vi "MainKinetics.vi"() -> ()   [LabVIEW 2017]
uses:
  <vilib>/Utility/miscctls.llb/LVRowAndColumnTypeDef.ctl
  <vilib>/Utility/sysdir.llb/System Directory Type.ctl
  <vilib>/Utility/config.llb/Read Key (String).vi
  <vilib>/Utility/config.llb/Write Key (String).vi
  <vilib>/Utility/cursorutil.llb/Set Cursor (Icon Pict).vi
  PCAN_Driver/ControlCAN.lvlib
  <vilib>/Utility/config.llb/NI_LVConfig.lvlib
panel:
  out "Offset":dbl
  out "Analogtest":bool=TRUE
  out "TestinExecution":string
  out "FullSpeed2 Current":dbl
  out "FullSpeed1 Current":dbl
  out "String":string
  out "ParamVersion":string
  out "DSP Board S/N":string
  out "POWER Board S/N":string caption="DRIVER Board S/N"
  in  "EventTimeout":i32=100
  out "SpeedLimit":dbl[](array[numeric])
  out "TestArray":string[](array[string])
  out "Motor Speed RPM Serial":dbl
  out "DAQmx Device Name":tag
  out "PN":string
  out "FileName":string
  out "VenableSpeed":u16
  out "TesterVersion":string
  out "ClosePanel":bool=TRUE
  out "UUT SN Report":string
  out "Automation":bool
  out "Test Failed":bool
  out "VisualInspectionResult":bool
  out "MotorTempResult":bool
  out "VenableDirectionResult":bool
  out "VenableResult":bool
  out "ComTestResult":bool=TRUE
  out "UUT SoftwareVer":string
  out "Next SN":i32
  in  "SetSN":bool
  out "Current SN":i32
  out "FullSpeed2 Speed":dbl
  out "FullSpeed2 Current":dbl
  out "FullSpeed1 Current":dbl
  out "FullSpeed1 Speed":dbl
  out "UUT":u8
  out "CAN Status":bool
  out "Array":u64[][](array[numeric]) format="%016x"
  out "Motor Phase Current RMS":dbl
  out "Ambient Temperature":dbl
  out "Speed error":bool
  out "Commutation err":bool
  out "Under voltage/Over voltage":bool
  out "Derated drive temp":bool
  out "Motor Over temperature":bool
  out "Motor Sensor temp Fauilre":bool
  out "Drive Over temperature":bool
  out "Drive Sensor temp Failure":bool
  out "Ambient Over temp":bool
  out "Ambient Sensor temp":bool
  out "DC Voltage":dbl
  out "DC Current":dbl
  out "Power transistor Heat sink Temp.":dbl
  out "Motor Stator Temp.":dbl
  out "Motor Speed RPM":dbl
  out "ECS State":u16
  out "UUT":string="EBAY"
  in  "Logger Path":path
  in  "Report":bool
  in  "Start":bool
  in  "ATR":string[][](table)=[["Test Communication", "-", "-", "-", "-", ""], ["Set S/N", "-", "-", "-", "-", ""], ["Set Board Number", "-", "-", "-", "-", ""], [" ", "", "", "", "", ""], ["Test Communication", "-", "-", "-", "-", ""], ["Get S/N", "-", "-", "-", "", ""], ["Get Board Number", "-", "-", "-", "", ""], ["Get FW", "-", "-", "-", "", ""], ["Enable Motor", "", "", "", "", ""], ["Small position command", "", "", "", "", ""], ["Measure delta", "", "", "", "", ""], ["Velocity command", "", "", "", "", ""]]
  in  "Settings":bool
  in  "Refresh Button":bool
  out "Serial Status":bool
  in  "VISA Kinetics":refnum<visa-resource-name>="COM6"
  in  "Serial Com":bool
  in  "Help Button":bool
  out "Pannel User Message":string
  in  "Stop Button":bool
  # "Kinetics"
  # "REDLER TECHNOLOGIES LTD"
  # "ver 1.2p"
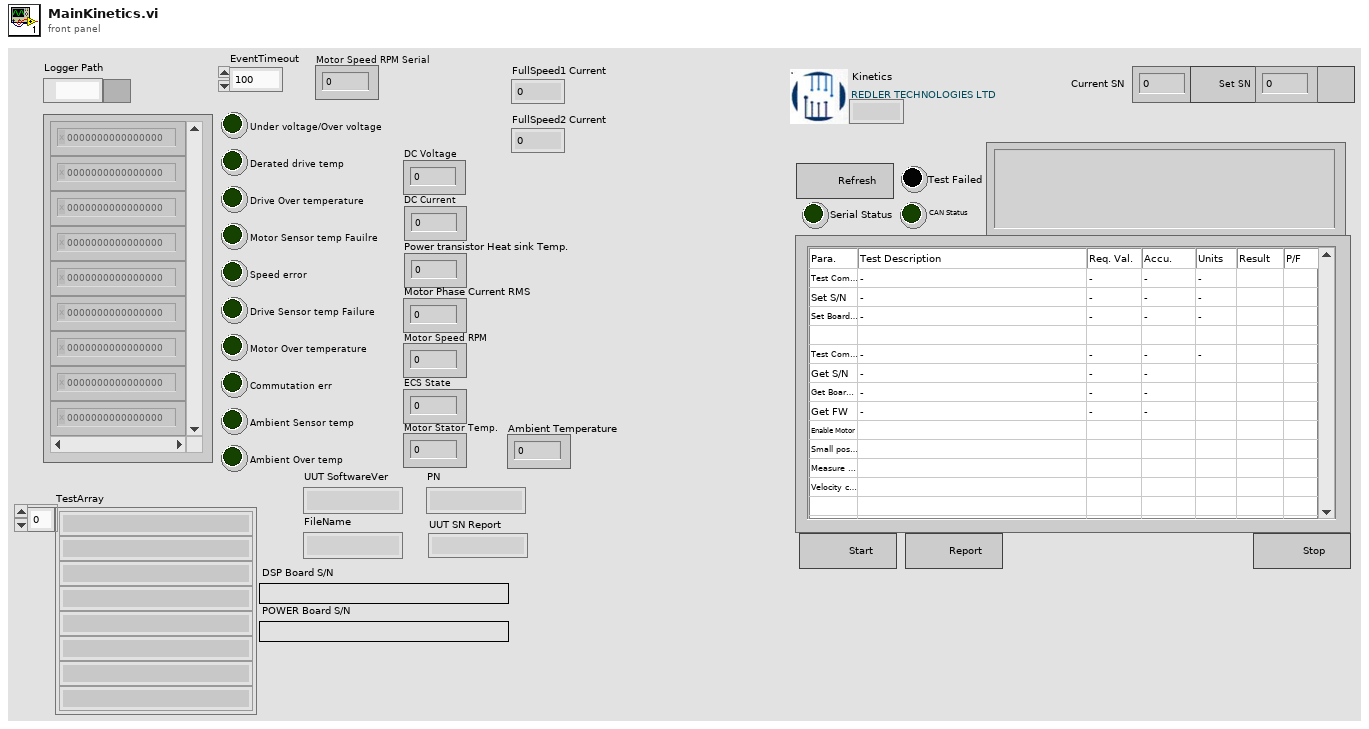
[diagram p1: front panel]
types:
  T1 = cluster{"VISA":refnum<visa-resource-name>, "TestArray":string[]}
  T2 = cluster{"ID":u32, "MSGTYPE":u8, "LEN":u8, "aDATA":u8[]}[]
  T3 = enum16{"Erase ATR Table", "Stop", "MainProgram", "Initialize"}
  T4 = typedef "NI_LVConfig.lvlib/Config Data RefNum.ctl" = refnum<k1>
  T5 = enum16{"Init", "0 ohm", "6 ohm", "13.2 ohm", "15 ohm", "25.9 ohm", "33 ohm", "Down", "Up", "Venable", "Firmware", "PowerSuply"}
  T6 = enum16{"Wait", "Exit", "VC=0", "ReadVC", "VC=1000"}
  T7 = enum16{"Stop", "Result", "FullSpeed2", "MD[1]=1", "FullSpeed1", "MD[1]=0"}
  T8 = enum16{"K15", "K16", "K17", "Venable", "Firmeware", "Fan", "Power", "120C", "110C", "100C", "90C", "80C", "70C", "60C", "50C", "40C", "30C", "25C", "20C", "10C", "0C"}
  T9 = enum8{"Term1", "Term2", "Current", "Fan", "TempCPU"}
  T10 = enum16{"Exit", "AI0/3", "AO0", "Wait", "Read", "Init"}
  T11 = enum16{"Exit", "Wait", "ReadCurrent", "ReadTemp", "Init"}
  T12 = enum16{"Init", "0 ohm", "6 ohm", "13.2 ohm", "15 ohm", "25.9 ohm", "33 ohm", "Down", "Up", "Venable", "Firmware", "PowerSuply"}[]
  T13 = enum8{"Enabled", "Disabled", "Disabled and Grayed Out"}
  T14 = typedef "LVRowAndColumnTypeDef.ctl" = cluster{"Row":i32, "Column":i32}
  T15 = enum32{"Invalid", "Standard", "Closed", "Hidden", "Minimized", "Maximized"}
  T16 = cluster{"ID":u32, "MSGTYPE":u8, "LEN":u8, "aDATA":u8[]}
  T17 = enum16{"open", "replace", "create", "open or create", "replace or create", "replace or create with confirmation"}
  T18 = typedef "ControlCAN.lvlib/DevType.ctl" = u32
  T19 = typedef "ControlCAN.lvlib/CAN Channel.ctl" = u32
  T20 = typedef "ControlCAN.lvlib/VCI_INIT_CONFIG.ctl" = cluster{"AccCode":u32, "AccMask":u32, "InitFlag":T21, "Fliter":T22, "Timing0":u8, "Timing1":u8, "Mode":T23}
  T21 = typedef "ControlCAN.lvlib/InitFlag.ctl" = u32
  T22 = typedef "ControlCAN.lvlib/Fliter.ctl" = u8
  T23 = typedef "ControlCAN.lvlib/Mode.ctl" = u8
  T24 = cluster{"DevType":T18, "DevIndex":u32, "CanIndex":T19, "VCI_INIT_CONFIG":T20}
  T25 = typedef "ControlCAN.lvlib/VCI_CAN_OBJ.ctl" = cluster{"ID":u32, "TimeStamp":u32, "TimeFlag":u8, "SendType":u8, "RemoteFlag":u8, "ExternFlag":u8, "DataLen":u8, "Data":u8[], "Reserved":u8[]}
  T26 = cluster{"Type":enum16{"接收", "发送"}, "Channel":T19, "Time":timestamp, "VCI_CAN_OBJ":T25}[]
  T27 = cluster{"Type":enum16{"接收", "发送"}, "Channel":T19, "Time":timestamp, "VCI_CAN_OBJ":T25}
  T28 = typedef "LVPoint32TypeDef.ctl" = cluster{"Horizontal":i32, "Vertical":i32}
  T29 = typedef "System Directory Type.ctl" = i32
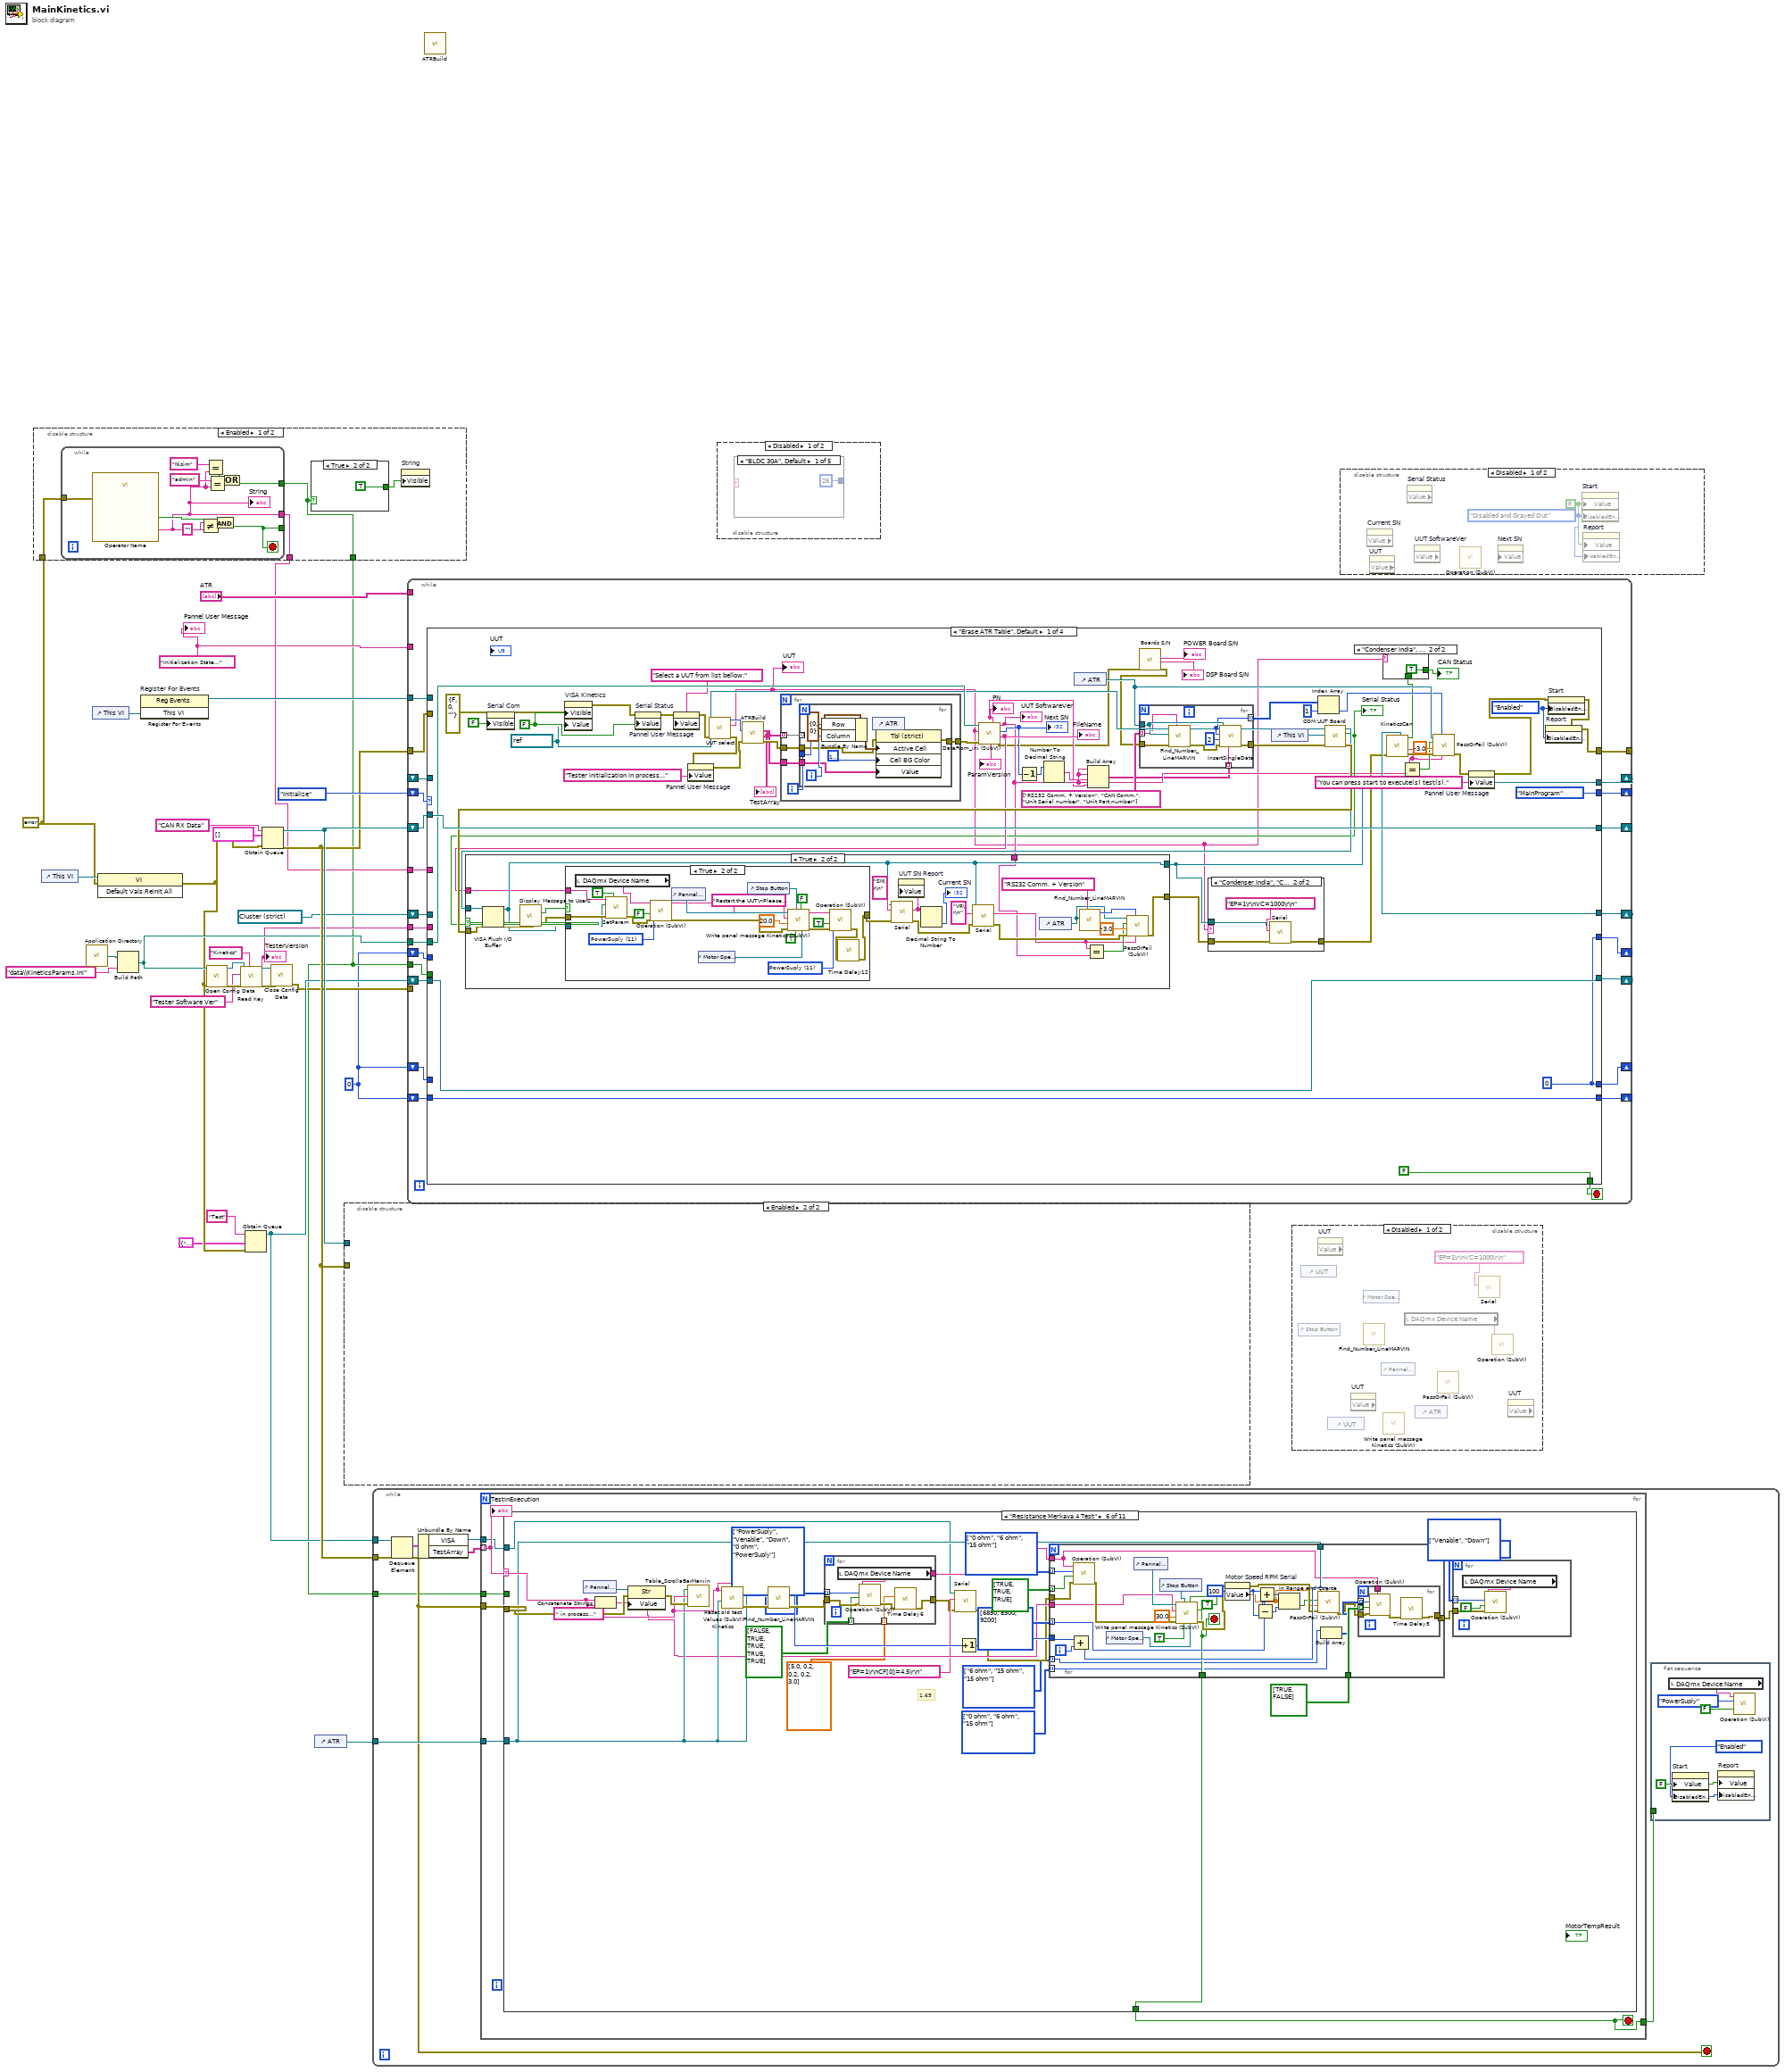
[diagram p0: block diagram]
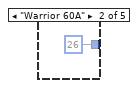
[diagram p2: hidden frame]
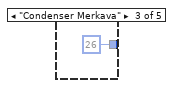
[diagram p3: hidden frame]
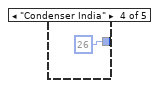
[diagram p4: hidden frame]
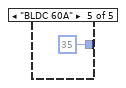
[diagram p5: hidden frame]
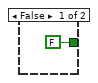
[diagram p7: hidden frame]
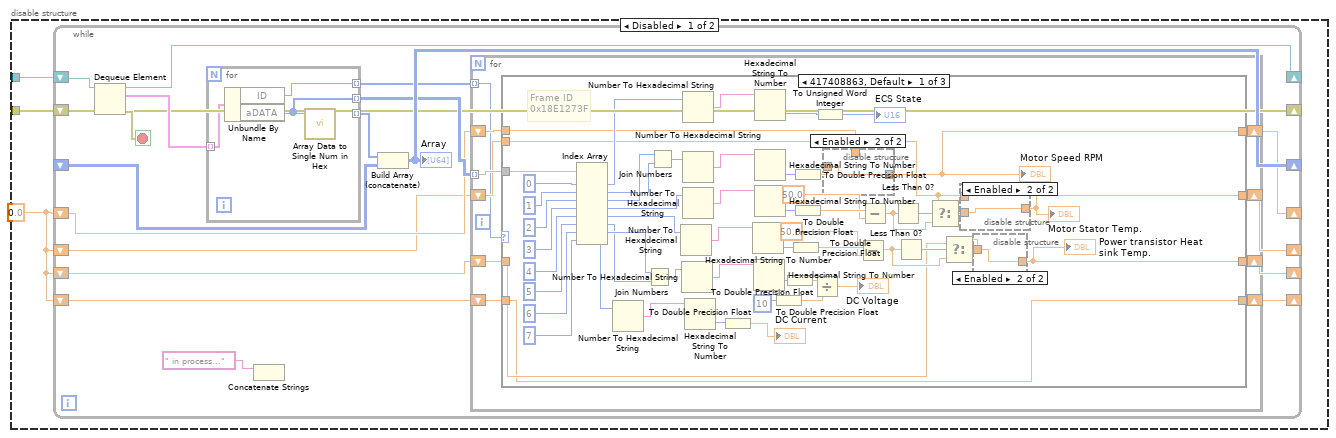
[diagram p9: hidden frame]
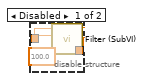
[diagram p10: hidden frame]
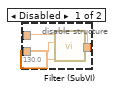
[diagram p11: hidden frame]
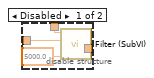
[diagram p12: hidden frame]
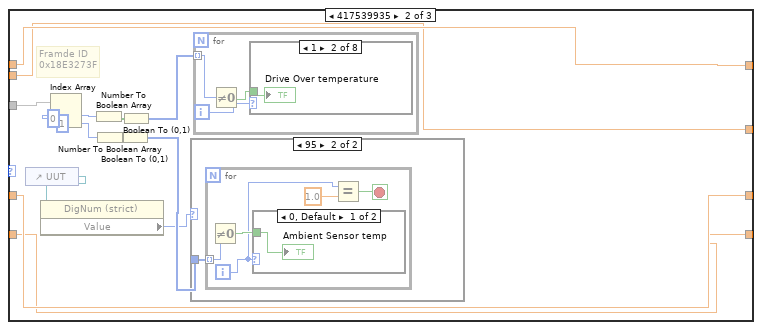
[diagram p13: hidden frame]
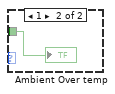
[diagram p15: hidden frame]
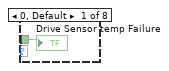
[diagram p16: hidden frame]
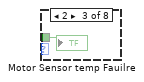
[diagram p17: hidden frame]
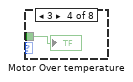
[diagram p18: hidden frame]
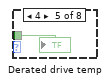
[diagram p19: hidden frame]
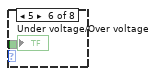
[diagram p20: hidden frame]
diagram:
  w17 = "Initialization State..."
  w2 = 0
  w5 = errorcluster {"status"=FALSE, "code"=0, "source"=""} ("error in (no error)")
  n1 = disable-structure shown="Enabled" {
    disable-tunnel: [w35 _] -> w18
    disable-tunnel: w5 -> [w33 _]
    disable-tunnel: [w32 _] -> w3
    frame Enabled {
      n2 = while {
        tunnel: [w45] -> _
        tunnel: [w38] -> w35
        tunnel: [w42] -> w32
        tunnel: w33 -> [w39]
        stop <- w45 stop-if-true
        n3 = call "Operator Name"("error in (no error)"=w39) -> ("Operator Name"=w38:string, "OK"=w46:bool)  [unwired: 16 in, 1 out]
        "String" <- w38
        n4 = Not Equal?(x=w38, y="") -> (x != y?=w47:bool)
        n5 = Equal?(x="Nisim", y=w38) -> (x = y?=w40:bool)
        n6 = Equal?(x="admin", y=w38) -> (x = y?=w43:bool)
        n7 = And(x=w46, y=w47) -> (x .and. y?=w45:bool)
        n8 = Or(x=w40, y=w43) -> (x .or. y?=w42:bool)
      }
      n9 = case shown="True" w32 {
        tunnel: [FALSE TRUE] -> w34
        frame False {
        }
        frame True {
        }
      }
      n10 = property on="String" class="Str"("Visible"=w34) -> ()  [unwired: 2 in, 2 out]
    }
    frame Disabled {
    }
  }
  n11 = control-ref of="This VI"() -> (w6:refnum<vi>)
  n12 = call <vilib>:"Application Directory.vi"() -> ("Application Directory"=w22:path)
  n13 = control-ref of="This VI"() -> (w20:refnum<vi>)
  n14 = invoke class="VI" method="Default Vals.Reinit All"(reference=w6, error in=w5) -> (error out=w4:errorcluster)  [unwired: 1 in, 2 out]
  n15 = Build Path(base path=w22, name or relative path="data\\KineticsParams.ini") -> (appended path=w9:path)
  n16 = register-events "Register For Events"(w20) -> (reference out=w19:refnum<event-registration>)  [unwired: 2 in, 1 out]
  n17 = call <vilib>:"Open Config Data.vi"("error in (no error)"=w4, "configuration file path"=w9) -> ("error out"=w15:errorcluster, "refnum"=w14:T4)  [unwired: 1 in, 7 out]
  n18 = call-poly <vilib>:"Read Key.vi"("section"="Kinetics", "error in (no error)"=w15, "key"="Tester Software Ver", "refnum"=w14) -> ("error out"=w12:errorcluster, "value"=w7:string, "refnum out"=w11:T4)  [unwired: 2 in, 3 out]
  "TesterVersion" <- w7
  n19 = Obtain Queue(name (unnamed)="Test", element data type=T1 {"VISA"="COM1", "TestArray"=[]}, error in (no error)=w4) -> (queue out=w25:refnum<queue>)  [unwired: 2 in, 2 out]
  n20 = Obtain Queue(name (unnamed)="CAN RX Data", element data type=T2 [], error in (no error)=w4) -> (queue out=w28:refnum<queue>, error out=w26:errorcluster)  [unwired: 2 in, 1 out]
  n21 = call <vilib>:"Close Config Data.vi"("error in (no error)"=w12, "refnum"=w11) -> ("error out"=w10:errorcluster)  [unwired: 8 in, 1 out]
  n22 = control-ref of="ATR"() -> (w16:refnum<vi>)
  n23 = disable-structure shown="Enabled" {
    disable-tunnel: w28 -> [w51 _]
    disable-tunnel: w26 -> [w50 _]
    frame Disabled {
      w49 = 0.0
      n24 = while {
        shift-right: [w68] -> _
        shift-left: w51 -> [w70]
        shift-right: [w66] -> _
        shift-left: _ -> [w67]
        shift-right: [w62] -> _
        shift-left: w50 -> [w62]
        shift-right: [w60] -> _
        shift-left: w49 -> [w61]
        shift-right: [w59] -> _
        shift-left: w49 -> [w58]
        shift-right: [w57] -> _
        shift-left: w49 -> [w56]
        shift-right: [w55] -> _
        shift-left: w49 -> [w54]
        stop <- w69 stop-if-true
        n25 = Dequeue Element(queue=w70, error in (no error)=w62) -> (queue out=w68:refnum<queue>, element=w63:T2, error out=w69:errorcluster)  [unwired: 1 in, 1 out]
        n26 = for {
          tunnel: [w216] -> w65 mode=indexing
          tunnel: w63 -> [w215] mode=indexing
          tunnel: [w214] -> w64 mode=indexing
          tunnel: [w213] -> w53 mode=indexing
          n27 = Unbundle By Name(w215) -> ("ID"=w213:u32, "aDATA"=w214:u8[])
          n28 = call "Array Data to Single Num in Hex.vi"("aDATA"=w214) -> ("Numeric"=w216:u64)  [unwired: 10 in]
        }
        n29 = Concatenate Strings(" in process..." ("Strin")) -> ()  [unwired: 1 in, 1 out]
        n30 = Build Array (concatenate)(w65, w67) -> (w66:u64[][])
        "Array" <- w66
        n31 = for {
          tunnel: w64 -> [w80] mode=indexing
          shift-right: [w78] -> w60
          shift-left: w61 -> [w79]
          shift-right: [w77] -> w59
          shift-left: w58 -> [w76]
          shift-right: [w75] -> w57
          shift-left: w56 -> [w74]
          shift-right: [w73] -> w55
          shift-left: w54 -> [w72]
          tunnel: w53 -> [w71] mode=indexing
          n32 = case shown="417408863, Default" w71 {
            tunnel: w80 -> [w117 w165 w203]
            tunnel: w79 -> [w91 w154 w192]
            tunnel: [w90 w154 w192] -> w78
            tunnel: [w87 w153 w191] -> w77
            tunnel: w76 -> [w86 w153 w191]
            tunnel: [w83 w152 w190] -> w75
            tunnel: w74 -> [w82 w152 w190]
            tunnel: [w81 w151 w186] -> w73
            tunnel: w72 -> [w81 w151 w185]
            frame 417408863, Default {
              # "Frame ID\n0x18E1273F"
              n33 = Index Array(array=w117, index #1=0 ("index"), index #2=1 ("index"), index #3=2 ("index"), index #4=3 ("index"), index #5=4 ("index"), index #6=5 ("index"), index #7=6 ("index"), index #8=7 ("index")) -> (element #1=w101:u8, element #2=w103:u8, element #3=w104:u8, element #4=w108:u8, element #5=w111:u8, element #6=w115:u8, element #7=w116:u8, element #8=w114:u8)
              n34 = Number To Hexadecimal String(2:w114) -> (0:w128:string)  [unwired: 1 in]
              n35 = Join Numbers(hi=w116, lo=w115) -> ((hi.lo)=w135:u16)
              n36 = Join Numbers(hi=w104, lo=w103) -> ((hi.lo)=w105:u16)
              n37 = Number To Hexadecimal String(2:w111) -> (0:w112:string)  [unwired: 1 in]
              n38 = Number To Hexadecimal String(2:w135) -> (0:w134:string)  [unwired: 1 in]
              n39 = Number To Hexadecimal String(2:w101) -> (0:w102:string)  [unwired: 1 in]
              n40 = Number To Hexadecimal String(2:w105) -> (0:w106:string)  [unwired: 1 in]
              n41 = Number To Hexadecimal String(2:w108) -> (0:w109:string)  [unwired: 1 in]
              n42 = Hexadecimal String To Number(string=w128) -> (number=w127:u32)  [unwired: 2 in, 1 out]
              n43 = To Double Precision Float(number=w127) -> (double precision float=→"DC Current":dbl)
              n44 = Hexadecimal String To Number(string=w112) -> (number=w113:u32)  [unwired: 2 in, 1 out]
              n45 = Hexadecimal String To Number(string=w134) -> (number=w133:u32)  [unwired: 2 in, 1 out]
              n46 = Hexadecimal String To Number(string=w102) -> (number=w99:u32)  [unwired: 2 in, 1 out]
              n47 = Hexadecimal String To Number(string=w106) -> (number=w107:u32)  [unwired: 2 in, 1 out]
              n48 = Hexadecimal String To Number(string=w109) -> (number=w110:u32)  [unwired: 2 in, 1 out]
              n49 = To Double Precision Float(number=u32 10 ("y")) -> (double precision float=w131:dbl)
              n50 = To Double Precision Float(number=w133) -> (double precision float=w130:dbl)
              n51 = To Double Precision Float(number=w113) -> (double precision float=w96:dbl)
              n52 = To Double Precision Float(number=w107) -> (double precision float=w92:dbl)
              n53 = To Double Precision Float(number=w110) -> (double precision float=w98:dbl)
              n54 = Divide(x=w130, y=w131) -> (x/y=→"DC Voltage":dbl)
              n55 = To Unsigned Word Integer(number=w99) -> (unsigned 16bit integer=→"ECS State":u16)
              n56 = disable-structure shown="Enabled" {
                disable-tunnel: w92 -> [w149 w150]
                disable-tunnel: w91 -> [w148 _]
                disable-tunnel: [w146 w150] -> w90
                frame Disabled {
                  n57 = call "Filter (SubVI).vi"("Delta"=5000.0, "NewVal"=w149, "OldVal"=w148) -> ("Val"=w146:dbl)  [unwired: 8 in]
                }
                frame Enabled {
                }
              }
              "Motor Speed RPM" <- w90
              n58 = Subtract(x=w96, y=50.0 ("x")) -> (x-y=w85:dbl)
              n59 = Subtract(x=w98, y=50.0 ("x")) -> (x-y=w88:dbl)
              n60 = Less Than 0?(x=w88) -> (x < 0?=w94:bool)
              n61 = Less Than 0?(x=w85) -> (x < 0?=w93:bool)
              n62 = Select(t=w86, s=w94, f=w88) -> (s? t:f=w89:dbl)
              n63 = Select(t=w82, s=w93, f=w85) -> (s? t:f=w84:dbl)
              n64 = disable-structure shown="Enabled" {
                disable-tunnel: w89 -> [w144 w145]
                disable-tunnel: [w143 w145] -> w87
                disable-tunnel: w86 -> [w142 _]
                frame Disabled {
                  n65 = call "Filter (SubVI).vi"("Delta"=130.0, "NewVal"=w144, "OldVal"=w142) -> ("Val"=w143:dbl)  [unwired: 8 in]
                }
                frame Enabled {
                }
              }
              "Motor Stator Temp." <- w87
              n66 = disable-structure shown="Enabled" {
                disable-tunnel: w84 -> [w139 w140]
                disable-tunnel: [w137 w140] -> w83
                disable-tunnel: w82 -> [w136 _]
                frame Disabled {
                  n67 = call "Filter (SubVI).vi"("Delta"=100.0, "NewVal"=w139, "OldVal"=w136) -> ("Val"=w137:dbl)  [unwired: 8 in]
                }
                frame Enabled {
                }
              }
              "Power transistor Heat sink Temp." <- w83
            }
            frame 417539935 {
              # "Framde ID\n0x18E3273F"
              n68 = control-ref of="UUT"() -> (w155:refnum<vi>)
              n69 = property on="Property Node" class="DigNum (strict)"(reference=w155) -> ("Value"=w156:u8)  [unwired: 1 in, 2 out]
              n70 = Index Array(array=w165, index #1=0 ("index"), index #2=1 ("index")) -> (element #1=w163:u8, element #2=w158:u8)
              n71 = Number To Boolean Array(number=w163) -> (Boolean array=w162:bool[])
              n72 = Number To Boolean Array(number=w158) -> (Boolean array=w160:bool[])
              n73 = Boolean To (0,1)(Boolean=w160) -> (0, 1=w157:i16[])
              n74 = Boolean To (0,1)(Boolean=w162) -> (0, 1=w161:i16[])
              n75 = case shown="95" w156 {
                tunnel: w157 -> [_ w166]
                frame 0, Default {
                }
                frame 95 {
                  n76 = for {
                    tunnel: w166 -> [w171] mode=indexing
                    i -> [w167]
                    stop <- w169 stop-if-true
                    n77 = Not Equal To 0?(x=w171) -> (x != 0?=w170:bool)
                    n78 = case shown="0, Default" w167 {
                      tunnel: w170 -> [w172 w173]
                      frame 0, Default {
                        "Ambient Sensor temp" <- w172
                      }
                      frame 1 {
                        "Ambient Over temp" <- w173
                      }
                    }
                    n79 = Equal?(x=w167, y=1.0) -> (x = y?=w169:bool)
                  }
                }
              }
              n80 = for {
                tunnel: w161 -> [w175] mode=indexing
                i -> [w176]
                n81 = Not Equal To 0?(x=w175) -> (x != 0?=w174:bool)
                n82 = case shown="1" w176 {
                  tunnel: w174 -> [w177 w178 w179 w180 w181 w182 w183 w184]
                  frame 0, Default {
                    "Drive Sensor temp Failure" <- w177
                  }
                  frame 1 {
                    "Drive Over temperature" <- w178
                  }
                  frame 2 {
                    "Motor Sensor temp Fauilre" <- w179
                  }
                  frame 3 {
                    "Motor Over temperature" <- w180
                  }
                  frame 4 {
                    "Derated drive temp" <- w181
                  }
                  frame 5 {
                    "Under voltage/Over voltage" <- w182
                  }
                  frame 6 {
                    "Commutation err" <- w183
                  }
                  frame 7 {
                    "Speed error" <- w184
                  }
                }
              }
            }
            frame 417474399 {
              # "Frame ID\n0x18E2273F"
              n83 = Index Array(array=w203, index #1=0 ("index"), index #2=1 ("index")) -> (element #1=w200:u8, element #2=w197:u8)
              n84 = disable-structure shown="Enabled" {
                disable-tunnel: [w211 w212] -> w201
                disable-tunnel: w200 -> [w210 w212]
                frame Disabled {
                  n85 = Number To Hexadecimal String(2:w210) -> (0:w209:string)  [unwired: 1 in]
                  n86 = Hexadecimal String To Number(string=w209) -> (number=w211:u32)  [unwired: 2 in, 1 out]
                }
                frame Enabled {
                }
              }
              n87 = Number To Hexadecimal String(2:w197) -> (0:w195:string)  [unwired: 1 in]
              n88 = Hexadecimal String To Number(string=w195) -> (number=w196:u32)  [unwired: 2 in, 1 out]
              n89 = To Double Precision Float(number=w196) -> (double precision float=w194:dbl)
              n90 = To Double Precision Float(number=w201) -> (double precision float=→"Motor Phase Current RMS":dbl)
              n91 = Subtract(x=w194, y=50.0) -> (x-y=w188:dbl)
              n92 = Less Than 0?(x=w188) -> (x < 0?=w189:bool)
              n93 = Select(t=w185, s=w189, f=w188) -> (s? t:f=w187:dbl)
              n94 = disable-structure shown="Disabled" {
                disable-tunnel: w187 -> [w207 w208]
                disable-tunnel: [w205 w208] -> w186
                disable-tunnel: w185 -> [w204 _]
                frame Disabled {
                  n95 = call "Filter (SubVI).vi"("Delta"=65.0, "NewVal"=w207, "OldVal"=w204) -> ("Val"=w205:dbl)  [unwired: 8 in]
                }
                frame Enabled {
                }
              }
              "Ambient Temperature" <- w186
            }
          }
        }
      }
    }
    frame Enabled {
    }
  }
  n96 = while {
    tunnel: w16 -> [w225]
    tunnel: w26 -> [w223]
    tunnel: w25 -> [w224]
    tunnel: w3 -> [w218]
    stop <- w220 stop-if-true
    n97 = Dequeue Element(queue=w224, error in (no error)=w223) -> (element=w222:T1, error out=w220:errorcluster)  [unwired: 1 in, 2 out]
    n98 = Unbundle By Name(w222) -> ("VISA"=w221:refnum<visa-resource-name>, "TestArray"=w217:string[])
    n99 = for {
      tunnel: w217 -> [w235] mode=indexing
      tunnel: w221 -> [w233]
      tunnel: w225 -> [w232]
      tunnel: w220 -> [w236]
      tunnel: [w231] -> w219
      tunnel: w218 -> [w234]
      stop <- w231 stop-if-true
      n100 = case shown="\"Resistance Merkava 4 Test\"" w235 {
        selector: w235 -> [_ w254 w659 w1120 w1247 w1391 w1467 w1542 w1628 w1789 w1907]
        tunnel: w232 -> [_ w247 _ _ w1240 w1384 w1460 w1535 w1629 w1797 w1905]
        tunnel: w236 -> [_ w257 _ _ w1255 w1390 w1466 w1541 w1630 w1804 w1909]
        tunnel: w234 -> [_ _ _ _ _ _ _ _ _ _ _]
        tunnel: w233 -> [_ w250 w658 w1119 w1243 w1376 w1456 w1524 w1606 w1790 w1906]
        tunnel: [TRUE ("Stopped") w242 w657 w1109 w1236 w1371 w1447 w1526 w1620 w1788 FALSE ("Stopped")] -> w231
        frame "", Default {
        }
        frame "Comm. & Motor Test" {
          n101 = control-ref of="Pannel User Message"() -> (w258:refnum<vi>)
          n102 = Concatenate Strings(w254, " in process..." ("string")) -> (w249:string)
          n103 = property class="Str"(reference=w258, error in=w257, "Value"=w249) -> (error out=w256:errorcluster)  [unwired: 1 out]
          n104 = call "Table_ScrollaBarMarvin.vi"("error in"=w256, "Line to focus"=w254, "reference in"=w247) -> ("error out"=w253:errorcluster)  [unwired: 2 out]
          n105 = property on="UUT" class="Str"() -> ("Value"=w246:string)  [unwired: 2 in, 2 out]
          n106 = call "Find_Number_LineMARVIN.vi"("Test Paragraph"=w254, "error in"=w253, "TableIn"=w247) -> ("error out"=w259:errorcluster, "Line number"=w238:i32)  [unwired: 2 in, 2 out]
          n107 = Concatenate Strings("- Set the FIREWERE switch to OFF position." ("Screen Line"), "- Set the VENABLE switch to ON position." ("Screen Line")) -> (w243:string)
          n108 = call <vilib>:"Clear Errors.vi"("error in (no error)"=w259) -> ("error out"=w252:errorcluster)  [unwired: 5 in, 1 out]
          n109 = Add(x=3, y=w238) -> (x+y=w248:i32)
          n110 = call "Reset old test Values (SubVI) Kinetics.vi"("error in"=w252, "Atr in"=w247, "Test Paragraph"=w254) -> ("error out"=w241:errorcluster)  [unwired: 6 in, 2 out]
          n111 = case shown="\"Condenser India\", \"Condenser Merkava\"" w246 {
            tunnel: w243 -> [_ w656]
            tunnel: w241 -> [w654 w655]
            tunnel: [w654 w655] -> w240
            frame "False", Default {
            }
            frame "Condenser India", "Condenser Merkava" {
              n112 = One Button Dialog(message=w656) -> ()  [unwired: 1 in, 1 out]
            }
          }
          n113 = for {
            N: 2 -> [_]
            tunnel: w250 -> [w267]
            tunnel: w249 -> [w266]
            tunnel: w248 -> [w265]
            tunnel: w247 -> [w264]
            tunnel: [w263] -> w242
            tunnel: w240 -> [w262]
            tunnel: w238 -> [w260]
            i -> [w261]
            n114 = case shown="1" w261 {
              tunnel: w267 -> [w285 w376]
              tunnel: w266 -> [w284 w375]
              tunnel: w265 -> [w282 _]
              tunnel: w264 -> [w275 w373]
              tunnel: [w280 w377] -> w263
              tunnel: w262 -> [w271 _]
              tunnel: w260 -> [w277 _]
              frame 0, Default {
                n115 = Increment(x=w277) -> (x+1=w270:i32)
                n116 = property on="Serial Status" class="Bool (strict)"() -> ("Value"=w279:bool)  [unwired: 2 in, 2 out]
                n117 = property on="UUT SoftwareVer" class="Str"() -> ("Value"=w268:string)  [unwired: 2 in, 2 out]
                n118 = call "PassOrFail (SubVI).vi"("String Res"=w268, "index (row)"=w270, "error in (no error)"=w271, "Data in"=-3.0, "Pass?Fail"=w279, "Table in"=w275) -> ("error out"=w273:errorcluster)  [unwired: 5 in]
                n119 = Increment(x=w270) -> (x+1=w269:i32)
                n120 = property on="CAN Status" class="Bool (strict)"() -> ("Value"=w274:bool)  [unwired: 2 in, 2 out]
                n121 = call "PassOrFail (SubVI).vi"("String Res"=w268, "index (row)"=w269, "error in (no error)"=w273, "Data in"=-3.0, "Pass?Fail"=w274, "Table in"=w275) -> ("error out"=w272:errorcluster)  [unwired: 5 in]
                n122 = while {
                  shift-right: [w296] -> _
                  shift-left: T6."VC=1000" -> [w299]
                  tunnel: w272 -> [w298]
                  tunnel: w285 -> [w297]
                  tunnel: w284 -> [w295]
                  shift-right: [w292] -> w281
                  shift-left: bool[] [FALSE, FALSE] -> [w293]
                  tunnel: w282 -> [w291]
                  tunnel: w275 -> [w290]
                  tunnel: [w288] -> w280
                  i -> [w294]
                  stop <- w289 stop-if-true
                  n123 = case shown="\"VC=0\"" w299 {
                    tunnel: w298 -> [_ w322 _ w353 _]
                    tunnel: w297 -> [w302 w320 w329 w357 _]
                    tunnel: [T6."Exit" T6."Wait" w326 T6."Wait" T6."ReadVC"] -> w296
                    tunnel: w295 -> [_ _ _ _ w365]
                    tunnel: [TRUE FALSE FALSE FALSE FALSE] -> w289
                    tunnel: w294 -> [_ _ w327 _ w360]
                    tunnel: w293 -> [w301 w317 w325 w355 w362]
                    tunnel: [w301 w317 w324 w355 w362] -> w292
                    tunnel: w291 -> [w310 _ _ _ _]
                    tunnel: w290 -> [w312 _ _ _ _]
                    tunnel: [_ _ _ _ w359] -> w288
                    frame "Exit", Default {
                      n124 = And Array Elements(Boolean array=w301) -> (logical AND=w305:bool)
                      n125 = local read "DAQmx Device Name"() -> (w309:tag)
                      n126 = Select(t="OK", s=w305, f="Failed") -> (s? t:f=w311:string)
                      n127 = call "PassOrFail (SubVI).vi"("String Res"=w311, "index (row)"=w310, "Data in"=-3.0, "Pass?Fail"=w305, "Table in"=w312) -> ("error out"=w300:errorcluster)  [unwired: 6 in]
                      n128 = call "Serial.vi"("error in (no error)"=w300, "write buffer"="EP=1\r\nVC=0\r\n", "VISA resource name"=w302) -> ("error out"=w303:errorcluster)  [unwired: 7 in, 1 out]
                      n129 = call "Operation (SubVI).vi"("error in (no error)"=w303, "On/Off"=FALSE, "Operation"=T5."Venable", "DAQmx Device Name"=w309) -> ()  [unwired: 7 in, 1 out]
                    }
                    frame "VC=0" {
                      n130 = call "Serial.vi"("error in (no error)"=w322, "write buffer"="EP=1\r\nVC=0\r\n", "VISA resource name"=w320) -> ()  [unwired: 7 in, 2 out]
                    }
                    frame "ReadVC" {
                      n131 = call "Serial.vi"("write buffer"="VC\r\n", "VISA resource name"=w329) -> ("read buffer"=w328:string)  [unwired: 8 in, 1 out]
                      n132 = case shown="5, Default" w327 {
                        tunnel: w328 -> [w338 w344]
                        tunnel: [T6."VC=0" T6."Exit"] -> w326
                        tunnel: w325 -> [w333 w343]
                        tunnel: [w331 w340] -> w324
                        frame 2 {
                          n133 = Decimal String To Number(string=w338) -> (number=w337:i32)  [unwired: 2 in, 1 out]
                          n134 = In Range and Coerce(upper limit=1100, x=w337, lower limit=900) -> (In Range?=w332:bool)  [unwired: 1 out]
                          n135 = Replace Array Subset(array=w333, new element=w332, index=0) -> (w331:bool[])
                        }
                        frame 5, Default {
                          n136 = Decimal String To Number(string=w344) -> (number=w347:i32)  [unwired: 2 in, 1 out]
                          n137 = In Range and Coerce(upper limit=100, x=w347, lower limit=0) -> (In Range?=w341:bool)  [unwired: 1 out]
                          n138 = Replace Array Subset(array=w343, new element=w341, index=1) -> (w340:bool[])
                        }
                      }
                    }
                    frame "VC=1000" {
                      n139 = local read "DAQmx Device Name"() -> (w354:tag)
                      n140 = call "Operation (SubVI).vi"("error in (no error)"=w353, "On/Off"=TRUE, "Operation"=T5."Venable", "DAQmx Device Name"=w354) -> ("error out"=w352:errorcluster)  [unwired: 7 in]
                      n141 = call "Serial.vi"("error in (no error)"=w352, "write buffer"="EP=1\r\nVC=1000\r\n", "VISA resource name"=w357) -> ()  [unwired: 7 in, 2 out]
                    }
                    frame "Wait" {
                      n142 = case shown="4" w360 {
                        tunnel: [25.0 ("Time to wait") 15.0 ("Time to wait")] -> w366
                        frame 4 {
                        }
                        frame 1, Default {
                        }
                      }
                      n143 = control-ref of="Motor Speed RPM Serial"() -> (w370:refnum<vi>)
                      n144 = control-ref of="Pannel User Message"() -> (w369:refnum<vi>)
                      n145 = control-ref of="Stop Button"() -> (w364:refnum<vi>)
                      n146 = call "Write panel message Kinetics (SubVI).vi"(4:"rpm"=w370, 5:"rpm"=TRUE ("rpm"), "PrintTime"=TRUE, "Stop"=w364, "Time to wait"=w366, "Strin"=w365, "String in"=w369) -> ("Stopped"=w359:bool)  [unwired: 3 in, 1 out]
                    }
                  }
                }
                n147 = And Array Elements(Boolean array=w281) -> (logical AND=→"ComTestResult":bool)
              }
              frame 1 {
                n148 = case shown="False" FALSE {
                  tunnel: [_ w399] -> w377
                  tunnel: w376 -> [w378 w398]
                  tunnel: w375 -> [_ w396]
                  tunnel: w373 -> [w384 _]
                  frame False {
                    n149 = Two Button Dialog(message="Is the motor run in he right direction?", 1:"No" ("F button name (\"Cancel\")"), 2:"Yes" ("T button name (\"OK\")")) -> (T button?=w380:bool)
                    n150 = call "Find_Number_LineMARVIN.vi"("Test Paragraph"="Motor Direction", "TableIn"=w384) -> ("Line number"=w395:i32)  [unwired: 3 in, 3 out]
                    n151 = Select(t="OK", s=w380, f="Failed") -> (s? t:f=w394:string)
                    n152 = call "PassOrFail (SubVI).vi"("String Res"=w394, "index (row)"=w395, "Data in"=-3.0, "Pass?Fail"=w380, "Table in"=w384) -> ("error out"=w392:errorcluster)  [unwired: 6 in]
                    n153 = call "Serial.vi"("error in (no error)"=w392, "write buffer"="EP=1\r\nVC=0\r\n", "VISA resource name"=w378) -> ("error out"=w393:errorcluster)  [unwired: 7 in, 1 out]
                    n154 = local read "DAQmx Device Name"() -> (w379:tag)
                    n155 = call "Operation (SubVI).vi"("error in (no error)"=w393, "On/Off"=FALSE, "Operation"=T5."Venable", "DAQmx Device Name"=w379) -> ()  [unwired: 7 in, 1 out]
                  }
                  frame True {
                    n156 = property on="UUT" class="Str"() -> ("Value"=w401:string)  [unwired: 2 in, 2 out]
                    n157 = case shown="\"BLDC 60A\"" w401 {
                      tunnel: [26 26 26 26 47] -> w402
                      tunnel: [_ _ _ _ 56] -> w403
                      tunnel: [_ _ _ _ "10800"] -> w397
                      frame "BLDC 30A", Default {
                      }
                      frame "Warrior 60A" {
                      }
                      frame "Condenser Merkava" {
                      }
                      frame "Condenser India" {
                      }
                      frame "BLDC 60A" {
                      }
                    }
                    n158 = local read "DAQmx Device Name"() -> (w407:tag)
                    n159 = control-ref of="Stop Button"() -> (w404:refnum<vi>)
                    n160 = control-ref of="ATR"() -> (w408:refnum<vi>)
                    n161 = control-ref of="Pannel User Message"() -> (w405:refnum<vi>)
                    n162 = control-ref of="Motor Speed RPM Serial"() -> (w406:refnum<vi>)
                    n163 = while {
                      shift-right: [w421] -> _
                      shift-left: T7."MD[1]=0" -> [w422]
                      tunnel: w404 -> [w420]
                      tunnel: w405 -> [w419]
                      tunnel: w406 -> [w418]
                      tunnel: w407 -> [w417]
                      tunnel: w402 -> [w416]
                      tunnel: w403 -> [w415]
                      tunnel: w408 -> [w414]
                      tunnel: [w409] -> w399
                      tunnel: w398 -> [w412]
                      tunnel: w397 -> [w411]
                      tunnel: w396 -> [w410]
                      stop <- w413 stop-if-true
                      n164 = case shown="\"MD[1]=1\"" w422 {
                        tunnel: [T7."Stop" T7."Stop" w472 w546 w571 w646] -> w421
                        tunnel: [TRUE w433 FALSE FALSE FALSE FALSE] -> w413
                        tunnel: w420 -> [_ _ w457 w523 w555 w623]
                        tunnel: w419 -> [_ _ w458 w524 w556 w624]
                        tunnel: w418 -> [_ _ w459 w518 w558 w618]
                        tunnel: w417 -> [_ w428 w462 w510 w561 w610]
                        tunnel: w416 -> [_ _ _ _ w557 _]
                        tunnel: w415 -> [_ _ w456 _ _ _]
                        tunnel: w414 -> [_ w435 _ _ _ _]
                        tunnel: w412 -> [_ w427 w452 _ w553 w615]
                        tunnel: w411 -> [_ _ w451 _ w550 _]
                        tunnel: w410 -> [_ _ w449 w515 w548 w614]
                        tunnel: [_ _ w448 w506 w547 w605] -> w409
                        frame "Stop", Default {
                        }
                        frame "Result" {
                          n165 = property on="FullSpeed2 Current" class="DigNum (strict)"() -> ("Value"=w440:dbl)  [unwired: 2 in, 2 out]
                          n166 = property on="FullSpeed1 Current" class="DigNum (strict)"() -> ("Value"=w439:dbl)  [unwired: 2 in, 2 out]
                          n167 = Subtract(x=w440, y=w439) -> (x-y=w447:dbl)
                          n168 = Absolute Value(x=w447) -> (abs(x)=w442:dbl)
                          n169 = Greater Or Equal?(x=w442, y=u32 5) -> (x >= y?=w434:bool)
                          n170 = call "Find_Number_LineMARVIN.vi"("Test Paragraph"="Motor Direction", "TableIn"=w435) -> ("Line number"=w444:i32)  [unwired: 3 in, 3 out]
                          n171 = Select(t="OK", s=w434, f="Failed") -> (s? t:f=w436:string)
                          n172 = call "PassOrFail (SubVI).vi"("String Res"=w436, "index (row)"=w444, "Data in"=-3.0, "Pass?Fail"=w434, "Table in"=w435) -> ("error out"=w426:errorcluster)  [unwired: 6 in]
                          n173 = call "Serial.vi"("error in (no error)"=w426, "write buffer"="EP=1\r\nVC=0\r\n", "VISA resource name"=w427) -> ("error out"=w432:errorcluster)  [unwired: 7 in, 1 out]
                          n174 = Not(x=TRUE) -> (.not. x?=w433:bool)
                          n175 = call "Operation (SubVI).vi"("error in (no error)"=w432, "On/Off"=FALSE, "Operation"=T5."Venable", "DAQmx Device Name"=w428) -> ()  [unwired: 7 in, 1 out]
                        }
                        frame "FullSpeed2" {
                          n176 = Search and Replace String(input string="EP=1\r\nVC=0\r\n" ("write buffer"), search string="0", replace string=w451) -> (result string=w455:string)  [unwired: 5 in, 3 out]
                          n177 = call "Serial.vi"("write buffer"=w455, "VISA resource name"=w452) -> ("error out"=w450:errorcluster)  [unwired: 8 in, 1 out]
                          n178 = Concatenate Strings(w449, "\nFull speed operation " ("string")) -> (w466:string)
                          n179 = call "Write panel message Kinetics (SubVI).vi"(4:"rpm"=w459, 5:"rpm"=TRUE ("rpm"), "PrintTime"=FALSE, "Stop"=w457, "error in (no error)"=w450, "Time to wait"=0.2, "Strin"=w466, "String in"=w458) -> ("error out"=w469:errorcluster, "Stopped"=w461:bool)  [unwired: 2 in]
                          n180 = flat-sequence {
                            tunnel: w469 -> [w476]
                            tunnel: [w476] -> w468
                            tunnel: [w475] -> w467
                            frame #0 {
                              n181 = call <vilib>:"High Resolution Relative Seconds.vi"() -> ("relative seconds"=w475:dbl)
                            }
                          }
                          n182 = while {
                            tunnel: w468 -> [w488]
                            tunnel: [w498] -> _
                            tunnel: w456 -> [w504]
                            tunnel: w467 -> [w502]
                            tunnel: w466 -> [w496]
                            tunnel: w459 -> [w482]
                            tunnel: w462 -> [w490]
                            tunnel: w461 -> [w489]
                            tunnel: [w477] -> w460
                            tunnel: w458 -> [w487]
                            tunnel: w457 -> [w486]
                            tunnel: [w477] -> w448
                            stop <- w505 stop-if-true
                            n183 = call <vilib>:"High Resolution Relative Seconds.vi"() -> ("relative seconds"=w503:dbl)
                            n184 = property class="DigNum (strict)"(reference=w482) -> ("Value"=w481:dbl)  [unwired: 1 in, 2 out]
                            n185 = Subtract(x=w503, y=w502) -> (x-y=w501:dbl)
                            n186 = call "Aquire AI2"("error in"=w488, "device name"=w490) -> ("data"=w493:dynamicdata, "error out"=w492:errorcluster)  [unwired: 15 in, 1 out]
                            n187 = Greater Or Equal?(x=w501, y=120.0) -> (x >= y?=w499:bool)
                            n188 = To Double Precision Float(number=w493) -> (double precision float=w491:dbl)
                            "FullSpeed2 Current" <- w491
                            n189 = Multiply(x=w491, y=25.0) -> (x*y=w485:dbl)
                            n190 = Greater Or Equal?(x=w485, y=w504) -> (x >= y?=w483:bool)
                            n191 = Greater Or Equal?(x=w481, y=10000.0) -> (x >= y?=w478:bool)
                            n192 = And(x=w483, y=w478) -> (x .and. y?=w479:bool)
                            n193 = call "Write panel message Kinetics (SubVI).vi"(4:"rpm"=w482, 5:"rpm"=TRUE ("rpm"), "PrintTime"=FALSE, "Stop"=w486, "error in (no error)"=w492, "Time to wait"=0.2, "Strin"=w496, "String in"=w487) -> ("error out"=w498:errorcluster, "Stopped"=w477:bool)  [unwired: 2 in]
                            n194 = Compound Arithmetic op=OR(w477, w489, w499, w479) -> (w505:bool)
                          }
                          n195 = Select(t=T7."Stop", s=w460, f=T7."Result") -> (s? t:f=w472:T7)
                        }
                        frame "MD[1]=1" {
                          n196 = call "Operation (SubVI).vi"("On/Off"=FALSE, "Operation"=T5."Venable", "DAQmx Device Name"=w510) -> ("error out"=w533:errorcluster)  [unwired: 8 in]
                          n197 = Concatenate Strings(w515, "\nSet Parameters MD[1]=1" ("Strin")) -> (w525:string)
                          n198 = call "Write panel message Kinetics (SubVI).vi"(4:"rpm"=w518, 5:"rpm"=FALSE ("rpm"), "PrintTime"=FALSE, "Stop"=w523, "error in (no error)"=w533, "Time to wait"=30.0, "Strin"=w525, "String in"=w524) -> ("error out"=w532:errorcluster, "Stopped"=w507:bool)  [unwired: 2 in]
                          n199 = call "Serial.vi"("error in (no error)"=w532, "write buffer"="EP=1\r\nVC=0\r\nMD[1]=1\r\n") -> ("error out"=w529:errorcluster)  [unwired: 8 in, 1 out]
                          n200 = call "Operation (SubVI).vi"("error in (no error)"=w529, "On/Off"=FALSE, "Operation"=T5."PowerSuply", "DAQmx Device Name"=w510) -> ("error out"=w528:errorcluster)  [unwired: 7 in]
                          n201 = call "Write panel message Kinetics (SubVI).vi"(4:"rpm"=w518, 5:"rpm"=FALSE ("rpm"), "PrintTime"=TRUE, "Stop"=w523, "error in (no error)"=w528, "Time to wait"=25.0, "Strin"=w525, "String in"=w524) -> ("error out"=w511:errorcluster, "Stopped"=w508:bool)  [unwired: 2 in]
                          n202 = call "Operation (SubVI).vi"("error in (no error)"=w511, "On/Off"=TRUE, "Operation"=T5."PowerSuply", "DAQmx Device Name"=w510) -> ("error out"=w512:errorcluster)  [unwired: 7 in]
                          n203 = call "Operation (SubVI).vi"("error in (no error)"=w512, "On/Off"=TRUE, "Operation"=T5."Venable", "DAQmx Device Name"=w510) -> ("error out"=w520:errorcluster)  [unwired: 7 in]
                          n204 = call "Write panel message Kinetics (SubVI).vi"(4:"rpm"=w518, 5:"rpm"=FALSE ("rpm"), "PrintTime"=TRUE, "Stop"=w523, "error in (no error)"=w520, "Time to wait"=3.0, "Strin"=w525, "String in"=w524) -> ("Stopped"=w509:bool)  [unwired: 2 in, 1 out]
                          n205 = Compound Arithmetic op=OR(w509, w508, w507) -> (w506:bool)
                          n206 = Compound Arithmetic op=OR(w509, w508, w507) -> (w517:bool)
                          n207 = Select(t=T7."Stop", s=w517, f=T7."FullSpeed2") -> (s? t:f=w546:T7)
                        }
                        frame "FullSpeed1" {
                          n208 = Search and Replace String(input string="EP=1\r\nVC=0\r\n" ("write buffer"), search string="0", replace string=w550) -> (result string=w549:string)  [unwired: 5 in, 3 out]
                          n209 = call "Serial.vi"("write buffer"=w549, "VISA resource name"=w553) -> ("error out"=w554:errorcluster)  [unwired: 8 in, 1 out]
                          n210 = Concatenate Strings(w548, "\nFull speed operation " ("string")) -> (w565:string)
                          n211 = call "Write panel message Kinetics (SubVI).vi"(4:"rpm"=w558, 5:"rpm"=TRUE ("rpm"), "PrintTime"=FALSE, "Stop"=w555, "error in (no error)"=w554, "Time to wait"=0.2, "Strin"=w565, "String in"=w556) -> ("error out"=w568:errorcluster, "Stopped"=w560:bool)  [unwired: 2 in]
                          n212 = flat-sequence {
                            tunnel: w568 -> [w575]
                            tunnel: [w575] -> w567
                            tunnel: [w574] -> w566
                            frame #0 {
                              n213 = call <vilib>:"High Resolution Relative Seconds.vi"() -> ("relative seconds"=w574:dbl)
                            }
                          }
                          n214 = while {
                            tunnel: w567 -> [w587]
                            tunnel: [w597] -> _
                            tunnel: w557 -> [w603]
                            tunnel: w566 -> [w601]
                            tunnel: w565 -> [w595]
                            tunnel: w558 -> [w580]
                            tunnel: w561 -> [w589]
                            tunnel: w560 -> [w588]
                            tunnel: [w576] -> w559
                            tunnel: w556 -> [w586]
                            tunnel: w555 -> [w585]
                            tunnel: [w576] -> w547
                            stop <- w604 stop-if-true
                            n215 = call <vilib>:"High Resolution Relative Seconds.vi"() -> ("relative seconds"=w602:dbl)
                            n216 = property class="DigNum (strict)"(reference=w580) -> ("Value"=w579:dbl)  [unwired: 1 in, 2 out]
                            n217 = Subtract(x=w602, y=w601) -> (x-y=w600:dbl)
                            n218 = call "Aquire AI"("error in"=w587, "device name"=w589) -> ("data"=w592:dynamicdata, "error out"=w591:errorcluster)  [unwired: 15 in, 1 out]
                            n219 = Greater Or Equal?(x=w600, y=120.0) -> (x >= y?=w598:bool)
                            n220 = To Double Precision Float(number=w592) -> (double precision float=w590:dbl)
                            "FullSpeed1 Current" <- w590
                            n221 = Multiply(x=25.0, y=w590) -> (x*y=w584:dbl)
                            n222 = Greater Or Equal?(x=w584, y=w603) -> (x >= y?=w582:bool)
                            n223 = Greater Or Equal?(x=w579, y=10000.0) -> (x >= y?=w577:bool)
                            n224 = And(x=w577, y=w582) -> (x .and. y?=w581:bool)
                            n225 = call "Write panel message Kinetics (SubVI).vi"(4:"rpm"=w580, 5:"rpm"=TRUE ("rpm"), "PrintTime"=FALSE, "Stop"=w585, "error in (no error)"=w591, "Time to wait"=0.2, "Strin"=w595, "String in"=w586) -> ("error out"=w597:errorcluster, "Stopped"=w576:bool)  [unwired: 2 in]
                            n226 = Compound Arithmetic op=OR(w576, w588, w598, w581) -> (w604:bool)
                          }
                          n227 = Select(t=T7."Stop", s=w559, f=T7."MD[1]=1") -> (s? t:f=w571:T7)
                        }
                        frame "MD[1]=0" {
                          n228 = call "Operation (SubVI).vi"("On/Off"=FALSE, "Operation"=T5."Venable", "DAQmx Device Name"=w610) -> ("error out"=w633:errorcluster)  [unwired: 8 in]
                          n229 = Concatenate Strings(w614, "\nSet Parameters MD[1]=0" ("Strin")) -> (w625:string)
                          n230 = call "Write panel message Kinetics (SubVI).vi"(4:"rpm"=w618, 5:"rpm"=FALSE ("rpm"), "PrintTime"=FALSE, "Stop"=w623, "error in (no error)"=w633, "Time to wait"=0.2, "Strin"=w625, "String in"=w624) -> ("error out"=w632:errorcluster, "Stopped"=w606:bool)  [unwired: 2 in]
                          n231 = call "Serial.vi"("error in (no error)"=w632, "write buffer"="EP=1\r\nVC=0\r\nMD[1]=0\r\n", "VISA resource name"=w615) -> ("error out"=w629:errorcluster)  [unwired: 7 in, 1 out]
                          n232 = call "Operation (SubVI).vi"("error in (no error)"=w629, "On/Off"=FALSE, "Operation"=T5."PowerSuply", "DAQmx Device Name"=w610) -> ("error out"=w628:errorcluster)  [unwired: 7 in]
                          n233 = call "Write panel message Kinetics (SubVI).vi"(4:"rpm"=w618, 5:"rpm"=FALSE ("rpm"), "PrintTime"=TRUE, "Stop"=w623, "error in (no error)"=w628, "Time to wait"=25.0, "Strin"=w625, "String in"=w624) -> ("error out"=w613:errorcluster, "Stopped"=w607:bool)  [unwired: 2 in]
                          n234 = call "Operation (SubVI).vi"("error in (no error)"=w613, "On/Off"=TRUE, "Operation"=T5."PowerSuply", "DAQmx Device Name"=w610) -> ("error out"=w612:errorcluster)  [unwired: 7 in]
                          n235 = call "Operation (SubVI).vi"("error in (no error)"=w612, "On/Off"=TRUE, "Operation"=T5."Venable", "DAQmx Device Name"=w610) -> ("error out"=w620:errorcluster)  [unwired: 7 in]
                          n236 = call "Write panel message Kinetics (SubVI).vi"(4:"rpm"=w618, 5:"rpm"=FALSE ("rpm"), "PrintTime"=TRUE, "Stop"=w623, "error in (no error)"=w620, "Time to wait"=3.0, "Strin"=w625, "String in"=w624) -> ("Stopped"=w608:bool)  [unwired: 2 in, 1 out]
                          n237 = Compound Arithmetic op=OR(w608, w607, w606) -> (w605:bool)
                          n238 = Compound Arithmetic op=OR(w608, w607, w606) -> (w617:bool)
                          n239 = Select(t=T7."Stop", s=w617, f=T7."FullSpeed1") -> (s? t:f=w646:T7)
                        }
                      }
                    }
                  }
                }
              }
            }
          }
        }
        frame "Venable Test" {
          n240 = control-ref of="Stop Button"() -> (w663:refnum<vi>)
          n241 = control-ref of="ATR"() -> (w664:refnum<vi>)
          n242 = control-ref of="Pannel User Message"() -> (w665:refnum<vi>)
          n243 = control-ref of="Motor Speed RPM Serial"() -> (w666:refnum<vi>)
          n244 = control-ref of="UUT"() -> (w667:refnum<vi>)
          n245 = Concatenate Strings(w659, " in process..." ("Strin")) -> (w660:string)
          n246 = while {
            shift-right: [w674] -> _
            shift-left: enum16{"Stop", "Direction", "Venable", "Start"}."Start" -> [w679]
            tunnel: w663 -> [w678]
            tunnel: w664 -> [w677]
            tunnel: w665 -> [w676]
            tunnel: w666 -> [w675]
            tunnel: w667 -> [w672]
            tunnel: w660 -> [w673]
            tunnel: w659 -> [w671]
            tunnel: w658 -> [w670]
            tunnel: [w668] -> w657
            stop <- w669 stop-if-true
            n247 = case shown="\"Start\"" w679 {
              tunnel: w678 -> [_ w709 w958 w1006]
              tunnel: w677 -> [_ w705 w956 w999]
              tunnel: w676 -> [_ w708 w959 w1012]
              tunnel: w675 -> [_ w707 w960 _]
              tunnel: w672 -> [w680 w701 w961 _]
              tunnel: [w682 FALSE FALSE FALSE] -> w669
              tunnel: [w681 w704 w957 w1010] -> w674
              tunnel: w673 -> [_ w706 w955 w1005]
              tunnel: w671 -> [_ _ _ w998]
              tunnel: w670 -> [_ _ _ w1001]
              tunnel: [_ _ _ w993] -> w668
              frame "Stop", Default {
                n248 = disable-structure shown="Enabled" {
                  disable-tunnel: [w685 TRUE] -> w682
                  disable-tunnel: [w684 enum16{"Stop", "Direction", "Venable", "Start"}."Stop"] -> w681
                  disable-tunnel: w680 -> [w683 _]
                  frame Disabled {
                    n249 = flat-sequence {
                      tunnel: w683 -> [_]
                      tunnel: [TRUE] -> w685
                      tunnel: [enum16{"Stop", "Direction", "Venable", "Start"}."Stop"] -> w684
                      frame #0 {
                        (unwired) u16 0 ("Motor Speed RPM")
                        (unwired) TRUE ("Remote")
                        n250 = property on="VISA Kinetics" class="VISAName"() -> (error out=w689:errorcluster, "Value"=w690:refnum<visa-resource-name>)  [unwired: 2 in, 1 out]
                        n251 = call "Serial.vi"("error in (no error)"=w689, "Clear Log"=FALSE, "write buffer"="EP=1\r\nMD[1]=1\r\n", "VISA resource name"=w690) -> ("error out"=w686:errorcluster)  [unwired: 6 in, 1 out]
                        n252 = call "CANSendMessage.vi"("error in (no error)"=w686) -> ("error out"=w695:errorcluster)  [unwired: 10 in]
                        n253 = call "TesterOption (SubVI).vi"("2 Options"=FALSE, "error in (no error)"=w695, "On/Off"=FALSE, "Tester Option"=T8."Venable") -> ("error out"=w691:errorcluster)  [unwired: 6 in, 1 out]
                        n254 = call "Time Delay9"("error in (no error)"=w691) -> ()  [unwired: 10 in, 1 out]
                      }
                      frame #1 {
                      }
                    }
                  }
                  frame Enabled {
                  }
                }
              }
              frame "Direction" {
                n255 = property on="UUT" class="DigNum (strict)"() -> ("Value"=w700:u8)  [unwired: 2 in, 2 out]
                n256 = while {
                  shift-right: [w720] -> w703
                  shift-left: T7."MD[1]=0" -> [w721]
                  tunnel: w701 -> [w718]
                  tunnel: w709 -> [w717]
                  tunnel: w708 -> [w716]
                  tunnel: w707 -> [w715]
                  tunnel: w706 -> [w714]
                  tunnel: w705 -> [w713]
                  tunnel: w700 -> [w712]
                  stop <- w719 stop-if-true
                  n257 = case shown="\"FullSpeed2\"" w721 {
                    tunnel: [T7."Stop" w745 w782 w852 w880 w950] -> w720
                    tunnel: [TRUE FALSE FALSE FALSE FALSE FALSE] -> w719
                    tunnel: w718 -> [_ _ _ _ _ _]
                    tunnel: w717 -> [_ w732 w759 w822 w860 w918]
                    tunnel: w716 -> [_ _ w758 w831 w859 w928]
                    tunnel: w715 -> [_ _ w775 w820 w874 w924]
                    tunnel: w714 -> [_ _ w770 w839 w872 w936]
                    tunnel: w713 -> [_ w736 _ _ _ _]
                    tunnel: w712 -> [_ w724 w756 _ w854 _]
                    frame "Stop", Default {
                    }
                    frame "Result" {
                      n258 = property on="FullSpeed1 Current" class="DigNum (strict)"() -> ("Value"=w740:dbl)  [unwired: 2 in, 2 out]
                      n259 = property on="FullSpeed2 Current" class="DigNum (strict)"() -> ("Value"=w741:dbl)  [unwired: 2 in, 2 out]
                      n260 = property on="FullSpeed2 Speed" class="DigNum (strict)"() -> ("Value"=w743:dbl)  [unwired: 2 in, 2 out]
                      n261 = property on="FullSpeed1 Speed" class="DigNum (strict)"() -> ("Value"=w742:dbl)  [unwired: 2 in, 2 out]
                      n262 = Subtract(x=w741, y=w740) -> (x-y=w739:dbl)
                      n263 = Absolute Value(x=w739) -> (abs(x)=w728:dbl)
                      n264 = Greater Or Equal?(x=w728, y=u32 5) -> (x >= y?=w734:bool)
                      n265 = Equal?(x=w724, y=u8 95) -> (x = y?=w726:bool)
                      n266 = case shown="True" w726 {
                        tunnel: w743 -> [_ w754]
                        tunnel: w742 -> [_ w753]
                        tunnel: [TRUE w750] -> w735
                        frame False {
                        }
                        frame True {
                          n267 = Subtract(x=w754, y=w753) -> (x-y=w755:dbl)
                          n268 = Absolute Value(x=w755) -> (abs(x)=w752:dbl)
                          n269 = Greater Or Equal?(x=w752, y=500.0) -> (x >= y?=w750:bool)
                        }
                      }
                      n270 = call "Find_Number_LineMARVIN.vi"("Test Paragraph"="Motor Rotation Direction", "TableIn"=w736) -> ("Line number"=w733:i32)  [unwired: 3 in, 3 out]
                      n271 = And(x=w735, y=w734) -> (x .and. y?=w725:bool)
                      "VenableDirectionResult" <- w725
                      n272 = call "PassOrFail (SubVI).vi"("String Res"="", "index (row)"=w733, "Data in"=-3.0, "Pass?Fail"=w725, "Table in"=w736) -> ("error out"=w731:errorcluster)  [unwired: 6 in]
                      n273 = property class="Bool (strict)"(reference=w732, error in=w731) -> ("Value"=w748:bool)  [unwired: 2 out]
                      n274 = Select(t=T7."Stop", s=w748, f=T7."Stop") -> (s? t:f=w745:T7)
                    }
                    frame "FullSpeed2" {
                      (unwired) TRUE ("Remote")
                      n275 = Concatenate Strings(w770, "\nFull speed operation " ("string")) -> (w757:string)
                      n276 = call "CANSendMessage.vi"() -> ("error out"=w777:errorcluster)  [unwired: 11 in]
                      n277 = call "Write panel message Kinetics (SubVI).vi"(4:"rpm"=w775, 5:"rpm"=TRUE ("rpm"), "PrintTime"=FALSE, "Stop"=w759, "error in (no error)"=w777, "Time to wait"=0.2, "Strin"=w757, "String in"=w758) -> ("error out"=w762:errorcluster)  [unwired: 2 in, 1 out]
                      n278 = Equal?(x=w756, y=u8 95) -> (x = y?=w765:bool)
                      n279 = Select(t=u16 15100, s=w765, f=u16 12100 ("y")) -> ()  [unwired: 1 out]
                      n280 = flat-sequence {
                        tunnel: w762 -> [w787]
                        tunnel: [w787] -> w761
                        tunnel: [w786] -> w760
                        frame #0 {
                          n281 = call <vilib>:"High Resolution Relative Seconds.vi"() -> ("relative seconds"=w786:dbl)
                        }
                      }
                      n282 = Select(t=14500.0, s=w765, f=11500.0) -> (s? t:f=w764:dbl)
                      n283 = Select(t=47.0, s=w765, f=24.0) -> (s? t:f=w763:dbl)
                      n284 = while {
                        tunnel: w775 -> [w789]
                        tunnel: w761 -> [w813]
                        tunnel: [w796] -> w772
                        tunnel: w764 -> [w809]
                        tunnel: w763 -> [w808]
                        tunnel: w760 -> [w804]
                        tunnel: w759 -> [w794]
                        tunnel: w758 -> [w795]
                        tunnel: w757 -> [w792]
                        stop <- w806 stop-if-true
                        n285 = call <vilib>:"High Resolution Relative Seconds.vi"() -> ("relative seconds"=w805:dbl)
                        n286 = Subtract(x=w805, y=w804) -> (x-y=w803:dbl)
                        n287 = property class="DigNum (strict)"(reference=w789, error in=w813) -> ("Value"=w810:dbl)  [unwired: 2 out]
                        "FullSpeed2 Speed" <- w810
                        n288 = Greater Or Equal?(x=w803, y=120.0) -> (x >= y?=w801:bool)
                        n289 = Greater Or Equal?(x=w810, y=w809) -> (x >= y?=w800:bool)
                        n290 = property class="Bool (strict)"(reference=w794) -> ("Value"=w799:bool)  [unwired: 1 in, 2 out]
                        n291 = call "GetADCTester (SubVI).vi"("GetADCTester"=T9."Current", "TimeToGet"=5) -> ("error out"=w811:errorcluster, "ADCValOutput Single"=w807:dbl)  [unwired: 7 in, 1 out]
                        "FullSpeed2 Current" <- w807
                        n292 = Greater Or Equal?(x=w807, y=w808) -> (x >= y?=w797:bool)
                        n293 = And(x=w800, y=w797) -> (x .and. y?=w798:bool)
                        n294 = Compound Arithmetic op=OR(w799, w801, w798) -> (w806:bool)
                        n295 = call "Write panel message Kinetics (SubVI).vi"(4:"rpm"=w789, 5:"rpm"=TRUE ("rpm"), "PrintTime"=FALSE, "Stop"=w794, "error in (no error)"=w811, "Time to wait"=0.2, "Strin"=w792, "String in"=w795) -> ("error out"=w796:errorcluster)  [unwired: 2 in, 1 out]
                      }
                      n296 = property class="Bool (strict)"(reference=w759, error in=w772) -> ("Value"=w785:bool)  [unwired: 2 out]
                      n297 = Select(t=T7."Stop", s=w785, f=T7."Result") -> (s? t:f=w782:T7)
                    }
                    frame "MD[1]=1" {
                      (unwired) TRUE ("Remote")
                      (unwired) u16 0 ("Motor Speed RPM")
                      n298 = Concatenate Strings(w839, "\nSet Parameters MD[1]=1" ("Strin")) -> (w830:string)
                      n299 = call "TesterOption (SubVI).vi"("2 Options"=FALSE, "On/Off"=FALSE, "Tester Option"=T8."Venable") -> ("error out"=w844:errorcluster, "VISA Refnum out"=w835:refnum<visa-resource-name>)  [unwired: 7 in]
                      n300 = call "CANSendMessage.vi"("error in (no error)"=w844) -> ("error out"=w846:errorcluster)  [unwired: 10 in]
                      n301 = call "Write panel message Kinetics (SubVI).vi"(4:"rpm"=w820, 5:"rpm"=FALSE ("rpm"), "PrintTime"=TRUE, "Stop"=w822, "error in (no error)"=w846, "Time to wait"=20.0, "Strin"=w830, "String in"=w831) -> ("error out"=w819:errorcluster)  [unwired: 2 in, 1 out]
                      n302 = property on="VISA Kinetics" class="VISAName"(error in=w819) -> (error out=w845:errorcluster, "Value"=w848:refnum<visa-resource-name>)  [unwired: 1 in, 1 out]
                      n303 = call "Serial.vi"("error in (no error)"=w845, "Clear Log"=FALSE, "write buffer"="EP=1\r\nMD[1]=1\r\n", "VISA resource name"=w848) -> ("error out"=w834:errorcluster)  [unwired: 6 in, 1 out]
                      n304 = call "TesterOption (SubVI).vi"("2 Options"=FALSE, "error in (no error)"=w834, "On/Off"=FALSE, "Tester Option"=T8."Power", "VISA Refnum in"=w835) -> ("error out"=w832:errorcluster, "VISA Refnum out"=w823:refnum<visa-resource-name>)  [unwired: 5 in]
                      n305 = call "Write panel message Kinetics (SubVI).vi"(4:"rpm"=w820, 5:"rpm"=FALSE ("rpm"), "PrintTime"=TRUE, "Stop"=w822, "error in (no error)"=w832, "Time to wait"=25.0, "Strin"=w830, "String in"=w831) -> ("error out"=w824:errorcluster)  [unwired: 2 in, 1 out]
                      n306 = call "TesterOption (SubVI).vi"("2 Options"=FALSE, "error in (no error)"=w824, "On/Off"=TRUE, "Tester Option"=T8."Venable", "VISA Refnum in"=w823) -> ("error out"=w821:errorcluster)  [unwired: 5 in, 1 out]
                      n307 = call "Time Delay8"("error in (no error)"=w821) -> ("error out"=w817:errorcluster)  [unwired: 10 in]
                      n308 = property class="Bool (strict)"(reference=w822, error in=w817) -> ("Value"=w853:bool)  [unwired: 2 out]
                      n309 = Select(t=T7."Stop", s=w853, f=T7."FullSpeed2") -> (s? t:f=w852:T7)
                    }
                    frame "FullSpeed1" {
                      (unwired) TRUE ("Remote")
                      n310 = call "CANSendMessage.vi"() -> ("error out"=w875:errorcluster)  [unwired: 11 in]
                      n311 = Concatenate Strings(w872, "\nFull speed operation " ("string")) -> (w858:string)
                      n312 = call "Write panel message Kinetics (SubVI).vi"(4:"rpm"=w874, 5:"rpm"=TRUE ("rpm"), "PrintTime"=FALSE, "Stop"=w860, "error in (no error)"=w875, "Time to wait"=0.2, "Strin"=w858, "String in"=w859) -> ("error out"=w863:errorcluster)  [unwired: 2 in, 1 out]
                      n313 = Equal?(x=w854, y=u8 95) -> (x = y?=w870:bool)
                      n314 = flat-sequence {
                        tunnel: w863 -> [w885]
                        tunnel: [w885] -> w862
                        tunnel: [w884] -> w861
                        frame #0 {
                          n315 = call <vilib>:"High Resolution Relative Seconds.vi"() -> ("relative seconds"=w884:dbl)
                        }
                      }
                      n316 = Select(t=u16 15100, s=w870, f=u16 12100 ("y")) -> ()  [unwired: 1 out]
                      n317 = Select(t=13700.0, s=w870, f=11500.0) -> (s? t:f=w865:dbl)
                      n318 = Select(t=56.0, s=w870, f=33.0) -> (s? t:f=w864:dbl)
                      n319 = while {
                        tunnel: w874 -> [w887]
                        tunnel: w862 -> [w911]
                        tunnel: [w894] -> w873
                        tunnel: w865 -> [w906]
                        tunnel: w864 -> [w903]
                        tunnel: w861 -> [w901]
                        tunnel: w860 -> [w892]
                        tunnel: w859 -> [w893]
                        tunnel: w858 -> [w890]
                        stop <- w908 stop-if-true
                        n320 = property class="DigNum (strict)"(reference=w887, error in=w911) -> ("Value"=w907:dbl)  [unwired: 2 out]
                        "FullSpeed1 Speed" <- w907
                        n321 = call <vilib>:"High Resolution Relative Seconds.vi"() -> ("relative seconds"=w902:dbl)
                        n322 = Subtract(x=w902, y=w901) -> (x-y=w900:dbl)
                        n323 = Greater Or Equal?(x=w900, y=120.0) -> (x >= y?=w898:bool)
                        n324 = Greater Or Equal?(x=w907, y=w906) -> (x >= y?=w905:bool)
                        n325 = call "GetADCTester (SubVI).vi"("GetADCTester"=T9."Current", "TimeToGet"=5) -> ("error out"=w909:errorcluster, "ADCValOutput Single"=w904:dbl)  [unwired: 7 in, 1 out]
                        "FullSpeed1 Current" <- w904
                        n326 = Greater Or Equal?(x=w904, y=w903) -> (x >= y?=w895:bool)
                        n327 = And(x=w895, y=w905) -> (x .and. y?=w896:bool)
                        n328 = property class="Bool (strict)"(reference=w892) -> ("Value"=w897:bool)  [unwired: 1 in, 2 out]
                        n329 = call "Write panel message Kinetics (SubVI).vi"(4:"rpm"=w887, 5:"rpm"=TRUE ("rpm"), "PrintTime"=FALSE, "Stop"=w892, "error in (no error)"=w909, "Time to wait"=0.2, "Strin"=w890, "String in"=w893) -> ("error out"=w894:errorcluster)  [unwired: 2 in, 1 out]
                        n330 = Compound Arithmetic op=OR(w897, w896, w898) -> (w908:bool)
                      }
                      n331 = property class="Bool (strict)"(reference=w860, error in=w873) -> ("Value"=w883:bool)  [unwired: 2 out]
                      n332 = Select(t=T7."Stop", s=w883, f=T7."MD[1]=1") -> (s? t:f=w880:T7)
                    }
                    frame "MD[1]=0" {
                      (unwired) TRUE ("Remote")
                      (unwired) u16 0 ("Motor Speed RPM")
                      n333 = Concatenate Strings(w936, "\nSet Parameters MD[1]=0" ("Strin")) -> (w927:string)
                      n334 = call "TesterOption (SubVI).vi"("2 Options"=FALSE, "On/Off"=FALSE, "Tester Option"=T8."Venable") -> ("error out"=w942:errorcluster, "VISA Refnum out"=w932:refnum<visa-resource-name>)  [unwired: 7 in]
                      n335 = call "CANSendMessage.vi"("error in (no error)"=w942) -> ("error out"=w944:errorcluster)  [unwired: 10 in]
                      n336 = call "Write panel message Kinetics (SubVI).vi"(4:"rpm"=w924, 5:"rpm"=FALSE ("rpm"), "PrintTime"=FALSE, "Stop"=w918, "error in (no error)"=w944, "Time to wait"=0.2, "Strin"=w927, "String in"=w928) -> ("error out"=w939:errorcluster)  [unwired: 2 in, 1 out]
                      n337 = property on="VISA Kinetics" class="VISAName"(error in=w939) -> (error out=w943:errorcluster, "Value"=w946:refnum<visa-resource-name>)  [unwired: 1 in, 1 out]
                      n338 = call "Serial.vi"("error in (no error)"=w943, "Clear Log"=FALSE, "write buffer"="EP=1\r\nMD[1]=0\r\n", "VISA resource name"=w946) -> ("error out"=w931:errorcluster)  [unwired: 6 in, 1 out]
                      n339 = call "TesterOption (SubVI).vi"("2 Options"=FALSE, "error in (no error)"=w931, "On/Off"=FALSE, "Tester Option"=T8."Power", "VISA Refnum in"=w932) -> ("error out"=w929:errorcluster, "VISA Refnum out"=w919:refnum<visa-resource-name>)  [unwired: 5 in]
                      n340 = call "Write panel message Kinetics (SubVI).vi"(4:"rpm"=w924, 5:"rpm"=FALSE ("rpm"), "PrintTime"=TRUE, "Stop"=w918, "error in (no error)"=w929, "Time to wait"=25.0, "Strin"=w927, "String in"=w928) -> ("error out"=w920:errorcluster)  [unwired: 2 in, 1 out]
                      n341 = call "TesterOption (SubVI).vi"("2 Options"=FALSE, "error in (no error)"=w920, "On/Off"=TRUE, "Tester Option"=T8."Venable", "VISA Refnum in"=w919) -> ("error out"=w917:errorcluster)  [unwired: 5 in, 1 out]
                      n342 = call "Time Delay4"("error in (no error)"=w917) -> ("error out"=w913:errorcluster)  [unwired: 10 in]
                      n343 = property class="Bool (strict)"(reference=w918, error in=w913) -> ("Value"=w951:bool)  [unwired: 2 out]
                      n344 = Select(t=T7."Stop", s=w951, f=T7."FullSpeed1") -> (s? t:f=w950:T7)
                    }
                  }
                }
                n345 = flat-sequence {
                  tunnel: [enum16{"Stop", "Direction", "Venable", "Start"}."Stop"] -> w704
                  tunnel: w703 -> [_]
                  frame #0 {
                  }
                }
              }
              frame "Venable" {
                n346 = call "Find_Number_LineMARVIN.vi"("Test Paragraph"="Enable Test", "TableIn"=w956) -> ("Line number"=w962:i32)  [unwired: 3 in, 3 out]
                n347 = Increment(x=w962) -> (x+1=w952:i32)
                n348 = for {
                  tunnel: u16[] [5000, 0, 5000] -> [w987] mode=indexing
                  tunnel: bool[] [TRUE, FALSE, TRUE] -> [w985] mode=indexing
                  tunnel: w952 -> [w988]
                  tunnel: w961 -> [_]
                  tunnel: w960 -> [w978]
                  tunnel: w959 -> [w981]
                  tunnel: w958 -> [w980]
                  tunnel: w956 -> [w974]
                  tunnel: w955 -> [w972]
                  tunnel: [w971] -> w954 mode=indexing
                  i -> [w989]
                  (unwired) u16 5000 ("Motor Speed RPM")
                  (unwired) TRUE ("Remote")
                  w990 = 200.0 ("y")
                  n349 = call "CANSendMessage.vi"() -> ("error out"=w984:errorcluster)  [unwired: 11 in]
                  n350 = Add(x=w988, y=w989) -> (x+y=w975:i32)
                  n351 = call "TesterOption (SubVI).vi"("2 Options"=FALSE, "error in (no error)"=w984, "On/Off"=w985, "Tester Option"=T8."Venable") -> ("error out"=w983:errorcluster)  [unwired: 6 in, 1 out]
                  n352 = call "Write panel message Kinetics (SubVI).vi"(4:"rpm"=w978, 5:"rpm"=TRUE ("rpm"), "PrintTime"=TRUE, "Stop"=w980, "error in (no error)"=w983, "Time to wait"=15.0, "Strin"=w972, "String in"=w981) -> ("error out"=w982:errorcluster)  [unwired: 2 in, 1 out]
                  n353 = property class="DigNum (strict)"(reference=w978, error in=w982) -> ("Value"=w973:dbl)  [unwired: 2 out]
                  n354 = Add(x=w987, y=w990) -> (x+y=w992:dbl)
                  n355 = Subtract(x=w987, y=w990) -> (x-y=w991:dbl)
                  n356 = In Range and Coerce(upper limit=w992, x=w973, lower limit=w991) -> (In Range?=w971:bool)  [unwired: 1 out]
                  n357 = call "PassOrFail (SubVI).vi"("index (row)"=w975, "Data in"=w973, "Pass?Fail"=w971, "Table in"=w974) -> ()  [unwired: 7 in, 1 out]
                }
                n358 = property class="Bool (strict)"(reference=w958) -> ("Value"=w969:bool)  [unwired: 1 in, 2 out]
                n359 = And Array Elements(Boolean array=w954) -> (logical AND=→"VenableResult":bool)
                n360 = Select(t=enum16{"Stop", "Direction", "Venable", "Start"}."Stop", s=w969, f=enum16{"Stop", "Direction", "Venable", "Start"}."Direction") -> (s? t:f=w957:enum16{"Stop", "Direction", "Venable", "Start"})
              }
              frame "Start" {
                n361 = property class="Str"(reference=w1012, "Value"=w1005) -> (error out=w1009:errorcluster)  [unwired: 1 in, 1 out]
                n362 = call "Find_Number_LineMARVIN.vi"("Test Paragraph"=w998, "error in"=w1009, "TableIn"=w999) -> ("error out"=w1000:errorcluster, "Line number"=w997:i32)  [unwired: 2 in, 2 out]
                n363 = call "Table_ScrollaBarMarvin.vi"("error in"=w1000, "Line to focus"=w998, "reference in"=w999) -> ("error out"=w1013:errorcluster)  [unwired: 2 out]
                n364 = call "Reset old test Values (SubVI) Kinetics.vi"("error in"=w1013, "Atr in"=w999, "Test Paragraph"=w998) -> ("error out"=w994:errorcluster)  [unwired: 6 in, 2 out]
                n365 = Increment(x=w997) -> (x+1=w996:i32)
                n366 = while {
                  shift-right: [w1025] -> _
                  shift-left: T6."VC=1000" -> [w1028]
                  tunnel: w994 -> [w1027]
                  tunnel: w1001 -> [w1026]
                  tunnel: w998 -> [w1024]
                  shift-right: [w1021] -> w1004
                  shift-left: bool[] [FALSE, FALSE] -> [w1022]
                  tunnel: w996 -> [w1020]
                  tunnel: w999 -> [w1019]
                  shift-right: [w1017] -> _
                  shift-left: dbl[] [0.0, 0.0] -> [w1018]
                  tunnel: [w1015] -> w993
                  i -> [w1023]
                  stop <- w1016 stop-if-true
                  n367 = case shown="\"Wait\"" w1028 {
                    tunnel: w1027 -> [_ w1046 _ w1092 _]
                    tunnel: w1026 -> [_ w1045 w1061 w1096 _]
                    tunnel: [T6."Exit" T6."Wait" w1058 T6."Wait" T6."ReadVC"] -> w1025
                    tunnel: w1024 -> [_ _ _ _ w1103]
                    tunnel: [TRUE FALSE FALSE FALSE w1098] -> w1016
                    tunnel: w1023 -> [_ _ w1059 _ _]
                    tunnel: w1022 -> [w1030 w1043 w1057 w1094 w1100]
                    tunnel: [w1030 w1043 w1056 w1094 w1100] -> w1021
                    tunnel: w1020 -> [w1031 _ _ _ _]
                    tunnel: w1019 -> [w1032 _ _ _ _]
                    tunnel: w1018 -> [w1029 w1041 w1054 w1087 w1099]
                    tunnel: [w1029 w1041 w1053 w1087 w1099] -> w1017
                    tunnel: [_ _ _ _ w1098] -> w1015
                    frame "Exit", Default {
                      n368 = for {
                        tunnel: w1032 -> [w1040]
                        tunnel: w1031 -> [w1039]
                        tunnel: w1030 -> [w1038] mode=indexing
                        tunnel: w1029 -> [w1035] mode=indexing
                        i -> [w1036]
                        n369 = Add(x=w1036, y=w1039) -> (x+y=w1037:i32)
                        n370 = call "PassOrFail (SubVI).vi"("index (row)"=w1037, "Data in"=w1035, "Pass?Fail"=w1038, "Table in"=w1040) -> ()  [unwired: 7 in, 1 out]
                      }
                    }
                    frame "VC=0" {
                      n371 = disable-structure shown="Enabled" {
                        disable-tunnel: w1046 -> [w1049 _]
                        disable-tunnel: w1045 -> [w1047 _]
                        frame Disabled {
                          n372 = call "Serial.vi"("error in (no error)"=w1049, "write buffer"="EP=1\r\nVC=0\r\n", "VISA resource name"=w1047) -> ()  [unwired: 7 in, 2 out]
                        }
                        frame Enabled {
                          n373 = local read "DAQmx Device Name"() -> (w1052:tag)
                          n374 = call "Operation (SubVI).vi"("On/Off"=FALSE, "Operation"=T5."Venable", "DAQmx Device Name"=w1052) -> ()  [unwired: 8 in, 1 out]
                        }
                      }
                    }
                    frame "ReadVC" {
                      n375 = call "Serial.vi"("write buffer"="VC\r\n", "VISA resource name"=w1061) -> ("read buffer"=w1060:string)  [unwired: 8 in, 1 out]
                      n376 = case shown="5, Default" w1059 {
                        tunnel: w1060 -> [w1073 w1083]
                        tunnel: [T6."VC=0" T6."Exit"] -> w1058
                        tunnel: w1057 -> [w1069 w1082]
                        tunnel: [w1067 w1079] -> w1056
                        tunnel: w1054 -> [w1066 w1078]
                        tunnel: [w1063 w1075] -> w1053
                        frame 2 {
                          n377 = Decimal String To Number(string=w1073) -> (number=w1064:i32)  [unwired: 2 in, 1 out]
                          n378 = In Range and Coerce(upper limit=1100, x=w1064, lower limit=900) -> (In Range?=w1068:bool)  [unwired: 1 out]
                          n379 = Replace Array Subset(array=w1066, new element=w1064, index=0) -> (w1063:dbl[])
                          n380 = Replace Array Subset(array=w1069, new element=w1068, index=0) -> (w1067:bool[])
                        }
                        frame 5, Default {
                          n381 = Decimal String To Number(string=w1083) -> (number=w1076:i32)  [unwired: 2 in, 1 out]
                          n382 = In Range and Coerce(upper limit=100, x=w1076, lower limit=0) -> (In Range?=w1080:bool)  [unwired: 1 out]
                          n383 = Replace Array Subset(array=w1078, new element=w1076, index=1) -> (w1075:dbl[])
                          n384 = Replace Array Subset(array=w1082, new element=w1080, index=1) -> (w1079:bool[])
                        }
                      }
                    }
                    frame "VC=1000" {
                      n385 = local read "DAQmx Device Name"() -> (w1093:tag)
                      n386 = call "Operation (SubVI).vi"("error in (no error)"=w1092, "On/Off"=TRUE, "Operation"=T5."Venable", "DAQmx Device Name"=w1093) -> ("error out"=w1091:errorcluster)  [unwired: 7 in]
                      n387 = call "Serial.vi"("error in (no error)"=w1091, "write buffer"="EP=1\r\nVC=1000\r\n", "VISA resource name"=w1096) -> ()  [unwired: 7 in, 2 out]
                    }
                    frame "Wait" {
                      n388 = control-ref of="Motor Speed RPM Serial"() -> (w1108:refnum<vi>)
                      n389 = control-ref of="Pannel User Message"() -> (w1107:refnum<vi>)
                      n390 = control-ref of="Stop Button"() -> (w1102:refnum<vi>)
                      n391 = call "Write panel message Kinetics (SubVI).vi"(4:"rpm"=w1108, 5:"rpm"=TRUE ("rpm"), "PrintTime"=TRUE, "Stop"=w1102, "Time to wait"=20.0, "Strin"=w1103, "String in"=w1107) -> ("Stopped"=w1098:bool)  [unwired: 3 in, 1 out]
                    }
                  }
                }
                n392 = And Array Elements(Boolean array=w1004) -> ()  [unwired: 1 out]
                n393 = property class="Bool (strict)"(reference=w1006) -> ("Value"=w1014:bool)  [unwired: 1 in, 2 out]
                n394 = Select(t=enum16{"Stop", "Direction", "Venable", "Start"}."Stop", s=w1014, f=enum16{"Stop", "Direction", "Venable", "Start"}."Stop") -> (s? t:f=w1010:enum16{"Stop", "Direction", "Venable", "Start"})
              }
            }
          }
        }
        frame "Motor Thermistor Test" {
          n395 = Concatenate Strings(w1120, " in process..." ("Strin")) -> (w1121:string)
          n396 = control-ref of="ATR"() -> (w1123:refnum<vi>)
          n397 = control-ref of="Pannel User Message"() -> (w1124:refnum<vi>)
          n398 = property class="Str"(reference=w1124, "Value"=w1121) -> (error out=w1117:errorcluster)  [unwired: 1 in, 1 out]
          n399 = call "Find_Number_LineMARVIN.vi"("Test Paragraph"=w1120, "error in"=w1117, "TableIn"=w1123) -> ("error out"=w1114:errorcluster, "Line number"=w1113:i32)  [unwired: 2 in, 2 out]
          n400 = call "Table_ScrollaBarMarvin.vi"("error in"=w1114, "Line to focus"=w1120, "reference in"=w1123) -> ("error out"=w1118:errorcluster)  [unwired: 2 out]
          n401 = call "Reset old test Values (SubVI) Kinetics.vi"("error in"=w1118, "Atr in"=w1123, "Test Paragraph"=w1120) -> ("error out"=w1110:errorcluster)  [unwired: 6 in, 2 out]
          n402 = Increment(x=w1113) -> (x+1=w1112:i32)
          n403 = while {
            shift-right: [w1135] -> _
            shift-left: T6."VC=1000" -> [w1138]
            tunnel: w1110 -> [w1137]
            tunnel: w1119 -> [w1136]
            tunnel: w1120 -> [w1134]
            shift-right: [w1130] -> _
            shift-left: bool[] [FALSE, FALSE] -> [w1131]
            tunnel: w1112 -> [w1129]
            tunnel: w1123 -> [w1128]
            shift-right: [w1126] -> _
            shift-left: dbl[] [0.0, 0.0] -> [w1127]
            tunnel: [w1125] -> w1109
            i -> [w1132]
            stop <- w1133 stop-if-true
            n404 = case shown="\"Wait\"" w1138 {
              tunnel: w1137 -> [_ w1162 _ w1219 _]
              tunnel: w1136 -> [w1139 w1161 w1178 w1223 _]
              tunnel: [T6."Exit" T6."Wait" w1175 T6."Wait" T6."ReadVC"] -> w1135
              tunnel: w1134 -> [_ _ _ _ w1230]
              tunnel: [TRUE FALSE FALSE FALSE w1225] -> w1133
              tunnel: w1132 -> [_ w1156 w1176 _ _]
              tunnel: w1131 -> [w1145 w1159 w1174 w1221 w1227]
              tunnel: [w1145 w1159 w1173 w1221 w1227] -> w1130
              tunnel: w1129 -> [w1146 _ _ _ _]
              tunnel: w1128 -> [w1147 _ _ _ _]
              tunnel: w1127 -> [w1144 w1157 w1171 w1214 w1226]
              tunnel: [w1144 w1157 w1170 w1214 w1226] -> w1126
              tunnel: [_ _ _ _ w1225] -> w1125
              frame "Exit", Default {
                n405 = for {
                  tunnel: w1147 -> [w1155]
                  tunnel: w1146 -> [w1154]
                  tunnel: w1145 -> [w1153] mode=indexing
                  tunnel: w1144 -> [w1150] mode=indexing
                  i -> [w1151]
                  n406 = Add(x=w1151, y=w1154) -> (x+y=w1152:i32)
                  n407 = call "PassOrFail (SubVI).vi"("index (row)"=w1152, "Data in"=w1150, "Pass?Fail"=w1153, "Table in"=w1155) -> ()  [unwired: 7 in, 1 out]
                }
                n408 = local read "DAQmx Device Name"() -> (w1143:tag)
                n409 = call "Serial.vi"("write buffer"="EP=1\r\nVC=0\r\n", "VISA resource name"=w1139) -> ()  [unwired: 8 in, 2 out]
                n410 = call "Operation (SubVI).vi"("On/Off"=FALSE, "Operation"=T5."Venable", "DAQmx Device Name"=w1143) -> ()  [unwired: 8 in, 1 out]
              }
              frame "VC=0" {
                n411 = disable-structure shown="Enabled" {
                  disable-tunnel: w1162 -> [w1165 _]
                  disable-tunnel: w1161 -> [w1163 _]
                  disable-tunnel: w1156 -> [_ w1166]
                  frame Disabled {
                    n412 = call "Serial.vi"("error in (no error)"=w1165, "write buffer"="EP=1\r\nVC=0\r\n", "VISA resource name"=w1163) -> ()  [unwired: 7 in, 2 out]
                  }
                  frame Enabled {
                    n413 = case shown="6, Default" w1166 {
                      tunnel: ["Connect wires of the thermistor" ("message") "Disconnect wires of the thermistor" ("message")] -> w1167
                      frame 6, Default {
                      }
                      frame 3 {
                      }
                    }
                    n414 = One Button Dialog(message=w1167) -> ()  [unwired: 1 in, 1 out]
                  }
                }
              }
              frame "ReadVC" {
                n415 = call "Serial.vi"("write buffer"="VC\r\n", "VISA resource name"=w1178) -> ("read buffer"=w1177:string)  [unwired: 8 in, 1 out]
                n416 = case shown="2" w1176 {
                  tunnel: w1177 -> [w1189 w1198 w1210]
                  tunnel: [w1183 T6."VC=0" T6."Exit"] -> w1175
                  tunnel: w1174 -> [w1180 w1197 w1209]
                  tunnel: [w1180 w1194 w1206] -> w1173
                  tunnel: w1171 -> [w1181 w1193 w1205]
                  tunnel: [w1181 w1190 w1202] -> w1170
                  frame 2 {
                    n417 = Decimal String To Number(string=w1189) -> (number=w1186:i32)  [unwired: 2 in, 1 out]
                    n418 = In Range and Coerce(upper limit=1100, x=w1186, lower limit=900) -> (In Range?=w1185:bool)  [unwired: 1 out]
                    n419 = Select(t=T6."VC=0", s=w1185, f=T6."Exit") -> (s? t:f=w1183:T6)
                  }
                  frame 5, Default {
                    n420 = Decimal String To Number(string=w1198) -> (number=w1191:i32)  [unwired: 2 in, 1 out]
                    n421 = In Range and Coerce(upper limit=100, x=w1191, lower limit=0) -> (In Range?=w1195:bool)  [unwired: 1 out]
                    n422 = Replace Array Subset(array=w1193, new element=w1191, index=0) -> (w1190:dbl[])
                    n423 = Replace Array Subset(array=w1197, new element=w1195, index=0) -> (w1194:bool[])
                  }
                  frame 8 {
                    n424 = Decimal String To Number(string=w1210) -> (number=w1203:i32)  [unwired: 2 in, 1 out]
                    n425 = In Range and Coerce(upper limit=1100, x=w1203, lower limit=900) -> (In Range?=w1207:bool)  [unwired: 1 out]
                    n426 = Replace Array Subset(array=w1205, new element=w1203, index=1) -> (w1202:dbl[])
                    n427 = Replace Array Subset(array=w1209, new element=w1207, index=1) -> (w1206:bool[])
                  }
                }
              }
              frame "VC=1000" {
                n428 = local read "DAQmx Device Name"() -> (w1220:tag)
                n429 = call "Operation (SubVI).vi"("error in (no error)"=w1219, "On/Off"=TRUE, "Operation"=T5."Venable", "DAQmx Device Name"=w1220) -> ("error out"=w1218:errorcluster)  [unwired: 7 in]
                n430 = call "Serial.vi"("error in (no error)"=w1218, "write buffer"="EP=1\r\nVC=1000\r\n", "VISA resource name"=w1223) -> ()  [unwired: 7 in, 2 out]
              }
              frame "Wait" {
                n431 = control-ref of="Motor Speed RPM Serial"() -> (w1235:refnum<vi>)
                n432 = control-ref of="Pannel User Message"() -> (w1234:refnum<vi>)
                n433 = control-ref of="Stop Button"() -> (w1229:refnum<vi>)
                n434 = call "Write panel message Kinetics (SubVI).vi"(4:"rpm"=w1235, 5:"rpm"=TRUE ("rpm"), "PrintTime"=TRUE, "Stop"=w1229, "Time to wait"=20.0, "Strin"=w1230, "String in"=w1234) -> ("Stopped"=w1225:bool)  [unwired: 3 in, 1 out]
              }
            }
          }
        }
        frame "Up/Down Blower Test" {
          n435 = control-ref of="Pannel User Message"() -> (w1256:refnum<vi>)
          n436 = Concatenate Strings(w1247, " in process..." ("Strin")) -> (w1248:string)
          n437 = property class="Str"(reference=w1256, error in=w1255, "Value"=w1248) -> (error out=w1254:errorcluster)  [unwired: 1 out]
          n438 = call "Table_ScrollaBarMarvin.vi"("error in"=w1254, "Line to focus"=w1247, "reference in"=w1240) -> ()  [unwired: 3 out]
          n439 = call "Reset old test Values (SubVI) Kinetics.vi"("Atr in"=w1240, "Test Paragraph"=w1247) -> ("error out"=w1249:errorcluster)  [unwired: 7 in, 2 out]
          n440 = call "Find_Number_LineMARVIN.vi"("Test Paragraph"=w1247, "error in"=w1249, "TableIn"=w1240) -> ("error out"=w1244:errorcluster, "Line number"=w1246:i32)  [unwired: 2 in, 2 out]
          n441 = Increment(x=w1246) -> (x+1=w1239:i32)
          n442 = call "Serial.vi"("error in (no error)"=w1244, "write buffer"="VM[1]\r\n", "VISA resource name"=w1243) -> ("error out"=w1242:errorcluster, "read buffer"=w1237:string)  [unwired: 7 in]
          n443 = call "InsertSingleData.vi"("String In"=w1237, "error in (no error)"=w1242, "Col"=2, "Row"=w1239, "Table in"=w1240) -> ("error out"=w1241:errorcluster)  [unwired: 6 in]
          n444 = while {
            shift-right: [w1268] -> _
            shift-left: T6."VC=1000" -> [w1271]
            tunnel: w1241 -> [w1270]
            tunnel: w1243 -> [w1269]
            tunnel: w1248 -> [w1267]
            shift-right: [w1264] -> _
            shift-left: bool[] [FALSE, FALSE] -> [w1265]
            tunnel: w1239 -> [w1263]
            tunnel: w1240 -> [w1262]
            shift-right: [w1260] -> _
            shift-left: dbl[] [0.0, 0.0] -> [w1261]
            tunnel: w1237 -> [w1259]
            tunnel: [w1257] -> w1236
            i -> [w1266]
            stop <- w1258 stop-if-true
            n445 = case shown="\"Wait\"" w1271 {
              tunnel: w1270 -> [_ w1292 _ w1352 _]
              tunnel: w1269 -> [_ w1291 w1308 w1355 _]
              tunnel: [T6."Exit" T6."Wait" w1305 T6."Wait" T6."ReadVC"] -> w1268
              tunnel: w1267 -> [_ _ _ _ w1362]
              tunnel: [TRUE FALSE FALSE FALSE w1357] -> w1258
              tunnel: w1266 -> [_ _ w1306 _ _]
              tunnel: w1265 -> [w1276 w1289 w1304 w1353 w1359]
              tunnel: [w1276 w1289 w1303 w1353 w1359] -> w1264
              tunnel: w1263 -> [w1277 _ _ _ _]
              tunnel: w1262 -> [w1278 _ _ _ _]
              tunnel: w1261 -> [w1275 w1287 w1301 w1347 w1358]
              tunnel: [w1275 w1287 w1300 w1347 w1358] -> w1260
              tunnel: w1259 -> [_ _ w1299 _ _]
              tunnel: [_ _ _ _ w1357] -> w1257
              frame "Exit", Default {
                n446 = for {
                  tunnel: w1278 -> [w1286]
                  tunnel: w1277 -> [w1285]
                  tunnel: w1276 -> [w1284] mode=indexing
                  tunnel: w1275 -> [w1281] mode=indexing
                  i -> [w1282]
                  n447 = Add(x=w1282, y=w1285) -> (x+y=w1283:i32)
                  n448 = call "PassOrFail (SubVI).vi"("index (row)"=w1283, "Data in"=w1281, "Pass?Fail"=w1284, "Table in"=w1286) -> ()  [unwired: 7 in, 1 out]
                }
                n449 = local read "DAQmx Device Name"() -> (w1274:tag)
                n450 = call "Operation (SubVI).vi"("On/Off"=FALSE, "Operation"=T5."Venable", "DAQmx Device Name"=w1274) -> ()  [unwired: 8 in, 1 out]
              }
              frame "VC=0" {
                n451 = disable-structure shown="Enabled" {
                  disable-tunnel: w1292 -> [w1295 _]
                  disable-tunnel: w1291 -> [w1293 _]
                  frame Disabled {
                    n452 = call "Serial.vi"("error in (no error)"=w1295, "write buffer"="EP=1\r\nVC=0\r\n", "VISA resource name"=w1293) -> ()  [unwired: 7 in, 2 out]
                  }
                  frame Enabled {
                    n453 = local read "DAQmx Device Name"() -> (w1298:tag)
                    n454 = call "Operation (SubVI).vi"("On/Off"=TRUE, "Operation"=T5."Down", "DAQmx Device Name"=w1298) -> ()  [unwired: 8 in, 1 out]
                  }
                }
              }
              frame "ReadVC" {
                n455 = call "Serial.vi"("write buffer"="VC\r\n", "VISA resource name"=w1308) -> ("read buffer"=w1307:string)  [unwired: 8 in, 1 out]
                n456 = case shown="5, Default" w1306 {
                  tunnel: w1307 -> [w1326 w1339]
                  tunnel: [T6."VC=0" T6."Exit"] -> w1305
                  tunnel: w1304 -> [w1324 w1338]
                  tunnel: [w1322 w1335] -> w1303
                  tunnel: w1301 -> [w1321 w1334]
                  tunnel: [w1319 w1331] -> w1300
                  tunnel: w1299 -> [w1313 _]
                  frame 2 {
                    w1314 = 100
                    n457 = Decimal String To Number(string=w1326) -> (number=w1315:i32)  [unwired: 2 in, 1 out]
                    n458 = Decimal String To Number(string=w1313) -> (number=w1310:i32)  [unwired: 2 in, 1 out]
                    n459 = Add(x=w1310, y=w1314) -> (x+y=w1312:i32)
                    n460 = Subtract(x=w1310, y=w1314) -> (x-y=w1311:i32)
                    n461 = In Range and Coerce(upper limit=w1312, x=w1315, lower limit=w1311) -> (In Range?=w1323:bool)  [unwired: 1 out]
                    n462 = Replace Array Subset(array=w1321, new element=w1315, index=0) -> (w1319:dbl[])
                    n463 = Replace Array Subset(array=w1324, new element=w1323, index=0) -> (w1322:bool[])
                    n464 = local read "DAQmx Device Name"() -> (w1318:tag)
                    n465 = call "Operation (SubVI).vi"("On/Off"=FALSE, "Operation"=T5."Up", "DAQmx Device Name"=w1318) -> ()  [unwired: 8 in, 1 out]
                  }
                  frame 5, Default {
                    n466 = Decimal String To Number(string=w1339) -> (number=w1332:i32)  [unwired: 2 in, 1 out]
                    n467 = In Range and Coerce(upper limit=100, x=w1332, lower limit=0) -> (In Range?=w1336:bool)  [unwired: 1 out]
                    n468 = Replace Array Subset(array=w1334, new element=w1332, index=1) -> (w1331:dbl[])
                    n469 = Replace Array Subset(array=w1338, new element=w1336, index=1) -> (w1335:bool[])
                    n470 = local read "DAQmx Device Name"() -> (w1330:tag)
                    n471 = call "Operation (SubVI).vi"("On/Off"=FALSE, "Operation"=T5."Down", "DAQmx Device Name"=w1330) -> ()  [unwired: 8 in, 1 out]
                  }
                }
              }
              frame "VC=1000" {
                n472 = local read "DAQmx Device Name"() -> (w1346:tag)
                n473 = call "Operation (SubVI).vi"("error in (no error)"=w1352, "On/Off"=TRUE, "Operation"=T5."Venable", "DAQmx Device Name"=w1346) -> ("error out"=w1351:errorcluster)  [unwired: 7 in]
                n474 = call "Serial.vi"("error in (no error)"=w1351, "write buffer"="EP=1\r\nVC=0\r\n", "VISA resource name"=w1355) -> ("error out"=w1343:errorcluster)  [unwired: 7 in, 1 out]
                n475 = call "Operation (SubVI).vi"("error in (no error)"=w1343, "On/Off"=TRUE, "Operation"=T5."Up", "DAQmx Device Name"=w1346) -> ()  [unwired: 7 in, 1 out]
              }
              frame "Wait" {
                n476 = control-ref of="Motor Speed RPM Serial"() -> (w1367:refnum<vi>)
                n477 = control-ref of="Pannel User Message"() -> (w1366:refnum<vi>)
                n478 = control-ref of="Stop Button"() -> (w1361:refnum<vi>)
                n479 = call "Write panel message Kinetics (SubVI).vi"(4:"rpm"=w1367, 5:"rpm"=TRUE ("rpm"), "PrintTime"=TRUE, "Stop"=w1361, "Time to wait"=30.0, "Strin"=w1362, "String in"=w1366) -> ("Stopped"=w1357:bool)  [unwired: 3 in, 1 out]
              }
            }
          }
        }
        frame "Resistance Merkava 4 Test" {
          w1369 = T12 [enum."0 ohm", enum."6 ohm", enum."15 ohm"] items=["Init", "0 ohm", "6 ohm", "13.2 ohm", "15 ohm", "25.9 ohm", "33 ohm", "Down", "Up", "Venable", "Firmware", "PowerSuply"]
          w1373 = T12 [enum."6 ohm", enum."15 ohm", enum."15 ohm"] items=["Init", "0 ohm", "6 ohm", "13.2 ohm", "15 ohm", "25.9 ohm", "33 ohm", "Down", "Up", "Venable", "Firmware", "PowerSuply"]
          w1380 = T12 [enum."Venable", enum."Down"] items=["Init", "0 ohm", "6 ohm", "13.2 ohm", "15 ohm", "25.9 ohm", "33 ohm", "Down", "Up", "Venable", "Firmware", "PowerSuply"]
          w1381 = T12 [enum."PowerSuply", enum."Venable", enum."Down", enum."0 ohm", enum."PowerSuply"] items=["Init", "0 ohm", "6 ohm", "13.2 ohm", "15 ohm", "25.9 ohm", "33 ohm", "Down", "Up", "Venable", "Firmware", "PowerSuply"]
          w1388 = T12 [enum."0 ohm", enum."6 ohm", enum."15 ohm"] items=["Init", "0 ohm", "6 ohm", "13.2 ohm", "15 ohm", "25.9 ohm", "33 ohm", "Down", "Up", "Venable", "Firmware", "PowerSuply"]
          # "1.65"
          n480 = control-ref of="Pannel User Message"() -> (w1395:refnum<vi>)
          n481 = Concatenate Strings(w1391, " in process..." ("Strin")) -> (w1382:string)
          n482 = property class="Str"(reference=w1395, error in=w1390, "Value"=w1382) -> (error out=w1394:errorcluster)  [unwired: 1 out]
          n483 = call "Table_ScrollaBarMarvin.vi"("error in"=w1394, "Line to focus"=w1391, "reference in"=w1384) -> ()  [unwired: 3 out]
          n484 = call "Reset old test Values (SubVI) Kinetics.vi"("Atr in"=w1384, "Test Paragraph"=w1391) -> ("error out"=w1393:errorcluster)  [unwired: 7 in, 2 out]
          n485 = call "Find_Number_LineMARVIN.vi"("Test Paragraph"=w1391, "error in"=w1393, "TableIn"=w1384) -> ("error out"=w1389:errorcluster, "Line number"=w1386:i32)  [unwired: 2 in, 2 out]
          n486 = for {
            tunnel: w1381 -> [w1406] mode=indexing
            tunnel: [w1404] -> w1383
            tunnel: w1389 -> [w1405]
            tunnel: [w1401] -> w1377
            tunnel: bool[] [FALSE, TRUE, TRUE, TRUE, TRUE] -> [w1403] mode=indexing
            tunnel: dbl[] [5.0, 0.2, 0.2, 0.2, 3.0] -> [w1400] mode=indexing
            n487 = local read "DAQmx Device Name"() -> (w1404:tag)
            n488 = call "Operation (SubVI).vi"("error in (no error)"=w1405, "On/Off"=w1403, "Operation"=w1406, "DAQmx Device Name"=w1404) -> ("error out"=w1402:errorcluster)  [unwired: 7 in]
            n489 = call "Time Delay6"("error in (no error)"=w1402, "Delay Time (s)"=w1400) -> ("error out"=w1401:errorcluster)  [unwired: 9 in]
          }
          n490 = call "Serial.vi"("error in (no error)"=w1377, "write buffer"="EP=1\r\nCF[0]=4.5\r\n", "VISA resource name"=w1376) -> ("error out"=w1378:errorcluster)  [unwired: 7 in, 1 out]
          n491 = Increment(x=w1386) -> (x+1=w1385:i32)
          n492 = for {
            tunnel: w1388 -> [w1413] mode=indexing
            tunnel: i32[] [6850, 8300, 9200] -> [w1429] mode=indexing
            tunnel: w1385 -> [w1424]
            tunnel: w1384 -> [w1419]
            tunnel: w1378 -> [w1418]
            tunnel: w1383 -> [w1417]
            tunnel: w1382 -> [w1416]
            tunnel: bool[] [TRUE, TRUE, TRUE] -> [w1415] mode=indexing
            tunnel: w1373 -> [w1410] mode=indexing
            tunnel: [w1414] -> w1371
            tunnel: bool[] [TRUE, FALSE] -> [w1412]
            tunnel: w1369 -> [w1409] mode=indexing
            tunnel: [w1408] -> w1368
            i -> [w1425]
            stop <- w1414 stop-if-true
            w1428 = 100 ("x")
            n493 = Add(x=w1424, y=w1425) -> (x+y=w1423:i32)
            n494 = call "Operation (SubVI).vi"("error in (no error)"=w1418, "On/Off"=w1415, "Operation"=w1413, "DAQmx Device Name"=w1417) -> ("error out"=w1431:errorcluster)  [unwired: 7 in]
            n495 = control-ref of="Motor Speed RPM Serial"() -> (w1432:refnum<vi>)
            n496 = control-ref of="Pannel User Message"() -> (w1434:refnum<vi>)
            n497 = control-ref of="Stop Button"() -> (w1437:refnum<vi>)
            n498 = call "Write panel message Kinetics (SubVI).vi"(4:"rpm"=w1432, 5:"rpm"=TRUE ("rpm"), "PrintTime"=TRUE, "Stop"=w1437, "error in (no error)"=w1431, "Time to wait"=30.0, "Strin"=w1416, "String in"=w1434) -> ("error out"=w1430:errorcluster, "Stopped"=w1414:bool)  [unwired: 2 in]
            n499 = property on="Motor Speed RPM Serial" class="DigNum (strict)"(error in=w1430) -> (error out=w1422:errorcluster, "Value"=w1421:dbl)  [unwired: 1 in, 1 out]
            n500 = Subtract(x=w1429, y=w1428) -> (x-y=w1426:i32)
            n501 = Add(x=w1428, y=w1429) -> (x+y=w1427:i32)
            n502 = In Range and Coerce(upper limit=w1427, x=w1421, lower limit=w1426) -> (In Range?=w1420:bool)  [unwired: 1 out]
            n503 = call "PassOrFail (SubVI).vi"("index (row)"=w1423, "error in (no error)"=w1422, "Data in"=w1421, "Pass?Fail"=w1420, "Table in"=w1419) -> ("error out"=w1407:errorcluster)  [unwired: 6 in]
            n504 = Build Array(w1410, w1409) -> (w1411:T12)
            n505 = for {
              tunnel: w1417 -> [w1443]
              tunnel: w1412 -> [w1442] mode=indexing
              tunnel: w1411 -> [w1441] mode=indexing
              tunnel: [w1439] -> w1408
              tunnel: w1407 -> [w1438]
              n506 = call "Operation (SubVI).vi"("error in (no error)"=w1438, "On/Off"=w1442, "Operation"=w1441, "DAQmx Device Name"=w1443) -> ("error out"=w1440:errorcluster)  [unwired: 7 in]
              n507 = call "Time Delay5"("error in (no error)"=w1440) -> ("error out"=w1439:errorcluster)  [unwired: 10 in]
            }
          }
          n508 = for {
            tunnel: w1368 -> [w1397]
            tunnel: w1380 -> [w1396] mode=indexing
            n509 = local read "DAQmx Device Name"() -> (w1398:tag)
            n510 = call "Operation (SubVI).vi"("error in (no error)"=w1397, "On/Off"=FALSE, "Operation"=w1396, "DAQmx Device Name"=w1398) -> ()  [unwired: 7 in, 1 out]
          }
        }
        frame "Resistance Merkava 3 Test" {
          w1445 = T12 [enum."0 ohm", enum."13.2 ohm", enum."33 ohm"] items=["Init", "0 ohm", "6 ohm", "13.2 ohm", "15 ohm", "25.9 ohm", "33 ohm", "Down", "Up", "Venable", "Firmware", "PowerSuply"]
          w1449 = T12 [enum."13.2 ohm", enum."33 ohm", enum."33 ohm"] items=["Init", "0 ohm", "6 ohm", "13.2 ohm", "15 ohm", "25.9 ohm", "33 ohm", "Down", "Up", "Venable", "Firmware", "PowerSuply"]
          w1452 = T12 [enum."PowerSuply", enum."Venable", enum."Up", enum."0 ohm", enum."PowerSuply"] items=["Init", "0 ohm", "6 ohm", "13.2 ohm", "15 ohm", "25.9 ohm", "33 ohm", "Down", "Up", "Venable", "Firmware", "PowerSuply"]
          w1457 = T12 [enum."Venable", enum."Up"] items=["Init", "0 ohm", "6 ohm", "13.2 ohm", "15 ohm", "25.9 ohm", "33 ohm", "Down", "Up", "Venable", "Firmware", "PowerSuply"]
          w1464 = T12 [enum."0 ohm", enum."13.2 ohm", enum."33 ohm"] items=["Init", "0 ohm", "6 ohm", "13.2 ohm", "15 ohm", "25.9 ohm", "33 ohm", "Down", "Up", "Venable", "Firmware", "PowerSuply"]
          # "6.5"
          n511 = control-ref of="Pannel User Message"() -> (w1471:refnum<vi>)
          n512 = Concatenate Strings(w1467, " in process..." ("Strin")) -> (w1458:string)
          n513 = property class="Str"(reference=w1471, error in=w1466, "Value"=w1458) -> (error out=w1470:errorcluster)  [unwired: 1 out]
          n514 = call "Table_ScrollaBarMarvin.vi"("error in"=w1470, "Line to focus"=w1467, "reference in"=w1460) -> ()  [unwired: 3 out]
          n515 = call "Reset old test Values (SubVI) Kinetics.vi"("Atr in"=w1460, "Test Paragraph"=w1467) -> ("error out"=w1469:errorcluster)  [unwired: 7 in, 2 out]
          n516 = call "Find_Number_LineMARVIN.vi"("Test Paragraph"=w1467, "error in"=w1469, "TableIn"=w1460) -> ("error out"=w1465:errorcluster, "Line number"=w1462:i32)  [unwired: 2 in, 2 out]
          n517 = for {
            tunnel: [w1481] -> w1459
            tunnel: w1465 -> [w1482]
            tunnel: [w1477] -> w1455
            tunnel: w1452 -> [w1480] mode=indexing
            tunnel: bool[] [FALSE, TRUE, TRUE, TRUE, TRUE] -> [w1479] mode=indexing
            tunnel: dbl[] [5.0, 0.2, 0.2, 0.2, 3.0] -> [w1476] mode=indexing
            n518 = local read "DAQmx Device Name"() -> (w1481:tag)
            n519 = call "Operation (SubVI).vi"("error in (no error)"=w1482, "On/Off"=w1479, "Operation"=w1480, "DAQmx Device Name"=w1481) -> ("error out"=w1478:errorcluster)  [unwired: 7 in]
            n520 = call "Time Delay7"("error in (no error)"=w1478, "Delay Time (s)"=w1476) -> ("error out"=w1477:errorcluster)  [unwired: 9 in]
          }
          n521 = Increment(x=w1462) -> (x+1=w1461:i32)
          n522 = call "Serial.vi"("error in (no error)"=w1455, "write buffer"="EP=1\r\nCF[0]=4.5\r\n", "VISA resource name"=w1456) -> ("error out"=w1454:errorcluster)  [unwired: 7 in, 1 out]
          n523 = for {
            tunnel: w1464 -> [w1494] mode=indexing
            tunnel: i32[] [6850, 9000, 9980] -> [w1505] mode=indexing
            tunnel: w1461 -> [w1500]
            tunnel: w1460 -> [w1495]
            tunnel: w1454 -> [w1493]
            tunnel: w1459 -> [w1492]
            tunnel: w1458 -> [w1491]
            tunnel: bool[] [FALSE, TRUE, TRUE] -> [w1490] mode=indexing
            tunnel: w1449 -> [w1487] mode=indexing
            tunnel: [w1489] -> w1447
            tunnel: bool[] [TRUE, FALSE] -> [w1488]
            tunnel: w1445 -> [w1486] mode=indexing
            tunnel: [w1484] -> w1444
            i -> [w1501]
            stop <- w1489 stop-if-true
            w1504 = 100 ("x")
            n524 = Add(x=w1500, y=w1501) -> (x+y=w1499:i32)
            n525 = call "Operation (SubVI).vi"("error in (no error)"=w1493, "On/Off"=w1490, "Operation"=w1494, "DAQmx Device Name"=w1492) -> ("error out"=w1507:errorcluster)  [unwired: 7 in]
            n526 = control-ref of="Motor Speed RPM Serial"() -> (w1508:refnum<vi>)
            n527 = control-ref of="Pannel User Message"() -> (w1510:refnum<vi>)
            n528 = control-ref of="Stop Button"() -> (w1513:refnum<vi>)
            n529 = call "Write panel message Kinetics (SubVI).vi"(4:"rpm"=w1508, 5:"rpm"=TRUE ("rpm"), "PrintTime"=TRUE, "Stop"=w1513, "error in (no error)"=w1507, "Time to wait"=30.0, "Strin"=w1491, "String in"=w1510) -> ("error out"=w1506:errorcluster, "Stopped"=w1489:bool)  [unwired: 2 in]
            n530 = property on="Motor Speed RPM Serial" class="DigNum (strict)"(error in=w1506) -> (error out=w1498:errorcluster, "Value"=w1497:dbl)  [unwired: 1 in, 1 out]
            n531 = Subtract(x=w1505, y=w1504) -> (x-y=w1502:i32)
            n532 = Add(x=w1504, y=w1505) -> (x+y=w1503:i32)
            n533 = In Range and Coerce(upper limit=w1503, x=w1497, lower limit=w1502) -> (In Range?=w1496:bool)  [unwired: 1 out]
            n534 = Build Array(w1487, w1486) -> (w1485:T12)
            n535 = call "PassOrFail (SubVI).vi"("index (row)"=w1499, "error in (no error)"=w1498, "Data in"=w1497, "Pass?Fail"=w1496, "Table in"=w1495) -> ("error out"=w1483:errorcluster)  [unwired: 6 in]
            n536 = for {
              tunnel: w1492 -> [w1519]
              tunnel: w1488 -> [w1518] mode=indexing
              tunnel: w1485 -> [w1517] mode=indexing
              tunnel: [w1515] -> w1484
              tunnel: w1483 -> [w1514]
              n537 = call "Operation (SubVI).vi"("error in (no error)"=w1514, "On/Off"=w1518, "Operation"=w1517, "DAQmx Device Name"=w1519) -> ("error out"=w1516:errorcluster)  [unwired: 7 in]
              n538 = call "Time Delay2"("error in (no error)"=w1516) -> ("error out"=w1515:errorcluster)  [unwired: 10 in]
            }
          }
          n539 = for {
            tunnel: w1444 -> [w1473]
            tunnel: w1457 -> [w1472] mode=indexing
            n540 = local read "DAQmx Device Name"() -> (w1474:tag)
            n541 = call "Operation (SubVI).vi"("error in (no error)"=w1473, "On/Off"=FALSE, "Operation"=w1472, "DAQmx Device Name"=w1474) -> ()  [unwired: 7 in, 1 out]
          }
        }
        frame "Resistance Namer Test" {
          w1521 = T12 [enum."13.2 ohm", enum."25.9 ohm", enum."33 ohm"] items=["Init", "0 ohm", "6 ohm", "13.2 ohm", "15 ohm", "25.9 ohm", "33 ohm", "Down", "Up", "Venable", "Firmware", "PowerSuply"]
          w1522 = T12 [enum."25.9 ohm", enum."33 ohm", enum."33 ohm"] items=["Init", "0 ohm", "6 ohm", "13.2 ohm", "15 ohm", "25.9 ohm", "33 ohm", "Down", "Up", "Venable", "Firmware", "PowerSuply"]
          w1528 = T12 [enum."Init", enum."PowerSuply", enum."Venable", enum."Down", enum."Up", enum."13.2 ohm", enum."PowerSuply", enum."Down", enum."Up"] items=["Init", "0 ohm", "6 ohm", "13.2 ohm", "15 ohm", "25.9 ohm", "33 ohm", "Down", "Up", "Venable", "Firmware", "PowerSuply"]
          w1533 = T12 [enum."Init", enum."Down", enum."Up"] items=["Init", "0 ohm", "6 ohm", "13.2 ohm", "15 ohm", "25.9 ohm", "33 ohm", "Down", "Up", "Venable", "Firmware", "PowerSuply"]
          w1539 = T12 [enum."13.2 ohm", enum."25.9 ohm", enum."33 ohm"] items=["Init", "0 ohm", "6 ohm", "13.2 ohm", "15 ohm", "25.9 ohm", "33 ohm", "Down", "Up", "Venable", "Firmware", "PowerSuply"]
          n542 = control-ref of="Pannel User Message"() -> (w1546:refnum<vi>)
          n543 = Concatenate Strings(w1542, " in process..." ("Strin")) -> (w1534:string)
          n544 = property class="Str"(reference=w1546, error in=w1541, "Value"=w1534) -> (error out=w1545:errorcluster)  [unwired: 1 out]
          n545 = call "Table_ScrollaBarMarvin.vi"("error in"=w1545, "Line to focus"=w1542, "reference in"=w1535) -> ()  [unwired: 3 out]
          n546 = call "Reset old test Values (SubVI) Kinetics.vi"("Atr in"=w1535, "Test Paragraph"=w1542) -> ("error out"=w1544:errorcluster)  [unwired: 7 in, 2 out]
          n547 = call "Find_Number_LineMARVIN.vi"("Test Paragraph"=w1542, "error in"=w1544, "TableIn"=w1535) -> ("error out"=w1540:errorcluster, "Line number"=w1537:i32)  [unwired: 2 in, 2 out]
          n548 = for {
            tunnel: [w1556] -> w1525
            tunnel: w1540 -> [w1557]
            tunnel: [w1553] -> w1532
            tunnel: w1528 -> [w1555] mode=indexing
            tunnel: dbl[] [1.0, 5.0, 0.2, 0.2, 0.2, 0.2, 5.0, 0.2, 0.2] -> [w1552] mode=indexing
            tunnel: bool[] [FALSE, FALSE, TRUE, TRUE, TRUE, TRUE, TRUE, TRUE, TRUE] -> [w1551] mode=indexing
            n549 = local read "DAQmx Device Name"() -> (w1556:tag)
            n550 = call "Operation (SubVI).vi"("error in (no error)"=w1557, "On/Off"=w1551, "Operation"=w1555, "DAQmx Device Name"=w1556) -> ("error out"=w1554:errorcluster)  [unwired: 7 in]
            n551 = call "Time Delay10"("error in (no error)"=w1554, "Delay Time (s)"=w1552) -> ("error out"=w1553:errorcluster)  [unwired: 9 in]
          }
          n552 = call "Serial.vi"("error in (no error)"=w1532, "write buffer"="EP=1\r\nCF[0]=4.5\r\n", "VISA resource name"=w1524) -> ("error out"=w1531:errorcluster)  [unwired: 7 in, 1 out]
          n553 = Increment(x=w1537) -> (x+1=w1536:i32)
          n554 = for {
            tunnel: w1539 -> [w1564] mode=indexing
            tunnel: i32[] [8350, 8900, 9450] -> [w1579] mode=indexing
            tunnel: w1536 -> [w1574]
            tunnel: w1535 -> [w1569]
            tunnel: w1531 -> [w1568]
            tunnel: w1525 -> [w1567]
            tunnel: w1534 -> [w1566]
            tunnel: [w1565] -> w1526
            tunnel: bool[] [TRUE, FALSE] -> [w1563]
            tunnel: w1522 -> [w1562] mode=indexing
            tunnel: w1521 -> [w1561] mode=indexing
            tunnel: [w1559] -> w1520
            i -> [w1575]
            stop <- w1565 stop-if-true
            w1578 = 100 ("x")
            n555 = Add(x=w1574, y=w1575) -> (x+y=w1573:i32)
            n556 = call "Operation (SubVI).vi"("error in (no error)"=w1568, "On/Off"=TRUE, "Operation"=w1564, "DAQmx Device Name"=w1567) -> ("error out"=w1581:errorcluster)  [unwired: 7 in]
            n557 = control-ref of="Motor Speed RPM Serial"() -> (w1582:refnum<vi>)
            n558 = control-ref of="Pannel User Message"() -> (w1584:refnum<vi>)
            n559 = control-ref of="Stop Button"() -> (w1587:refnum<vi>)
            n560 = call "Write panel message Kinetics (SubVI).vi"(4:"rpm"=w1582, 5:"rpm"=TRUE ("rpm"), "PrintTime"=TRUE, "Stop"=w1587, "error in (no error)"=w1581, "Time to wait"=30.0, "Strin"=w1566, "String in"=w1584) -> ("error out"=w1580:errorcluster, "Stopped"=w1565:bool)  [unwired: 2 in]
            n561 = property on="Motor Speed RPM Serial" class="DigNum (strict)"(error in=w1580) -> (error out=w1572:errorcluster, "Value"=w1571:dbl)  [unwired: 1 in, 1 out]
            n562 = Subtract(x=w1579, y=w1578) -> (x-y=w1576:i32)
            n563 = Add(x=w1578, y=w1579) -> (x+y=w1577:i32)
            n564 = In Range and Coerce(upper limit=w1577, x=w1571, lower limit=w1576) -> (In Range?=w1570:bool)  [unwired: 1 out]
            n565 = Build Array(w1562, w1561) -> (w1560:T12)
            n566 = call "PassOrFail (SubVI).vi"("index (row)"=w1573, "error in (no error)"=w1572, "Data in"=w1571, "Pass?Fail"=w1570, "Table in"=w1569) -> ("error out"=w1558:errorcluster)  [unwired: 6 in]
            n567 = for {
              tunnel: w1567 -> [w1594]
              tunnel: w1563 -> [w1593] mode=indexing
              tunnel: w1560 -> [w1592] mode=indexing
              tunnel: [w1590] -> w1559
              tunnel: w1558 -> [w1589]
              n568 = call "Operation (SubVI).vi"("error in (no error)"=w1589, "On/Off"=w1593, "Operation"=w1592, "DAQmx Device Name"=w1594) -> ("error out"=w1591:errorcluster)  [unwired: 7 in]
              n569 = call "Time Delay13"("error in (no error)"=w1591) -> ("error out"=w1590:errorcluster)  [unwired: 10 in]
            }
          }
          n570 = for {
            tunnel: w1520 -> [w1548]
            tunnel: w1533 -> [w1547] mode=indexing
            n571 = local read "DAQmx Device Name"() -> (w1549:tag)
            n572 = call "Operation (SubVI).vi"("error in (no error)"=w1548, "On/Off"=FALSE, "Operation"=w1547, "DAQmx Device Name"=w1549) -> ()  [unwired: 7 in, 1 out]
          }
        }
        frame "Analog Voltage Test" {
          w1602 = T12 [enum."Init", enum."PowerSuply"] items=["Init", "0 ohm", "6 ohm", "13.2 ohm", "15 ohm", "25.9 ohm", "33 ohm", "Down", "Up", "Venable", "Firmware", "PowerSuply"]
          w1626 = dbl[] [0.0, 1.0, 2.0, 3.0, 4.0, 4.5]
          n573 = control-ref of="Pannel User Message"() -> (w1634:refnum<vi>)
          n574 = Concatenate Strings(w1628, " in process..." ("string")) -> (w1608:string)
          n575 = property class="Str"(reference=w1634, error in=w1630, "Value"=w1608) -> (error out=w1633:errorcluster)  [unwired: 1 out]
          n576 = call "Table_ScrollaBarMarvin.vi"("error in"=w1633, "Line to focus"=w1628, "reference in"=w1629) -> ("error out"=w1632:errorcluster)  [unwired: 2 out]
          n577 = local read "DAQmx Device Name"() -> (w1600:tag)
          n578 = call "Find_Number_LineMARVIN.vi"("Test Paragraph"=w1628, "error in"=w1632, "TableIn"=w1629) -> ("error out"=w1636:errorcluster, "Line number"=w1635:i32)  [unwired: 2 in, 2 out]
          n579 = call <vilib>:"Clear Errors.vi"("error in (no error)"=w1636) -> ("error out"=w1627:errorcluster)  [unwired: 5 in, 1 out]
          n580 = call "Reset old test Values (SubVI) Kinetics.vi"("error in"=w1627, "Atr in"=w1629, "Test Paragraph"=w1628) -> ("error out"=w1616:errorcluster)  [unwired: 6 in, 2 out]
          n581 = for {
            tunnel: w1600 -> [w1641]
            tunnel: w1602 -> [w1640] mode=indexing
            tunnel: bool[] [FALSE, TRUE] -> [w1639] mode=indexing
            shift-right: [w1638] -> w1613
            shift-left: w1616 -> [w1642]
            n582 = call "Operation (SubVI).vi"("error in (no error)"=w1642, "On/Off"=w1639, "Operation"=w1640, "DAQmx Device Name"=w1641) -> ("error out"=w1638:errorcluster)  [unwired: 7 in]
          }
          n583 = control-ref of="Pannel User Message"() -> (w1615:refnum<vi>)
          n584 = control-ref of="Motor Speed RPM Serial"() -> (w1611:refnum<vi>)
          n585 = control-ref of="Stop Button"() -> (w1609:refnum<vi>)
          n586 = call "Write panel message Kinetics (SubVI).vi"(4:"rpm"=w1611, 5:"rpm"=FALSE ("rpm"), "PrintTime"=FALSE, "Stop"=w1609, "error in (no error)"=w1613, "Time to wait"=5.0, "Strin"=w1608, "String in"=w1615) -> ("error out"=w1607:errorcluster)  [unwired: 2 in, 1 out]
          n587 = local read "DAQmx Device Name"() -> (w1619:tag)
          n588 = call "Serial.vi"("error in (no error)"=w1607, "write buffer"="EP=1\r\nVC=0\r\n", "VISA resource name"=w1606) -> ("error out"=w1604:errorcluster)  [unwired: 7 in, 1 out]
          n589 = while {
            tunnel: [w1645] -> w1601
            tunnel: [TRUE] -> w1605
            tunnel: w1604 -> [w1643]
            stop <- w1647 stop-if-true
            n590 = control-ref of="Motor Speed RPM Serial"() -> (w1649:refnum<vi>)
            n591 = property class="DigNum (strict)"(reference=w1649, error in=w1643) -> (error out=w1645:errorcluster, "Value"=w1648:dbl)  [unwired: 1 out]
            n592 = Less Or Equal?(x=w1648, y=50.0) -> (x <= y?=w1647:bool)
          }
          "Analogtest" <- w1605
          n593 = call "Operation (SubVI).vi"("error in (no error)"=w1601, "On/Off"=FALSE, "Operation"=T5."PowerSuply", "DAQmx Device Name"=w1600) -> ("error out"=w1597:errorcluster)  [unwired: 7 in]
          n594 = call "Time Delay14"("error in (no error)"=w1597, "Delay Time (s)"=20.0) -> ("error out"=w1596:errorcluster)  [unwired: 9 in]
          n595 = for {
            tunnel: w1626 -> [w1660] mode=indexing
            tunnel: w1606 -> [w1659]
            tunnel: w1629 -> [w1658]
            tunnel: w1596 -> [w1653]
            tunnel: w1635 -> [w1657]
            tunnel: w1626 -> [w1656]
            tunnel: w1608 -> [w1655]
            tunnel: [w1653] -> w1625
            shift-right: [w1652] -> _
            shift-left: T10."Init" -> [w1661]
            tunnel: [w1651] -> w1620
            tunnel: w1619 -> [w1650]
            i -> [w1654]
            n596 = while {
              shift-right: [w1667] -> w1652
              shift-left: w1661 -> [w1673]
              tunnel: w1660 -> [w1672]
              tunnel: w1659 -> [w1671]
              tunnel: w1658 -> [w1670]
              tunnel: w1657 -> [w1669]
              tunnel: w1656 -> [w1668]
              tunnel: w1655 -> [w1666]
              tunnel: w1654 -> [w1665]
              tunnel: [w1663] -> w1651
              tunnel: w1650 -> [w1662]
              stop <- w1664 stop-if-true
              n597 = case shown="\"AI0/3\"" w1673 {
                tunnel: w1672 -> [_ w1678 w1713 w1719 _ _]
                tunnel: w1671 -> [_ _ _ _ _ w1740]
                tunnel: w1670 -> [_ w1685 _ _ _ w1762]
                tunnel: w1669 -> [_ w1684 _ _ _ w1761]
                tunnel: w1668 -> [_ _ _ _ _ w1760]
                tunnel: [T10."AO0" T10."Exit" T10."Wait" T10."AI0/3" T10."Read" w1744] -> w1667
                tunnel: [TRUE _ _ w1715 TRUE _] -> w1664
                tunnel: w1666 -> [_ _ _ w1723 _ _]
                tunnel: w1665 -> [_ w1679 _ _ _ _]
                tunnel: [_ _ _ w1715 _ _] -> w1663
                tunnel: w1662 -> [_ w1677 w1712 _ _ w1747]
                frame "Exit", Default {
                }
                frame "AI0/3" {
                  n598 = Increment(x=w1684) -> (x+1=w1683:i32)
                  n599 = property on="Motor Speed RPM Serial" class="DigNum (strict)"() -> ("Value"=w1687:dbl)  [unwired: 2 in, 2 out]
                  n600 = Multiply(x=w1679, y=2) -> (x*y=w1681:i32)
                  n601 = call "Aquire AI0"("device name"=w1677) -> ("data"=w1688:dynamicdata)  [unwired: 16 in, 2 out]
                  n602 = Add(x=w1683, y=w1681) -> (x+y=w1682:i32)
                  n603 = property on="Offset" class="DigNum (strict)" props=["Value"]() -> ()  [unwired: 2 in, 3 out]
                  n604 = To Double Precision Float(number=w1688) -> (double precision float=w1676:dbl)
                  n605 = Build Array(w1676, w1687) -> (w1686:dbl[])
                  n606 = for {
                    tunnel: w1686 -> [w1690] mode=indexing
                    tunnel: w1685 -> [w1695]
                    tunnel: w1682 -> [w1697]
                    tunnel: w1679 -> [w1693]
                    tunnel: w1678 -> [w1691]
                    i -> [w1694]
                    n607 = case shown="0, Default" w1694 {
                      tunnel: w1693 -> [_ w1705]
                      tunnel: [w1699 w1708] -> w1692
                      tunnel: w1691 -> [w1701 _]
                      tunnel: w1690 -> [w1698 w1707]
                      frame 0, Default {
                        w1700 = 0.2 ("y")
                        n608 = Add(x=w1700, y=w1701) -> (x+y=w1702:dbl)
                        n609 = Subtract(x=w1701, y=w1700) -> (x-y=w1703:dbl)
                        n610 = In Range and Coerce(upper limit=w1702, x=w1698, lower limit=w1703) -> (In Range?=w1699:bool)  [unwired: 1 out]
                      }
                      frame 1 {
                        w1709 = 200.0 ("y")
                        n611 = property on="SpeedLimit" class="Arr (strict)"() -> ("Value"=w1706:dbl[])  [unwired: 2 in, 2 out]
                        n612 = Index Array(array=w1706, index=w1705) -> (element=w1704:dbl)
                        n613 = Add(x=w1709, y=w1704) -> (x+y=w1710:dbl)
                        n614 = Subtract(x=w1704, y=w1709) -> (x-y=w1711:dbl)
                        n615 = In Range and Coerce(upper limit=w1710, x=w1707, lower limit=w1711) -> (In Range?=w1708:bool)  [unwired: 1 out]
                      }
                    }
                    n616 = Add(x=w1697, y=w1694) -> (x+y=w1696:i32)
                    n617 = call "PassOrFail (SubVI).vi"("index (row)"=w1696, "Data in"=w1690, "Pass?Fail"=w1692, "Table in"=w1695) -> ()  [unwired: 7 in, 1 out]
                  }
                }
                frame "AO0" {
                  n618 = call "Generate AO0"("data"=w1713, "device name"=w1712) -> ()  [unwired: 16 in, 2 out]
                }
                frame "Wait" {
                  n619 = Number To Fractional String(number=w1719, precision (6)=i16 1) -> (F-format string=w1717:string)  [unwired: 2 in]
                  n620 = Concatenate Strings(w1723, "\r\n", "Analog Output: ", w1717, "V." ("string")) -> (w1716:string)
                  n621 = control-ref of="Pannel User Message"() -> (w1725:refnum<vi>)
                  n622 = control-ref of="Motor Speed RPM Serial"() -> (w1724:refnum<vi>)
                  n623 = control-ref of="Stop Button"() -> (w1729:refnum<vi>)
                  n624 = call "Write panel message Kinetics (SubVI).vi"(4:"rpm"=w1724, 5:"rpm"=TRUE ("rpm"), "PrintTime"=TRUE, "Stop"=w1729, "Time to wait"=20.0, "Strin"=w1716, "String in"=w1725) -> ("Stopped"=w1715:bool)  [unwired: 3 in, 1 out]
                }
                frame "Read" {
                  n625 = One Button Dialog(message="No connection.") -> ()  [unwired: 1 in, 1 out]
                }
                frame "Init" {
                  w1754 = T12 [enum."PowerSuply", enum."Venable"] items=["Init", "0 ohm", "6 ohm", "13.2 ohm", "15 ohm", "25.9 ohm", "33 ohm", "Down", "Up", "Venable", "Firmware", "PowerSuply"]
                  n626 = for {
                    tunnel: w1754 -> [w1769] mode=indexing
                    tunnel: bool[] [TRUE, TRUE] -> [w1768] mode=indexing
                    tunnel: [w1767] -> w1734
                    tunnel: dbl[] [10.0, 2.0] -> [w1765] mode=indexing
                    tunnel: w1747 -> [w1764]
                    n627 = call "Operation (SubVI).vi"("On/Off"=w1768, "Operation"=w1769, "DAQmx Device Name"=w1764) -> ("error out"=w1766:errorcluster)  [unwired: 8 in]
                    n628 = call "Time Delay11"("error in (no error)"=w1766, "Delay Time (s)"=w1765) -> ("error out"=w1767:errorcluster)  [unwired: 9 in]
                  }
                  n629 = call "Aquire AI4"("error in"=w1734, "device name"=w1747) -> ("data"=w1748:dynamicdata, "error out"=w1736:errorcluster)  [unwired: 15 in, 1 out]
                  n630 = call "Serial.vi"("error in (no error)"=w1736, "write buffer"="AG[1]\r\n", "VISA resource name"=w1740) -> ("error out"=w1735:errorcluster, "read buffer"=w1739:string)  [unwired: 7 in]
                  n631 = Fract/Exp String To Number(string=w1739, default (0 dbl)=0.0 ("default (0 DBL)")) -> (number=w1737:dbl)  [unwired: 2 in, 1 out]
                  n632 = Equal To 0?(x=w1737) -> (x = 0?=w1746:bool)
                  n633 = for {
                    tunnel: w1740 -> [w1774]
                    tunnel: [w1770] -> w1756
                    tunnel: string[] ["EP=1\r\n", "VC=0\r\n", "CS[0]=0\r\n", "AG[1]\r\n"] -> [w1773] mode=indexing
                    tunnel: w1735 -> [w1771]
                    n634 = call "Time Delay3"("error in (no error)"=w1771) -> ("error out"=w1772:errorcluster)  [unwired: 10 in]
                    n635 = call "Serial.vi"("error in (no error)"=w1772, "write buffer"=w1773, "VISA resource name"=w1774) -> ("read buffer"=w1770:string)  [unwired: 7 in, 1 out]
                  }
                  n636 = Select(t=T10."Read", s=w1746, f=T10."AO0") -> (s? t:f=w1744:T10)
                  n637 = Fract/Exp String To Number(string=w1756, default (0 dbl)=sgl 0.0 ("default (0 DBL)")) -> (number=w1742:sgl)  [unwired: 2 in, 1 out]
                  n638 = To Double Precision Float(number=w1748) -> (double precision float=→"Offset":dbl)
                  n639 = Add(x=w1761, y=2) -> (x+y=w1759:i32)
                  n640 = for {
                    tunnel: w1762 -> [w1786]
                    tunnel: w1759 -> [w1785]
                    tunnel: w1760 -> [w1781] mode=indexing
                    tunnel: w1742 -> [w1782]
                    tunnel: [w1779] -> w1751
                    tunnel: [w1775] -> w1757 mode=indexing
                    i -> [w1777]
                    n641 = Multiply(x=w1777, y=2) -> (x*y=w1778:i32)
                    n642 = Multiply(x=w1782, y=w1781) -> (x*y=w1775:dbl)
                    n643 = Add(x=w1785, y=w1778) -> (x+y=w1784:i32)
                    n644 = Number To Fractional String(number=w1775, precision (6)=i16 1) -> (F-format string=w1780:string)  [unwired: 2 in]
                    n645 = call "InsertSingleData.vi"("String In"=w1780, "Col"=2, "Row"=w1784, "Table in"=w1786) -> ("error out"=w1779:errorcluster)  [unwired: 7 in]
                  }
                  "SpeedLimit" <- w1757
                  n646 = property on="Analogtest" class="Bool (strict)"(error in=w1751, "Value"=FALSE ("Analogtest")) -> ()  [unwired: 1 in, 2 out]
                }
              }
            }
          }
          n647 = local read "DAQmx Device Name"() -> (w1618:tag)
          n648 = call "Generate AO"("data"=0.0, "error in"=w1625, "device name"=w1618) -> ("error out"=w1621:errorcluster)  [unwired: 15 in, 1 out]
          n649 = call "Operation (SubVI).vi"("error in (no error)"=w1621, "On/Off"=FALSE, "Operation"=T5."Venable", "DAQmx Device Name"=w1618) -> ()  [unwired: 7 in, 1 out]
        }
        frame "Motor Run Test" {
          n650 = control-ref of="Pannel User Message"() -> (w1807:refnum<vi>)
          n651 = Concatenate Strings(w1789, " in process..." ("Strin")) -> (w1794:string)
          n652 = property class="Str"(reference=w1807, error in=w1804, "Value"=w1794) -> (error out=w1806:errorcluster)  [unwired: 1 out]
          n653 = call "Table_ScrollaBarMarvin.vi"("error in"=w1806, "Line to focus"=w1789, "reference in"=w1797) -> ()  [unwired: 3 out]
          n654 = call "Reset old test Values (SubVI) Kinetics.vi"("Atr in"=w1797, "Test Paragraph"=w1789) -> ("error out"=w1805:errorcluster)  [unwired: 7 in, 2 out]
          n655 = call "Find_Number_LineMARVIN.vi"("Test Paragraph"=w1789, "error in"=w1805, "TableIn"=w1797) -> ("error out"=w1802:errorcluster, "Line number"=w1796:i32)  [unwired: 2 in, 2 out]
          n656 = Increment(x=w1796) -> (x+1=w1795:i32)
          n657 = while {
            tunnel: w1802 -> [w1810]
            tunnel: w1790 -> [w1817]
            shift-right: [w1815] -> _
            shift-left: T11."Init" -> [w1816]
            tunnel: w1797 -> [w1814]
            tunnel: w1795 -> [w1813]
            tunnel: w1794 -> [w1811]
            tunnel: [w1810] -> w1791
            tunnel: [w1808] -> w1788
            i -> [w1812]
            stop <- w1809 stop-if-true
            n658 = case shown="\"ReadCurrent\"" w1816 {
              tunnel: w1810 -> [_ w1823 w1835 w1879 w1894]
              tunnel: w1817 -> [_ _ _ w1880 w1892]
              tunnel: [T11."Exit" T11."ReadTemp" w1832 T11."ReadCurrent" T11."ReadTemp"] -> w1815
              tunnel: w1814 -> [_ _ w1847 w1874 _]
              tunnel: w1813 -> [_ _ w1849 w1876 _]
              tunnel: w1812 -> [_ _ w1850 w1877 _]
              tunnel: w1811 -> [_ w1824 w1834 _ _]
              tunnel: [TRUE ("Stopped") w1820 w1833 _ _] -> w1809
              tunnel: [_ w1820 _ _ _] -> w1808
              frame "Exit", Default {
              }
              frame "Wait" {
                n659 = control-ref of="Motor Speed RPM Serial"() -> (w1829:refnum<vi>)
                n660 = control-ref of="Pannel User Message"() -> (w1828:refnum<vi>)
                n661 = control-ref of="Stop Button"() -> (w1827:refnum<vi>)
                n662 = call "Write panel message Kinetics (SubVI).vi"(4:"rpm"=w1829, 5:"rpm"=TRUE ("rpm"), "PrintTime"=TRUE, "Stop"=w1827, "error in (no error)"=w1823, "Time to wait"=1140.0, "Strin"=w1824, "String in"=w1828) -> ("Stopped"=w1820:bool)  [unwired: 2 in, 1 out]
              }
              frame "ReadCurrent" {
                w1845 = 3.0 ("x")
                n663 = control-ref of="Motor Speed RPM Serial"() -> (w1841:refnum<vi>)
                n664 = control-ref of="Pannel User Message"() -> (w1840:refnum<vi>)
                n665 = control-ref of="Stop Button"() -> (w1839:refnum<vi>)
                n666 = call "Write panel message Kinetics (SubVI).vi"(4:"rpm"=w1841, 5:"rpm"=TRUE ("rpm"), "PrintTime"=TRUE, "Stop"=w1839, "error in (no error)"=w1835, "Time to wait"=59.0, "Strin"=w1834, "String in"=w1840) -> ("error out"=w1830:errorcluster, "Stopped"=w1833:bool)  [unwired: 2 in]
                n667 = disable-structure shown="Disabled" {
                  disable-tunnel: w1830 -> [w1852 _]
                  frame Disabled {
                    n668 = property on="UUT" class="Str"() -> ("Value"=w1851:string)  [unwired: 2 in, 2 out]
                    n669 = case shown="\"Condenser India\", \"Condenser Merkava\"" w1851 {
                      tunnel: [w1853 w1855] -> _
                      tunnel: w1852 -> [_ w1856]
                      frame "Condenser India", "Condenser Merkava" {
                        n670 = call "Current prob"() -> ("Current"=w1853:dbl)  [unwired: 17 in, 2 out]
                      }
                      frame "True", Default {
                        n671 = local read "DAQmx Device Name"() -> (w1859:tag)
                        n672 = call "Aquire AI3"("error in"=w1856, "device name"=w1859) -> ("data"=w1858:dynamicdata)  [unwired: 15 in, 2 out]
                        n673 = To Double Precision Float(number=w1858) -> (double precision float=w1857:dbl)
                        n674 = Multiply(x=w1857, y=25.0) -> (x*y=w1855:dbl)
                      }
                    }
                  }
                  frame Enabled {
                  }
                }
                n675 = case shown="2, Default" w1850 {
                  tunnel: w1849 -> [w1862 w1865]
                  tunnel: [w1861 w1866] -> w1848
                  tunnel: [T11."Wait" T11."Exit"] -> w1832
                  frame 2, Default {
                    n676 = Increment(x=w1862) -> (x+1=w1861:i32)
                  }
                  frame 5 {
                    n677 = Add(x=w1865, y=3) -> (x+y=w1866:i32)
                  }
                }
                n678 = call "ValFromATR(SubVI).vi"("Row"=w1848, "Table in"=w1847) -> ("Val"=w1846:dbl)  [unwired: 8 in, 1 out]
                n679 = Add(x=w1845, y=w1846) -> (x+y=w1844:dbl)
                n680 = Subtract(x=w1846, y=w1845) -> (x-y=w1843:dbl)
                n681 = call "Current prob2"("error in (no error)"=w1830) -> ("Current"=w1831:dbl)  [unwired: 16 in, 2 out]
                n682 = In Range and Coerce(upper limit=w1844, x=w1831, lower limit=w1843) -> (In Range?=w1842:bool)  [unwired: 1 out]
                n683 = call "PassOrFail (SubVI).vi"("index (row)"=w1848, "Data in"=w1831, "Pass?Fail"=w1842, "Table in"=w1847) -> ()  [unwired: 7 in, 1 out]
              }
              frame "ReadTemp" {
                w1872 = 15.0 ("x")
                n684 = case shown="4" w1877 {
                  tunnel: w1876 -> [w1882 w1884]
                  tunnel: [w1882 w1885] -> w1875
                  frame 1, Default {
                  }
                  frame 4 {
                    n685 = Add(x=w1884, y=2) -> (x+y=w1885:i32)
                  }
                }
                n686 = call "Serial.vi"("error in (no error)"=w1879, "write buffer"="TA[1]\r\n", "VISA resource name"=w1880) -> ("read buffer"=w1878:string)  [unwired: 7 in, 1 out]
                n687 = call "ValFromATR(SubVI).vi"("Row"=w1875, "Table in"=w1874) -> ("Val"=w1873:dbl)  [unwired: 8 in, 1 out]
                n688 = Fract/Exp String To Number(string=w1878) -> (number=w1868:dbl)  [unwired: 3 in, 1 out]
                n689 = Add(x=w1872, y=w1873) -> (x+y=w1871:dbl)
                n690 = Subtract(x=w1873, y=w1872) -> (x-y=w1870:dbl)
                n691 = In Range and Coerce(upper limit=w1871, x=w1868, lower limit=w1870) -> (In Range?=w1869:bool)  [unwired: 1 out]
                n692 = call "PassOrFail (SubVI).vi"("index (row)"=w1875, "Data in"=w1868, "Pass?Fail"=w1869, "Table in"=w1874) -> ()  [unwired: 7 in, 1 out]
              }
              frame "Init" {
                n693 = property on="UUT" class="Str"(error in=w1894) -> (error out=w1891:errorcluster, "Value"=w1895:string)  [unwired: 1 in, 1 out]
                n694 = case shown="\"BLDC 60A\"" w1895 {
                  tunnel: ["EP=1\r\nVC=3700\r\n" ("write buffer") "EP=1\r\nVC=9980\r\n" ("write buffer") "EP=1\r\nCL[0]=55\r\nVC=11300\r\n" ("write buffer") "EP=1\r\n" ("write buffer")] -> w1893
                  frame "BLDC 30A", Default {
                  }
                  frame "BLDC 60A" {
                  }
                  frame "Warrior 60A" {
                  }
                  frame "Condenser India", "Condenser Merkava" {
                  }
                }
                n695 = call "Serial.vi"("error in (no error)"=w1891, "write buffer"=w1893, "VISA resource name"=w1892) -> ("error out"=w1886:errorcluster)  [unwired: 7 in, 1 out]
                n696 = local read "DAQmx Device Name"() -> (w1889:tag)
                n697 = call "Operation (SubVI).vi"("error in (no error)"=w1886, "On/Off"=TRUE, "Operation"=T5."Venable", "DAQmx Device Name"=w1889) -> ()  [unwired: 7 in, 1 out]
              }
            }
          }
          n698 = call "Serial.vi"("error in (no error)"=w1791, "write buffer"="EP=1\r\nVC=0\r\n", "VISA resource name"=w1790) -> ("error out"=w1792:errorcluster)  [unwired: 7 in, 1 out]
          n699 = local read "DAQmx Device Name"() -> (w1798:tag)
          n700 = call "Operation (SubVI).vi"("error in (no error)"=w1792, "On/Off"=FALSE, "Operation"=T5."Venable", "DAQmx Device Name"=w1798) -> ()  [unwired: 7 in, 1 out]
        }
        frame "Set Production Parameters" {
          n701 = control-ref of="Pannel User Message"() -> (w1914:refnum<vi>)
          n702 = Concatenate Strings(w1907, " in process..." ("Strin")) -> (w1911:string)
          n703 = property class="Str"(reference=w1914, error in=w1909, "Value"=w1911) -> (error out=w1913:errorcluster)  [unwired: 1 out]
          n704 = call "Table_ScrollaBarMarvin.vi"("error in"=w1913, "Line to focus"=w1907, "reference in"=w1905) -> ("error out"=w1908:errorcluster)  [unwired: 2 out]
          n705 = call "Reset old test Values (SubVI) Kinetics.vi"("error in"=w1908, "Atr in"=w1905, "Test Paragraph"=w1907) -> ("error out"=w1912:errorcluster)  [unwired: 6 in, 2 out]
          n706 = call "Find_Number_LineMARVIN.vi"("Test Paragraph"=w1907, "error in"=w1912, "TableIn"=w1905) -> ("error out"=w1904:errorcluster, "Line number"=w1902:i32)  [unwired: 2 in, 2 out]
          n707 = Increment(x=w1902) -> (x+1=w1901:i32)
          n708 = for {
            tunnel: w1906 -> [w1923]
            tunnel: w1905 -> [w1922]
            tunnel: w1904 -> [w1921]
            tunnel: string[] ["SN\r\n", "PN\r\n"] -> [w1919] mode=indexing
            tunnel: w1901 -> [w1916]
            i -> [w1917]
            n709 = call "Serial.vi"("error in (no error)"=w1921, "write buffer"=w1919, "VISA resource name"=w1923) -> ("error out"=w1920:errorcluster, "read buffer"=w1918:string)  [unwired: 7 in]
            n710 = Add(x=w1916, y=w1917) -> (x+y=w1915:i32)
            n711 = case shown="0, Default" w1917 {
              tunnel: w1922 -> [w1932 w1939]
              tunnel: w1920 -> [w1931 w1938]
              tunnel: w1918 -> [w1924 w1934]
              tunnel: w1915 -> [w1925 w1933]
              frame 0, Default {
                n712 = property on="Next SN" class="DigNum (strict)"() -> ("Value"=w1929:i32)  [unwired: 2 in, 2 out]
                n713 = Decrement(x=w1929) -> (x-1=w1930:i32)
                n714 = Number To Decimal String(number=w1930) -> (decimal integer string=w1928:string)  [unwired: 1 in]
                n715 = Equal?(x=w1924, y=w1928) -> (x = y?=w1927:bool)
                n716 = call "PassOrFail (SubVI).vi"("String Res"=w1924, "index (row)"=w1925, "error in (no error)"=w1931, "Data in"=-3.0, "Pass?Fail"=w1927, "Table in"=w1932) -> ()  [unwired: 5 in, 1 out]
              }
              frame 1 {
                n717 = property on="PN" class="Str"() -> ("Value"=w1937:string)  [unwired: 2 in, 2 out]
                n718 = Equal?(x=w1937, y=w1934) -> (x = y?=w1936:bool)
                n719 = call "PassOrFail (SubVI).vi"("String Res"=w1934, "index (row)"=w1933, "error in (no error)"=w1938, "Data in"=-3.0, "Pass?Fail"=w1936, "Table in"=w1939) -> ()  [unwired: 5 in, 1 out]
              }
            }
          }
        }
      }
      "TestinExecution" <- w235
    }
    n720 = flat-sequence {
      tunnel: w219 -> [_]
      frame #0 {
        w229 = T13."Enabled" ("Disabled")
        w230 = FALSE ("Start")
        n721 = local read "DAQmx Device Name"() -> (w228:tag)
        n722 = property on="Start" class="Bool (strict)"("Value"=w230, "DisabledEnum"=w229) -> ()  [unwired: 2 in, 2 out]
        n723 = property on="Report" class="Bool (strict)"("Value"=w230, "DisabledEnum"=w229) -> ()  [unwired: 2 in, 2 out]
        n724 = call "Operation (SubVI).vi"("On/Off"=FALSE, "Operation"=T5."PowerSuply", "DAQmx Device Name"=w228) -> ()  [unwired: 8 in, 1 out]
      }
    }
  }
  n725 = while {
    shift-right: [w1944] -> _
    shift-left: T3."Initialize" -> [w1963]
    shift-right: [w1960] -> _
    shift-left: _ -> [w1959]
    shift-right: [w1958] -> _
    shift-left: w28 -> [w1956]
    shift-right: [w1957] -> _
    shift-left: refnum<vi> refnum ("Config_CANAT") -> [w1955]
    shift-right: [w1953] -> _
    shift-left: w25 -> [w1954]
    tunnel: "ATR" -> [_]
    tunnel: w19 -> [w1952]
    tunnel: w18 -> [w1951]
    shift-right: [w1949] -> _
    shift-left: w2 -> [w1950]
    tunnel: w9 -> [w1948]
    tunnel: w3 -> [w1947]
    tunnel: w17 -> [_]
    tunnel: w26 -> [w1962]
    tunnel: [w1961] -> _
    tunnel: w10 -> [_]
    tunnel: w7 -> [w1945]
    shift-right: [w1942] -> _
    shift-left: w2 -> [w1943]
    shift-right: [w1940] -> _
    shift-left: w2 -> [w1941]
    stop <- w1946 stop-if-true
    n726 = case shown="\"Erase ATR Table\", Default" w1963 {
      tunnel: [T3."MainProgram" w2141 w2209 T3."Erase ATR Table"] -> w1944
      tunnel: [FALSE w2129 FALSE FALSE] -> w1946
      tunnel: [w2003 w2134 w2203 w2713] -> w1961
      tunnel: w1962 -> [_ w2106 w2207 _]
      tunnel: [w1967 refnum<visa-resource-name> refnum ("VISA resource name") w2204 w2737] -> w1960
      tunnel: w1959 -> [_ w2153 w2205 _]
      tunnel: [w2021 w2123 w2199 w2735] -> w1958
      tunnel: [w2006 refnum<vi> refnum ("Config_CANAT") w2200 w2722] -> w1957
      tunnel: w1956 -> [w2021 w2155 w2202 w2735]
      tunnel: w1955 -> [_ w2144 w2201 w2722]
      tunnel: w1954 -> [w2020 w2148 w2198 w2734]
      tunnel: [w2020 w2122 w2197 w2734] -> w1953
      tunnel: w1952 -> [_ _ w2196 _]
      tunnel: w1951 -> [_ _ w2195 _]
      tunnel: w1950 -> [w2018 w2146 w2194 w2732]
      tunnel: [w2018 w2146 w2193 w2732] -> w1949
      tunnel: w1948 -> [w2017 _ w2192 _]
      tunnel: w1947 -> [_ _ w2191 _]
      tunnel: w1945 -> [_ _ w2190 _]
      tunnel: w1943 -> [_ _ w2189 _]
      tunnel: [w2014 w2121 w2188 w2727] -> w1942
      tunnel: w1941 -> [_ _ w2187 _]
      tunnel: [w2014 w2121 w2186 w2727] -> w1940
      frame "Erase ATR Table", Default {
        w2005 = refnum<visa-resource-name> "COMx" ("VISA Kinetics")
        w2014 = 0
        w2016 = T13."Enabled" ("Disabled")
        w2023 = FALSE ("Visible")
        n727 = property on="Serial Com" class="Bool"(error in=errorcluster {"status"=FALSE, "code"=0, "source"=""} ("error out"), "Visible"=FALSE) -> (error out=w2019:errorcluster)  [unwired: 1 in, 1 out]
        n728 = property on="VISA Kinetics" class="VISAName"(error in=w2019, "Visible"=w2023, "Value"=w2005) -> (error out=w2025:errorcluster)  [unwired: 1 in, 1 out]
        n729 = property on="Serial Status" class="Bool (strict)"(error in=w2025, "Value"=w2023) -> (error out=w2012:errorcluster)  [unwired: 1 in, 1 out]
        n730 = property on="Pannel User Message" class="Str"(error in=w2012, "Value"="Select a UUT from list bellow:") -> (error out=w2011:errorcluster)  [unwired: 1 in, 1 out]
        n731 = call "UUT select.vi"("error constant"=w2011) -> ("error constant 2"=w1991:errorcluster, 2:"UUT Out"=w1966:string, 3:"UUT Out"=w2010:u16)  [unwired: 8 in]
        "UUT" <- w1966
        n732 = property on="Pannel User Message" class="Str"(error in=w1991, "Value"="Tester initialization in process..." ("Pannel User Message")) -> (error out=w1990:errorcluster)  [unwired: 1 in, 1 out]
        n733 = call "ATRBuild.vi"("error constant"=w1990, "UUT In"=w2010) -> ("error constant 2"=w2009:errorcluster, "TestArray"=→"TestArray":string[], "TestArray Out"=w2008:string[][])  [unwired: 7 in]
        n734 = for {
          tunnel: w2008 -> [w2092] mode=indexing
          tunnel: w2009 -> [w2090]
          tunnel: [w2089] -> w2015
          tunnel: w2008 -> [w2088]
          i -> [w2091]
          n735 = for {
            tunnel: w2092 -> [_] mode=indexing
            tunnel: w2091 -> [w2098]
            tunnel: w2090 -> [w2095]
            tunnel: [w2094] -> w2089
            tunnel: w2088 -> [w2093]
            i -> [w2099]
            n736 = Bundle By Name(cluster=T14 {"Row"=0, "Column"=0} ("Active Cell:Active Cell"), "Row"=w2098, "Column"=w2099) -> (w2097:T14)
            n737 = control-ref of="ATR"() -> (w2096:refnum<vi>)
            n738 = property class="Tbl (strict)"(reference=w2096, error in=w2095, "Active Cell"=w2097, "Cell BG Color"=u32 16777226, "Value"=w2093) -> (error out=w2094:errorcluster)  [unwired: 1 out]
          }
        }
        n739 = call "DataFrom_ini (SubVI).vi"("error in (no error)"=w2015, "UUT"=w1966, "appended path"=w2017) -> ("error out"=w1972:errorcluster, "FileName"=w2000:string, "Next SN"=w1982:i32, "UUT SoftwareVer"=w1981:string, "ParamVersion"=→"ParamVersion":string, "PN"=w1979:string)  [unwired: 3 in]
        "UUT SoftwareVer" <- w1981
        "Next SN" <- w1982
        "FileName" <- w2000
        "PN" <- w1979
        n740 = Decrement(x=w1982) -> (x-1=w1983:i32)
        n741 = Number To Decimal String(number=w1983) -> (decimal integer string=w1980:string)  [unwired: 1 in]
        n742 = control-ref of="ATR"() -> (w1996:refnum<vi>)
        n743 = Build Array(w1981, w1981, w1980, w1979) -> (w1978:string[])
        n744 = call "Boards S/N"("error in (no error)"=w1972) -> ("POWER Board S/N"=→"POWER Board S/N":string, "DSP Board S/N"=→"DSP Board S/N":string, "error out"=w1971:errorcluster)  [unwired: 15 in, 1 out]
        n745 = for {
          tunnel: w1971 -> [w2040]
          tunnel: w1996 -> [w2038]
          tunnel: string[] ["RS232 Comm. + Version", "CAN Comm.", "Unit Serial number", "Unit Part number"] -> [w2037] mode=indexing
          tunnel: [w2036] -> w1998
          tunnel: [w2035] -> w1977 mode=indexing
          tunnel: w1978 -> [w2034] mode=indexing
          n746 = call "Find_Number_LineMARVIN.vi"("Test Paragraph"=w2037, "error in"=w2040, "TableIn"=w2038) -> ("error out"=w2039:errorcluster, "Line number"=w2035:i32)  [unwired: 2 in, 2 out]
          n747 = call "InsertSingleData.vi"("String In"=w2034, "error in (no error)"=w2039, "Col"=2, "Row"=w2035, "Table in"=w2038) -> ("error out"=w2036:errorcluster)  [unwired: 6 in]
        }
        n748 = control-ref of="This VI"() -> (w1994:refnum<vi>)
        n749 = Index Array(array=w1977, index=1) -> (element=w1975:i32)
        n750 = call "COM UUT Board.vi"("error in (no error)"=w1998, "VI reference (current VI)"=w1994, "VISA resource name 2"=w2005) -> ("error out"=w2002:errorcluster, ".not. x?"=w1988:bool, "VISA resource name out"=w2001:refnum<visa-resource-name>)  [unwired: 6 in]
        "Serial Status" <- w1988
        n751 = case shown="True" w1988 {
          tunnel: w2002 -> [w2042 w2065]
          tunnel: w2001 -> [w2043 w2064]
          tunnel: [w2043 w2055] -> w1967
          tunnel: [w2042 w2049] -> w1969
          tunnel: w2000 -> [_ w2048]
          tunnel: w1981 -> [_ w2044]
          frame False {
          }
          frame True {
            n752 = VISA Flush I/O Buffer(VISA resource name=w2064, error in (no error)=w2065) -> (VISA resource name out=w2055:refnum<visa-resource-name>, error out=w2063:errorcluster)  [unwired: 1 in]
            n753 = call "Display Message to User2"("error in (no error)"=w2063) -> ("error out"=w2062:errorcluster, "Yes"=w2061:bool)  [unwired: 9 in]
            n754 = case shown="True" w2061 {
              tunnel: w2062 -> [w2066 w2087]
              tunnel: [w2066 w2067] -> w2060
              tunnel: w2055 -> [_ w2085]
              tunnel: w2048 -> [_ w2078]
              frame False {
              }
              frame True {
                w2071 = u16 11 items=["Init", "0 ohm", "6 ohm", "13.2 ohm", "15 ohm", "25.9 ohm", "33 ohm", "Down", "Up", "Venable", "Firmware", "PowerSuply"] ("Operation")
                w2076 = u16 11 items=["Init", "0 ohm", "6 ohm", "13.2 ohm", "15 ohm", "25.9 ohm", "33 ohm", "Down", "Up", "Venable", "Firmware", "PowerSuply"] ("Operation")
                n755 = local read "DAQmx Device Name"() -> (w2069:tag)
                n756 = call "SetParam.vi"("RS"=TRUE, "error in (no error)"=w2087, "Visa"=w2085, "Filein"=w2078) -> ("error out"=w2074:errorcluster)  [unwired: 7 in]
                n757 = call "Operation (SubVI).vi"("error in (no error)"=w2074, "On/Off"=FALSE, "Operation"=w2076, "DAQmx Device Name"=w2069) -> ("error out"=w2073:errorcluster)  [unwired: 7 in]
                n758 = control-ref of="Pannel User Message"() -> (w2084:refnum<vi>)
                n759 = control-ref of="Motor Speed RPM Serial"() -> (w2082:refnum<vi>)
                n760 = control-ref of="Stop Button"() -> (w2083:refnum<vi>)
                n761 = call "Write panel message Kinetics (SubVI).vi"(4:"rpm"=w2082, 5:"rpm"=FALSE ("rpm"), "PrintTime"=TRUE, "Stop"=w2083, "error in (no error)"=w2073, "Time to wait"=20.0, "Strin"="Restart the UUT\nPlease wait...", "String in"=w2084) -> ("error out"=w2070:errorcluster)  [unwired: 2 in, 1 out]
                n762 = call "Operation (SubVI).vi"("error in (no error)"=w2070, "On/Off"=TRUE, "Operation"=w2071, "DAQmx Device Name"=w2069) -> ("error out"=w2068:errorcluster)  [unwired: 7 in]
                n763 = call "Time Delay12"("error in (no error)"=w2068) -> ("error out"=w2067:errorcluster)  [unwired: 10 in]
              }
            }
            n764 = call "Serial.vi"("error in (no error)"=w2060, "write buffer"="SN\r\n", "VISA resource name"=w2055) -> ("error out"=w2056:errorcluster, "read buffer"=w2050:string)  [unwired: 7 in]
            n765 = property on="UUT SN Report" class="Str"("Value"=w2050) -> ()  [unwired: 2 in, 2 out]
            n766 = Decimal String To Number(string=w2050) -> (number=→"Current SN":i32)  [unwired: 2 in, 1 out]
            n767 = call "Serial.vi"("error in (no error)"=w2056, "write buffer"="VR\r\n", "VISA resource name"=w2055) -> ("error out"=w2051:errorcluster, "read buffer"=w2045:string)  [unwired: 7 in]
            n768 = control-ref of="ATR"() -> (w2052:refnum<vi>)
            n769 = call "Find_Number_LineMARVIN.vi"("Test Paragraph"="RS232 Comm. + Version", "TableIn"=w2052) -> ("Line number"=w2053:i32)  [unwired: 3 in, 3 out]
            n770 = Equal?(x=w2045, y=w2044) -> (x = y?=w2046:bool)
            n771 = call "PassOrFail (SubVI).vi"("String Res"=w2045, "index (row)"=w2053, "error in (no error)"=w2051, "Data in"=-3.0, "Pass?Fail"=w2046, "Table in"=w2052) -> ("error out"=w2049:errorcluster)  [unwired: 5 in]
          }
        }
        n772 = case shown="\"Condenser India\", \"Condenser Merkava\"" w1966 {
          tunnel: w1969 -> [w2029 w2032]
          tunnel: [w2029 w2031] -> w1968
          tunnel: w1967 -> [_ w2030]
          frame "False", Default {
          }
          frame "Condenser India", "Condenser Merkava" {
            n773 = call "Serial.vi"("error in (no error)"=w2032, "write buffer"="EP=1\r\nVC=1000\r\n", "VISA resource name"=w2030) -> ("error out"=w2031:errorcluster)  [unwired: 7 in, 1 out]
          }
        }
        n774 = call "KineticsCan.vi"("error in"=w1968) -> ("error out"=w1997:errorcluster, "Version"=w1992:string, "Res_Pass_T"=w1965:bool, "Config_CANAT_out"=w2006:refnum<vi>)  [unwired: 7 in]
        n775 = case shown="\"Condenser India\", \"Condenser Merkava\"" w1966 {
          tunnel: w1965 -> [w2027 _]
          tunnel: [w2027 TRUE ("Res_Pass_T")] -> w1964
          frame "False", Default {
          }
          frame "Condenser India", "Condenser Merkava" {
          }
        }
        "CAN Status" <- w1964
        n776 = Equal?(x=w1992, y=w1981) -> (x = y?=w1993:bool)
        n777 = call "PassOrFail (SubVI).vi"("String Res"=w1992, "index (row)"=w1975, "error in (no error)"=w1997, "Data in"=-3.0, "Pass?Fail"=w1993, "Table in"=w1996) -> ("error out"=w1987:errorcluster)  [unwired: 5 in]
        n778 = property on="Pannel User Message" class="Str"(error in=w1987, "Value"="You can press start to execute(s) test(s)." ("Pannel User Message")) -> (error out=w1986:errorcluster)  [unwired: 1 in, 1 out]
        n779 = property on="Start" class="Bool (strict)"(error in=w1986, "DisabledEnum"=w2016) -> (error out=w2004:errorcluster)  [unwired: 1 in, 1 out]
        n780 = property on="Report" class="Bool (strict)"(error in=w2004, "DisabledEnum"=w2016) -> (error out=w2003:errorcluster)  [unwired: 1 in, 1 out]
      }
      frame "Stop" {
        w2121 = 0
        n781 = control-ref of="ATR"() -> (w2120:refnum<vi>)
        n782 = call "PassFailUUT (SubVI).vi"("error in (no error)"=w2106, "Table in"=w2120) -> ("PassFaileUUTresult"=w2113:bool)  [unwired: 7 in, 2 out]
        n783 = property on="Test Failed" class="Bool (strict)"("Value"=w2113) -> ()  [unwired: 2 in, 2 out]
        n784 = flat-sequence {
          tunnel: w2106 -> [w2183]
          tunnel: [w2182] -> w2145
          frame #0 {
            n785 = control-ref of="Pannel User Message"() -> (w2185:refnum<vi>)
            n786 = property class="Str"(reference=w2185, error in=w2183, "Value"="Program Stopped...\r\nPlease turn OFF All Power sinks") -> (error out=w2182:errorcluster)  [unwired: 1 out]
          }
        }
        n787 = Select(t="PASS" ("name or relative path"), s=w2113, f="FAIL" ("name or relative path")) -> (s? t:f=w2112:string)
        n788 = call <vilib>:"Application Directory.vi"() -> ("Application Directory"=w2116:path)
        n789 = Build Path(base path=w2116, name or relative path="data\\TestResult.ini") -> (appended path=w2119:path)
        n790 = call <vilib>:"Open Config Data.vi"("configuration file path"=w2119) -> ("error out"=w2117:errorcluster, "refnum"=w2118:T4)  [unwired: 2 in, 7 out]
        n791 = call-poly <vilib>:"Write Key.vi"("section"="Kinetics", "error in (no error)"=w2117, "value"=w2112, "key"="Result", "refnum"=w2118) -> ("error out"=w2115:errorcluster, "refnum out"=w2114:T4)  [unwired: 4 in, 1 out]
        n792 = call <vilib>:"Close Config Data.vi"("error in (no error)"=w2115, "refnum"=w2114) -> ()  [unwired: 8 in, 2 out]
        n793 = disable-structure shown="Enabled" {
          disable-tunnel: w2145 -> [w2170 w2171]
          disable-tunnel: w2144 -> [w2168 _]
          disable-tunnel: [w2167 w2171] -> w2133
          frame Disabled {
            n794 = call "Clear CAN Buffer.vi"("error in (no error)"=w2170, "Cluster in"=w2168) -> ("error out"=w2169:errorcluster)  [unwired: 8 in, 1 out]
            n795 = call "Close CAN Device.vi"("error in (no error)"=w2169, "Cluster in"=w2168) -> ("error out"=w2167:errorcluster)  [unwired: 8 in, 1 out]
          }
          frame Enabled {
          }
        }
        n796 = local read "DAQmx Device Name"() -> (w2105:tag)
        n797 = VISA Close(VISA resource name=w2153, error in (no error)=w2145) -> (error out=w2147:errorcluster)
        n798 = property on="Stop Button" class="Bool (strict)"() -> ("Value"=w2125:bool)  [unwired: 2 in, 2 out]
        n799 = call "Operation (SubVI).vi"("On/Off"=FALSE, "Operation"=T5."Init", "DAQmx Device Name"=w2105) -> ("error out"=w2102:errorcluster)  [unwired: 8 in]
        n800 = property on="ClosePanel" class="Bool (strict)"() -> ("Value"=w2126:bool)  [unwired: 2 in, 2 out]
        n801 = Or(x=w2126, y=w2125) -> (x .or. y?=w2124:bool)
        n802 = Flush Queue(queue=w2148, error in (no error)=w2147) -> (queue out=w2150:refnum<queue>, error out=w2149:errorcluster)  [unwired: 1 out]
        n803 = Flush Queue(queue=w2155, error in (no error)=w2147) -> (queue out=w2154:refnum<queue>, error out=w2156:errorcluster)  [unwired: 1 out]
        n804 = case shown="False" w2124 {
          tunnel: w2156 -> [w2158 w2166]
          tunnel: w2154 -> [w2160 w2162]
          tunnel: w2150 -> [w2159 w2161]
          tunnel: w2149 -> [w2157 w2165]
          tunnel: [w2158 w2164] -> w2140
          tunnel: [w2157 w2163] -> w2139
          tunnel: [w2160 w2162] -> w2123
          tunnel: [w2159 w2161] -> w2122
          frame False {
          }
          frame True {
            n805 = Release Queue(queue=w2161, error in (no error)=w2165) -> (error out=w2163:errorcluster)  [unwired: 1 in, 2 out]
            n806 = Release Queue(queue=w2162, error in (no error)=w2166) -> (error out=w2164:errorcluster)  [unwired: 1 in, 2 out]
          }
        }
        n807 = Merge Errors(w2140, w2139, w2133, w2102) -> (w2138:errorcluster)
        n808 = property on="Refresh Button" class="Bool (strict)"() -> ("Value"=w2127:bool)  [unwired: 2 in, 2 out]
        n809 = call <vilib>:"Clear Errors.vi"("error in (no error)"=w2138) -> ("error out"=w2137:errorcluster)  [unwired: 5 in, 1 out]
        n810 = property on="Stop Button" class="Bool (strict)"() -> ("Value"=w2131:bool)  [unwired: 2 in, 2 out]
        n811 = property on="ClosePanel" class="Bool (strict)"(error in=w2137) -> (error out=w2135:errorcluster, "Value"=w2136:bool)  [unwired: 1 in, 1 out]
        n812 = Not(x=w2127) -> (.not. x?=w2128:bool)
        n813 = Select(t=T3."Initialize", s=w2127, f=T3."Stop") -> (s? t:f=w2141:T3)
        n814 = Not(x=w2131) -> (.not. x?=w2130:bool)
        n815 = Compound Arithmetic op=AND(w2136, w2130, w2128) -> (w2132:bool)
        n816 = case shown="False" w2132 {
          tunnel: w2135 -> [w2174 w2178]
          tunnel: [w2174 w2178] -> w2134
          tunnel: [w2173 w2177] -> w2129
          tunnel: w2127 -> [w2172 _]
          frame False {
            n817 = case shown="False" w2172 {
              tunnel: [TRUE FALSE] -> w2173
              frame False {
              }
              frame True {
              }
            }
          }
          frame True {
            n818 = flat-sequence {
              tunnel: [TRUE] -> w2177
              frame #0 {
              }
              frame #1 {
                n819 = control-ref of="This VI"() -> (w2181:refnum<vi>)
                n820 = property class="VI"(reference=w2181, "FP.State"=T15."Closed" ("Front Panel Window:State")) -> ()  [unwired: 1 in, 2 out]
              }
            }
          }
        }
      }
      frame "MainProgram" {
        n821 = event shown="[0] Timeout" {
          selector: w2196 -> [_ _ _ _ _ _ _ _ _ _ _ _ _]
          dyn-events: _ -> [_ _ _ _ _ _ _ _ _ _ _ _ _]
          timeout: "EventTimeout" -> [_ _ _ _ _ _ _ _ _ _ _ _ _]
          tunnel: [T3."MainProgram" T3."MainProgram" T3."MainProgram" T3."MainProgram" T3."MainProgram" T3."Stop" T3."MainProgram" w2552 T3."MainProgram" T3."MainProgram" T3."MainProgram" T3."Stop" T3."MainProgram"] -> w2209
          tunnel: [w2218 w2325 w2393 w2402 w2413 w2433 w2448 w2598 w2661 w2676 _ w2698 w2699] -> w2203
          tunnel: w2207 -> [w2224 w2325 w2392 w2404 w2413 w2433 _ w2598 w2662 w2675 w2683 w2698 w2699]
          tunnel: [w2215 w2319 w2394 w2403 w2414 w2431 w2440 w2557 w2659 w2673 _ w2696 w2703] -> w2204
          tunnel: w2205 -> [w2215 w2319 w2394 w2403 w2414 w2431 w2440 w2557 w2659 w2673 _ w2696 w2703]
          tunnel: w2202 -> [w2226 w2331 w2388 w2399 w2410 w2430 w2451 w2582 w2658 w2672 w2687 w2695 w2706]
          tunnel: w2201 -> [w2222 w2330 w2389 w2400 w2411 w2429 w2444 w2581 w2657 w2671 w2686 w2694 w2702]
          tunnel: [w2223 w2330 w2389 w2400 w2411 w2429 w2444 w2581 w2657 w2671 w2686 w2694 w2702] -> w2200
          tunnel: [w2225 w2331 w2388 w2399 w2410 w2430 w2451 w2582 w2658 w2672 w2687 w2695 w2706] -> w2199
          tunnel: w2198 -> [w2220 w2329 w2387 w2398 w2409 w2428 w2450 w2580 w2656 w2670 w2685 w2693 w2705]
          tunnel: [w2220 w2329 w2387 w2398 w2409 w2428 w2447 w2580 w2656 w2670 w2685 w2693 w2705] -> w2197
          tunnel: w2195 -> [_ _ _ _ _ _ _ w2535 _ _ _ _ _]
          tunnel: w2194 -> [w2221 w2328 w2386 w2397 w2408 w2426 w2445 w2561 w2655 w2669 w2684 w2692 w2704]
          tunnel: [w2221 w2328 w2386 w2397 w2408 w2426 w2445 w2560 w2655 w2669 w2684 w2692 w2704] -> w2193
          tunnel: w2192 -> [_ w2326 _ _ _ _ _ w2559 _ _ _ _ _]
          tunnel: w2191 -> [_ w2318 _ _ _ _ _ _ _ _ _ _ _]
          tunnel: w2190 -> [_ _ _ _ _ _ _ _ w2654 _ _ _ _]
          tunnel: w2189 -> [_ w2307 w2385 w2396 w2407 w2423 w2443 w2536 w2652 w2668 w2681 w2691 w2701]
          tunnel: [_ w2307 w2385 w2396 w2407 w2423 w2443 w2536 w2652 w2668 w2681 w2691 w2701] -> w2188
          tunnel: w2187 -> [w2217 w2306 w2384 w2395 w2406 w2422 w2442 w2528 w2651 w2667 w2680 w2690 w2700]
          tunnel: [w2216 w2306 w2384 w2395 w2406 w2422 w2442 w2528 w2651 w2667 w2680 w2690 w2700] -> w2186
          event Timeout {
            n822 = event-data() -> ()  [unwired: 1 in, 3 out]
            n823 = disable-structure shown="Enabled" {
              disable-tunnel: w2226 -> [w2243 w2300]
              disable-tunnel: [w2242 w2300] -> w2225
              disable-tunnel: w2224 -> [w2241 w2299]
              disable-tunnel: [w2240 w2297] -> w2223
              disable-tunnel: w2222 -> [w2239 w2297]
              disable-tunnel: [w2236 w2299] -> w2218
              disable-tunnel: w2217 -> [w2234 w2298]
              disable-tunnel: [w2233 w2298] -> w2216
              frame Disabled {
                n824 = property class="Clust (strict)"(reference=w2239, error in=w2241) -> (reference out=w2240:refnum<vi>, error out=w2235:errorcluster, "Value"=w2246:T24)
                n825 = Unbundle By Name(w2246) -> ("DevType"=w2247:T18, "CanIndex"=w2245:T19)
                n826 = call "VCI_Receive.vi"("CANIndex"=w2245, "DevIndex"=u32 0, "DevType"=w2247) -> ("Recieve"=w2244:T25[])  [unwired: 3 in, 5 out]
                n827 = Empty Array?(array=w2244) -> (empty?=w2238:bool)
                n828 = case shown="False" w2238 {
                  tunnel: w2245 -> [w2261 _]
                  tunnel: w2240 -> [w2259 _]
                  tunnel: w2243 -> [w2258 w2291]
                  tunnel: w2235 -> [w2257 w2290]
                  tunnel: w2244 -> [w2262 _]
                  tunnel: [w2252 w2290] -> w2236
                  tunnel: [w2251 w2291] -> w2242
                  tunnel: [TRUE w2285] -> w2237
                  tunnel: w2234 -> [_ w2289]
                  tunnel: [0 w2288] -> w2233
                  frame False {
                    n829 = call "Demo_MakeDispBuff.vi"("Channel"=w2261, "Type"=enum16{"接收", "发送"}."接收", "OBJs"=w2262) -> ("Buffer"=w2260:T26)
                    n830 = for {
                      N: 3 -> [_]
                      tunnel: w2260 -> [w2276]
                      tunnel: w2259 -> [w2275]
                      tunnel: w2258 -> [w2266]
                      tunnel: w2257 -> [w2265]
                      tunnel: [w2268] -> w2255 mode=indexing
                      tunnel: [w2266] -> w2254
                      tunnel: [w2265] -> w2253
                      i -> [w2264]
                      n831 = property class="Clust (strict)"(reference=w2275) -> ("Value"=w2273:T24)  [unwired: 1 in, 2 out]
                      n832 = Index Array(array=w2276, index=w2264) -> (element=w2269:T27)
                      n833 = Unbundle By Name(w2269) -> ("Channel"=w2271:T19, "VCI_CAN_OBJ"=w2274:T25)  [unwired: 2 out]
                      n834 = Unbundle By Name(w2273) -> ("CanIndex"=w2272:T19)
                      n835 = Equal?(x=w2272, y=w2271) -> (x = y?=w2270:bool)
                      n836 = case shown="True" w2270 {
                        tunnel: w2274 -> [_ w2284]
                        tunnel: [w2277 w2280] -> w2268
                        tunnel: T16 {"ID"=0, "MSGTYPE"=0, "LEN"=0, "aDATA"=[]} ("Msg") -> [w2277 w2279]
                        frame False {
                        }
                        frame True {
                          n837 = Unbundle By Name(w2284) -> ("ID"=w2278:u32, "DataLen"=w2283:u8, "Data"=w2281:u8[])
                          n838 = Bundle By Name(cluster=w2279, "ID"=w2278, "MSGTYPE"=u8 0, "LEN"=w2283, "aDATA"=w2281) -> (w2280:T16)
                        }
                      }
                    }
                    n839 = Enqueue Element(queue=w2254, element=w2255, error in (no error)=w2253) -> (queue out=w2251:refnum<queue>, error out=w2252:errorcluster)  [unwired: 2 out]
                  }
                  frame True {
                    n840 = Increment(x=w2289) -> (x+1=w2288:i32)
                    n841 = Greater Or Equal?(x=w2288, y=7) -> (x >= y?=w2286:bool)
                    n842 = Not(x=w2286) -> (.not. x?=w2285:bool)
                  }
                }
                n843 = property on="CAN Status" class="Bool (strict)"("Value"=w2237) -> ()  [unwired: 2 in, 2 out]
              }
              frame Enabled {
                n844 = control-ref of="ATR"() -> (w2292:refnum<vi>)
                n845 = call "PassFailUUT (SubVI).vi"("Table in"=w2292) -> ("PassFaileUUTresult"=w2293:bool)  [unwired: 8 in, 2 out]
                n846 = property on="Test Failed" class="Bool (strict)"("Value"=w2293) -> ()  [unwired: 2 in, 2 out]
                n847 = property on="Automation" class="Bool (strict)"() -> ("Value"=w2296:bool)  [unwired: 2 in, 2 out]
                n848 = property on="Start" class="Bool (strict)"() -> ("Value"=w2294:bool)  [unwired: 2 in, 2 out]
                n849 = Or(x=w2296, y=w2294) -> (x .or. y?=w2295:bool)
                n850 = case shown="False" w2295 {
                  frame False {
                    n851 = property on="Pannel User Message" class="Str"("Value"="You can press start to execute(s) test(s).") -> ()  [unwired: 2 in, 2 out]
                  }
                  frame True {
                  }
                }
              }
            }
            n852 = property on="ClosePanel" class="Bool (strict)"("Value"=FALSE ("ClosePanel")) -> ()  [unwired: 2 in, 2 out]
            n853 = Not Equal?(x=w2215, y=refnum<visa-resource-name> "COMx") -> (x != y?=w2213:bool)
            n854 = property on="Analogtest" class="Bool (strict)"() -> ("Value"=w2211:bool)  [unwired: 2 in, 2 out]
            n855 = Not(x=w2211) -> (.not. x?=w2210:bool)
            n856 = And(x=w2210, y=w2213) -> (x .and. y?=w2212:bool)
            n857 = case shown="True" w2212 {
              tunnel: w2215 -> [_ w2232]
              frame False {
              }
              frame True {
                n858 = call "Serial.vi"("Clear Log"=FALSE, "write buffer"="VC\r\n", "VISA resource name"=w2232) -> ("read buffer"=w2228:string)  [unwired: 7 in, 1 out]
                n859 = Fract/Exp String To Number(string=w2228) -> (number=→"Motor Speed RPM Serial":dbl)  [unwired: 3 in, 1 out]
              }
            }
          }
          event "SetSN": Value Change {
            n860 = event-data() -> ()  [unwired: 1 in, 6 out]
            n861 = property on="UUT" class="Str"() -> ("Value"=w2305:string)  [unwired: 2 in, 2 out]
            n862 = case shown="\"BLDC 30A\", Default" w2305 {
              tunnel: [26 26 26 26 35] -> w2303
              frame "BLDC 30A", Default {
              }
              frame "Warrior 60A" {
              }
              frame "Condenser Merkava" {
              }
              frame "Condenser India" {
              }
              frame "BLDC 60A" {
              }
            }
            n863 = control-ref of="ATR"() -> (w2310:refnum<vi>)
            n864 = property on="Current SN" class="DigNum (strict)"(error in=w2325) -> (error out=w2309:errorcluster, "Value"=w2324:i32)  [unwired: 1 in, 1 out]
            n865 = call "PassFailUUT (SubVI).vi"("error in (no error)"=w2309, "Table in"=w2310) -> ("Total Pass"=w2304:u8)  [unwired: 7 in, 2 out]
            n866 = Equal To 0?(x=w2324) -> (x = 0?=w2321:bool)
            n867 = Equal?(x=w2324, y=-1) -> (x = y?=w2322:bool)
            n868 = Equal?(x=w2304, y=w2303) -> (x = y?=w2302:bool)
            n869 = Or(x=w2322, y=w2321) -> (x .or. y?=w2320:bool)
            n870 = property on="CAN Status" class="Bool (strict)"() -> ("Value"=w2311:bool)  [unwired: 2 in, 2 out]
            n871 = property on="Serial Status" class="Bool (strict)"() -> ("Value"=w2316:bool)  [unwired: 2 in, 2 out]
            n872 = And(x=w2316, y=w2311) -> (x .and. y?=w2312:bool)
            n873 = case shown="True" w2312 {
              tunnel: w2326 -> [_ w2350]
              tunnel: w2320 -> [_ w2339]
              tunnel: w2319 -> [_ w2349]
              tunnel: w2318 -> [_ w2348]
              tunnel: [errorcluster {"status"=FALSE, "code"=0, "source"=""} ("error out") w2347] -> w2315
              tunnel: [w2337 w2346] -> w2317
              tunnel: w2302 -> [_ w2340]
              frame False {
                w2337 = FALSE ("Value")
                n874 = property on="SetSN" class="Bool (strict)"("Value"=w2337) -> ()  [unwired: 2 in, 2 out]
                n875 = call "Display Message to User10"() -> ()  [unwired: 10 in, 2 out]
              }
              frame True {
                n876 = property on="Test Failed" class="Bool (strict)"() -> ("Value"=w2344:bool)  [unwired: 2 in, 2 out]
                n877 = property on="Automation" class="Bool (strict)"() -> ("Value"=w2346:bool)  [unwired: 2 in, 2 out]
                n878 = Not(x=w2344) -> (.not. x?=w2345:bool)
                n879 = Select(t=w2345, s=w2346, f=w2348) -> (s? t:f=w2342:bool)
                n880 = Or(x=w2340, y=w2342) -> (x .or. y?=w2341:bool)
                n881 = And(x=w2339, y=w2341) -> (x .and. y?=w2343:bool)
                n882 = case shown="True" w2343 {
                  tunnel: w2350 -> [_ w2381]
                  tunnel: w2349 -> [_ w2374]
                  tunnel: [w2352 w2366] -> w2347
                  tunnel: w2339 -> [w2351 _]
                  frame False {
                    n883 = case shown="True" w2351 {
                      tunnel: [w2354 w2355] -> w2352
                      frame False {
                        n884 = call "Display Message to User9"() -> ("error out"=w2354:errorcluster)  [unwired: 10 in, 1 out]
                      }
                      frame True {
                        n885 = call "Display Message to User3"() -> ("error out"=w2355:errorcluster)  [unwired: 10 in, 1 out]
                      }
                    }
                    n886 = property on="Automation" class="Bool (strict)"(error in=w2352, "Value"=FALSE ("Automation")) -> ()  [unwired: 1 in, 2 out]
                  }
                  frame True {
                    w2373 = FALSE ("SetSN")
                    n887 = local read "DAQmx Device Name"() -> (w2359:tag)
                    n888 = property on="Next SN" class="DigNum (strict)"() -> ("Value"=w2361:i32)  [unwired: 2 in, 2 out]
                    n889 = call "Operation (SubVI).vi"("On/Off"=FALSE, "Operation"=T5."Venable", "DAQmx Device Name"=w2359) -> ("error out"=w2363:errorcluster)  [unwired: 8 in]
                    n890 = call <vilib>:"Clear Errors.vi"("error in (no error)"=w2363) -> ("error out"=w2364:errorcluster)  [unwired: 5 in, 1 out]
                    n891 = Number To Decimal String(number=w2361) -> (decimal integer string=w2362:string)  [unwired: 1 in]
                    "UUT SN Report" <- w2362
                    n892 = Search and Replace String(input string="EP=1\r\nSN=0\r\n" ("write buffer"), search string="0", replace string=w2362) -> (result string=w2376:string)  [unwired: 5 in, 3 out]
                    n893 = call "Serial.vi"("error in (no error)"=w2364, "Clear Log"=FALSE, "write buffer"=w2376, "VISA resource name"=w2374) -> ("error out"=w2358:errorcluster)  [unwired: 6 in, 1 out]
                    n894 = property on="UUT" class="Str"(error in=w2358) -> ("Value"=w2357:string)  [unwired: 1 in, 2 out]
                    n895 = call <vilib>:"Open Config Data.vi"("create file if necessary (T)"=FALSE, "configuration file path"=w2381) -> ("error out"=w2379:errorcluster, "refnum"=w2380:T4)  [unwired: 1 in, 7 out]
                    n896 = call-poly <vilib>:"Write Key.vi"("section"=w2357, "error in (no error)"=w2379, "value"=w2362, "key"="SN", "refnum"=w2380) -> ("error out"=w2369:errorcluster, "refnum out"=w2368:T4)  [unwired: 4 in, 1 out]
                    n897 = call <vilib>:"Close Config Data.vi"("error in (no error)"=w2369, "refnum"=w2368) -> ("error out"=w2367:errorcluster)  [unwired: 8 in, 1 out]
                    n898 = property on="Current SN" class="DigNum (strict)"("Value"=w2361) -> ()  [unwired: 2 in, 2 out]
                    n899 = property on="SetSN" class="Bool (strict)"(error in=w2367, "Value"=w2373) -> (error out=w2372:errorcluster)  [unwired: 1 in, 1 out]
                    n900 = property on="Automation" class="Bool (strict)"(error in=w2372, "Value"=w2373) -> (error out=w2371:errorcluster)  [unwired: 1 in, 1 out]
                    n901 = Increment(x=w2361) -> (x+1=w2370:i32)
                    n902 = property on="Next SN" class="DigNum (strict)"(error in=w2371, "Value"=w2370) -> (error out=w2366:errorcluster)  [unwired: 1 in, 1 out]
                  }
                }
              }
            }
            n903 = call <vilib>:"Clear Errors.vi"("error in (no error)"=w2315) -> ("error out"=w2308:errorcluster)  [unwired: 5 in, 1 out]
            n904 = property on="SetSN" class="Bool (strict)"(error in=w2308, "Value"=FALSE ("SetSN")) -> (error out=w2314:errorcluster)  [unwired: 1 in, 1 out]
            n905 = case shown="True" w2317 {
              tunnel: w2314 -> [_ _]
              frame False {
              }
              frame True {
                w2383 = TRUE ("Value (Signaling)")
                n906 = property on="Report" class="Bool (strict)"("Val(Sgnl)"=w2383, "Value"=w2383) -> ()  [unwired: 2 in, 2 out]
              }
            }
          }
          event "ATR": Mouse Enter {
            n907 = event-data() -> ()  [unwired: 1 in, 4 out]
            n908 = call-poly <vilib>:"Set Cursor.vi"("error in (no error)"=w2392, "icon"=u16 1) -> ("error out"=w2393:errorcluster)  [unwired: 8 in, 1 out]
          }
          event "ATR": Mouse Leave {
            n909 = event-data() -> ()  [unwired: 1 in, 4 out]
            n910 = call-poly <vilib>:"Set Cursor.vi"("error in (no error)"=w2404, "icon"=u16 0) -> ("error out"=w2402:errorcluster)  [unwired: 8 in, 1 out]
          }
          event "ATR": Mouse Down? {
            n911 = event-data() -> ("Coords"=w2421:T28)  [unwired: 1 in, 4 out]
            n912 = invoke on="ATR" class="Tbl (strict)" method="Point To Row Column"("Point"=w2421) -> ("InBounds"=w2417:bool, "CellPosition"=w2416:T14)  [unwired: 5 in, 4 out]
            n913 = Greater Than 0?(x=w2416) -> (x > 0?=w2420:cluster{"Row":bool, "Column":bool})
            n914 = Cluster To Array(cluster=w2420) -> (array=w2419:bool[])
            n915 = Or Array Elements(Boolean array=w2419) -> (logical OR=w2418:bool)
            n916 = Or(x=w2417, y=w2418) -> (x .or. y?=w2415:bool)
            n917 = event-data("Discard?"=w2415) -> ()  [unwired: 1 in, 1 out]
          }
          event Panel Close? {
            n918 = event-data() -> ("VIRef"=w2427:refnum<vi>)  [unwired: 1 in, 3 out]
            n919 = Close Reference(reference=w2427) -> ()  [unwired: 1 in, 1 out]
            n920 = disable-structure shown="Disabled" {
              frame Disabled {
                n921 = property on="Stop Button" class="Bool (strict)"("Val(Sgnl)"=TRUE ("Stop Button"), "Value"=FALSE ("Stop Button")) -> ()  [unwired: 2 in, 2 out]
              }
              frame Enabled {
              }
            }
            n922 = event-data("Discard?"=TRUE) -> ()  [unwired: 1 in, 1 out]
            "ClosePanel" <- TRUE ("ClosePanel")
          }
          event "Start": Value Change {
            w2438 = string[] []  # TestArray
            n923 = event-data() -> ()  [unwired: 1 in, 2 out]
            n924 = while {
              tunnel: [w2462] -> w2437
              tunnel: [w2461] -> w2449
              shift-right: [w2459] -> _
              shift-left: enum16{"Stop", "Tests", "Bit test", "Start"}."Start" -> [w2460]
              tunnel: w2438 -> [w2458]
              stop <- w2457 stop-if-true
              n925 = case shown="\"Tests\"" w2460 {
                tunnel: [w2467 w2472 w2482 w2493] -> w2462
                tunnel: [errorcluster {"status"=FALSE, "code"=0, "source"=""} ("error out") w2471 errorcluster {"status"=FALSE, "code"=0, "source"=""} ("error out") w2491] -> w2461
                tunnel: [w2466 w2478 enum16{"Stop", "Tests", "Bit test", "Start"}."Stop" w2487] -> w2459
                tunnel: w2458 -> [w2467 _ w2482 w2493]
                tunnel: [w2465 w2477 FALSE FALSE] -> w2457
                frame "Stop", Default {
                  n926 = flat-sequence {
                    tunnel: [enum16{"Stop", "Tests", "Bit test", "Start"}."Stop"] -> w2466
                    tunnel: [TRUE] -> w2465
                    frame #0 {
                    }
                  }
                  n927 = property on="Start" class="Bool (strict)"("Value"=FALSE ("Start")) -> ()  [unwired: 2 in, 2 out]
                }
                frame "Tests" {
                  w2476 = T13."Disabled and Grayed Out" ("Disabled")
                  n928 = property on="TestArray" class="Arr (strict)"() -> (error out=w2471:errorcluster, "Value"=w2473:string[])  [unwired: 2 in, 1 out]
                  n929 = call "Start Test Selection (SubVI).vi"("TestArrayIn"=w2473) -> ("AutoOut"=w2470:bool, "TestArrayOut"=w2472:string[])  [unwired: 9 in]
                  "Automation" <- w2470
                  n930 = property on="Start" class="Bool (strict)"("DisabledEnum"=w2476) -> ()  [unwired: 2 in, 2 out]
                  n931 = property on="Report" class="Bool (strict)"("DisabledEnum"=w2476) -> ()  [unwired: 2 in, 2 out]
                  n932 = control-ref of="ATR"() -> (w2474:refnum<vi>)
                  n933 = property on="Stop Button" class="Bool (strict)"("Value"=FALSE ("Stop Burn-in")) -> ()  [unwired: 2 in, 2 out]
                  n934 = case shown="True" w2470 {
                    tunnel: w2474 -> [_ w2479]
                    frame False {
                    }
                    frame True {
                      n935 = call "ResetTable Result (SubVI).vi"("Table in"=w2479) -> ()  [unwired: 11 in]
                    }
                  }
                  n936 = flat-sequence {
                    tunnel: [enum16{"Stop", "Tests", "Bit test", "Start"}."Tests"] -> w2478
                    tunnel: [TRUE] -> w2477
                    frame #0 {
                    }
                  }
                }
                frame "Bit test" {
                }
                frame "Start" {
                  n937 = property on="CAN Status" class="Bool (strict)"() -> (error out=w2490:errorcluster, "Value"=w2489:bool)  [unwired: 2 in, 1 out]
                  n938 = property on="Serial Status" class="Bool (strict)"(error in=w2490) -> ("Value"=w2488:bool)  [unwired: 1 in, 2 out]
                  n939 = And(x=w2489, y=w2488) -> (x .and. y?=w2486:bool)
                  n940 = case shown="True" w2486 {
                    tunnel: [w2495 w2500] -> w2491
                    tunnel: [enum16{"Stop", "Tests", "Bit test", "Start"}."Stop" enum16{"Stop", "Tests", "Bit test", "Start"}."Tests"] -> w2487
                    frame False {
                      n941 = call "Display Message to User5"() -> ("error out"=w2495:errorcluster)  [unwired: 10 in, 1 out]
                    }
                    frame True {
                      n942 = control-ref of="Motor Speed RPM Serial"() -> (w2497:refnum<vi>)
                      n943 = control-ref of="Stop Button"() -> (w2498:refnum<vi>)
                      n944 = control-ref of="Pannel User Message"() -> (w2499:refnum<vi>)
                      n945 = call "Write panel message Kinetics (SubVI).vi"(4:"rpm"=w2497, 5:"rpm"=FALSE ("rpm"), "PrintTime"=FALSE, "Stop"=w2498, "Time to wait"=0.0, "Strin"="TESTER BIT TEST OPERATION IN PROCESS\nPlease wait...", "String in"=w2499) -> ("error out"=w2500:errorcluster)  [unwired: 3 in, 1 out]
                    }
                  }
                }
              }
            }
            n946 = Array Size(array=w2437) -> (size(s)=w2436:i32)
            n947 = case shown="1, Default" w2436 {
              frame 0 {
              }
              frame 1, Default {
                n948 = local read "DAQmx Device Name"() -> (w2456:tag)
                n949 = call "Operation (SubVI).vi"("On/Off"=TRUE, "Operation"=T5."PowerSuply", "DAQmx Device Name"=w2456) -> ("error out"=w2453:errorcluster)  [unwired: 8 in]
                n950 = call "Time Delay"("error in (no error)"=w2453) -> ()  [unwired: 10 in, 1 out]
              }
            }
            n951 = Bundle By Name(cluster=T1 {"VISA"="COM1", "TestArray"=[]}, "VISA"=w2440, "TestArray"=w2437) -> (w2441:T1)
            n952 = Enqueue Element(queue=w2450, element=w2441, error in (no error)=w2449) -> (queue out=w2447:refnum<queue>, error out=w2448:errorcluster)  [unwired: 2 out]
          }
          event "Report", "Stop Button": Value Change {
            w2538 = T29 1 items=["User Home"=0, "User Desktop"=1, "User Documents"=2, "User Application Data"=3, "User Preferences"=4, "User Temporary"=5, "Public Documents"=6, "Public Application Data"=7, "Public Preferences"=8, "Public Cache"=13, "System Core Libraries"=9, "System Installed Libraries"=10, "Application Files"=11, "Boot Volume Root"=12] ("system directory type")
            w2505 = FALSE ("Report")
            n953 = event-data() -> ("CtlRef"=w2556:refnum<vi>)  [unwired: 1 in]
            n954 = call <vilib>:"Get System Directory.vi"("create directory if not found? (F)"=TRUE, "system directory type"=w2538) -> ("system directory"=w2537:path)  [unwired: 9 in]
            n955 = Build Path(base path=w2537, name or relative path="KineticsReports") -> (appended path=w2591:path)
            n956 = property on="CAN Status" class="Bool (strict)"() -> ("Value"=w2541:bool)  [unwired: 2 in, 2 out]
            n957 = property on="Serial Status" class="Bool (strict)"() -> ("Value"=w2542:bool)  [unwired: 2 in, 2 out]
            n958 = call <vilib>:"Check if File or Folder Exists.vi"("path"=w2591) -> ("error out"=w2589:errorcluster, "file or folder exists?"=w2592:bool, "dup path"=w2590:path)  [unwired: 8 in]
            n959 = And(x=w2542, y=w2541) -> (x .and. y?=w2543:bool)
            n960 = case shown="False" w2592 {
              tunnel: w2589 -> [w2648 w2649]
              tunnel: w2590 -> [w2647 w2650]
              tunnel: [w2646 w2650] -> w2540
              tunnel: [w2645 w2649] -> w2594
              frame False {
                n961 = Create Folder(path (use dialog)=w2647, error in=w2648) -> (created path=w2646:path, error out=w2645:errorcluster)  [unwired: 1 in, 1 out]
              }
              frame True {
              }
            }
            n962 = case shown="True" w2543 {
              tunnel: [w2599 "" ("read buffer")] -> w2578
              tunnel: [w2599 w2601] -> w2531
              tunnel: w2557 -> [_ w2609]
              tunnel: [w2599 w2618] -> w2534
              tunnel: [w2599 w2602] -> w2532
              tunnel: [w2599 "" ("read buffer")] -> w2550
              frame False {
                w2599 = "N_A" ("read buffer")
              }
              frame True {
                n963 = call "Serial.vi"("write buffer"="SN\r\n", "VISA resource name"=w2609) -> ("error out"=w2614:errorcluster, "read buffer"=w2616:string)  [unwired: 8 in]
                n964 = Decimal String To Number(string=w2616) -> (number=w2615:i32)  [unwired: 2 in, 1 out]
                n965 = Number To Decimal String(number=w2615, width (-)=i16 4) -> (decimal integer string=w2618:string)
                n966 = call "Serial.vi"("error in (no error)"=w2614, "write buffer"="VR\r\n", "VISA resource name"=w2609) -> ("error out"=w2610:errorcluster, "read buffer"=w2602:string)  [unwired: 7 in]
                n967 = call "Serial.vi"("error in (no error)"=w2610, "write buffer"="PN\r\n", "VISA resource name"=w2609) -> ("read buffer"=w2600:string)  [unwired: 7 in, 1 out]
                n968 = String Length(string=w2600) -> (length=w2607:i32)
                n969 = Subtract(x=6, y=w2607) -> (x-y=w2606:i32)
                n970 = for {
                  N: w2606 -> [_]
                  shift-right: [w2623] -> w2603
                  shift-left: "" -> [w2622]
                  n971 = Concatenate Strings(w2622, "0" ("string")) -> (w2623:string)
                }
                n972 = Concatenate Strings("RD" ("string"), w2603, w2600) -> (w2601:string)
              }
            }
            n973 = Get Date/Time String(want seconds? (F)=TRUE) -> (date string=w2593:string)  [unwired: 2 in, 1 out]
            n974 = call <vilib>:"Open Config Data.vi"("create file if necessary (T)"=FALSE, "configuration file path"=w2559) -> ("refnum"=w2569:T4)  [unwired: 1 in, 8 out]
            n975 = property on="Logger Path" class="Path"(error in=w2594, "Value"=w2540, "StartPath"=w2540) -> (error out=w2572:errorcluster)  [unwired: 1 in, 1 out]
            n976 = Search and Replace String(replace all?=TRUE ("replace all? (F)"), input string=w2593, search string="/") -> (result string=w2575:string)  [unwired: 5 in, 3 out]
            n977 = local read "UUT"() -> (w2512:string)
            n978 = call-poly <vilib>:"Read Key.vi"("section"=w2512, "key"="version", "refnum"=w2569) -> ("error out"=w2564:errorcluster, "value"=w2567:string, "refnum out"=w2566:T4)  [unwired: 5 in, 1 out]
            n979 = call-poly <vilib>:"Read Key.vi"("section"="Kinetics", "error in (no error)"=w2564, "key"="Tester Software Ver", "refnum"=w2566) -> ("error out"=w2562:errorcluster, "value"=w2533:string, "refnum out"=w2565:T4)  [unwired: 4 in, 1 out]
            n980 = property on="POWER Board S/N" class="Str"() -> ("Value"=w2510:string)  [unwired: 2 in, 2 out]
            n981 = Concatenate Strings("ATR" ("string"), w2578, w2534, "_", w2575, ".docx" ("string")) -> (w2573:string)
            n982 = call <vilib>:"Close Config Data.vi"("error in (no error)"=w2562, "refnum"=w2565) -> ()  [unwired: 8 in, 2 out]
            n983 = Build Path(base path=w2540, name or relative path=w2573) -> (appended path=w2574:path)
            n984 = property on="DSP Board S/N" class="Str"() -> ("Value"=w2509:string)  [unwired: 2 in, 2 out]
            n985 = Concatenate Strings("  Rev-" ("string"), w2567) -> (w2558:string)
            n986 = while {
              tunnel: w2573 -> [w2630]
              tunnel: w2540 -> [w2627]
              shift-right: [w2629] -> w2571
              shift-left: w2574 -> [w2628]
              shift-right: [w2625] -> w2560
              shift-left: w2561 -> [w2626]
              tunnel: w2572 -> [w2631]
              tunnel: [w2632] -> w2539
              stop <- w2624 continue-if-true
              n987 = call <vilib>:"Check if File or Folder Exists.vi"("error in (no error)"=w2631, "path"=w2628) -> ("error out"=w2632:errorcluster, "file or folder exists?"=w2624:bool)  [unwired: 7 in, 1 out]
              n988 = case shown="True" w2624 {
                tunnel: w2630 -> [_ w2644]
                tunnel: w2626 -> [_ w2636]
                tunnel: [w2634 w2641] -> w2629
                tunnel: w2628 -> [w2634 _]
                tunnel: w2627 -> [_ w2642]
                tunnel: [1 w2635] -> w2625
                frame False {
                }
                frame True {
                  w2637 = ".docx" ("search string")
                  n989 = Search and Replace String(input string=w2644, search string=w2637) -> (result string=w2643:string)  [unwired: 6 in, 3 out]
                  n990 = Number To Decimal String(number=w2636) -> (decimal integer string=w2639:string)  [unwired: 1 in]
                  n991 = call <vilib>:"Space Constant.vi"() -> ("String"=w2638:string)
                  n992 = Concatenate Strings(w2643, w2638, w2639, w2637) -> (w2640:string)
                  n993 = Build Path(base path=w2642, name or relative path=w2640) -> (appended path=w2641:path)
                  n994 = Increment(x=w2636) -> (x+1=w2635:i32)
                }
              }
            }
            n995 = property on="ParamVersion" class="Str"() -> ("Value"=w2508:string)  [unwired: 2 in, 2 out]
            n996 = call "HeaderBis.vi"("UUTHeader"=w2512, "POWER SN"=w2510, "Revision Param"=w2508, "P/N UUT"=w2531, "DSP SN"=w2509, "Driver S/N"=w2534, "VR"=w2532, "Oper."=w2535, "Tester Software Ver"=w2533) -> ("table header"=w2530:string, "Array"=w2529:string[][])  [unwired: 4 in, 1 out]
            n997 = Open/Create/Replace File(file path (use dialog)=w2571, error in=w2539, operation (0:open)=T17."create") -> (error out=w2584:errorcluster)  [unwired: 3 in, 2 out]
            n998 = control-ref of="ATR"() -> (w2596:refnum<vi>)
            n999 = property class="Tbl (strict)"(reference=w2596, error in=w2584) -> ("Value"=w2597:string[][])  [unwired: 2 out]
            n1000 = control-ref of="ATR"() -> (w2522:refnum<vi>)
            n1001 = call "PassFailUUT (SubVI).vi"("Table in"=w2522) -> ("PassFaileUUTresult"=w2515:bool)  [unwired: 8 in, 2 out]
            n1002 = property on="Test Failed" class="Bool (strict)"("Value"=w2515) -> ()  [unwired: 2 in, 2 out]
            n1003 = call "MarvinReport.vi"("HEADER1"=w2530, "ATR Or"=w2596, "Steps   pfull"=w2597, "Footer UUT"=w2550, "pageNum"=3, "InputHeaderArray"=w2529, "FILE NAME"=w2573, "Report Folder"=w2571, "REV"=w2558, "Test-Conductor"=w2535) -> ("error out"=w2545:errorcluster)  [unwired: 4 in, 1 out]
            n1004 = Select(t="PASS" ("name or relative path"), s=w2515, f="FAIL" ("name or relative path")) -> (s? t:f=w2514:string)
            n1005 = call <vilib>:"Clear Errors.vi"("error in (no error)"=w2545) -> ("error out"=w2544:errorcluster)  [unwired: 5 in, 1 out]
            n1006 = property class="Bool (strict)"(reference=w2556, error in=w2544) -> ("BoolText.Text"=w2555:string)  [unwired: 2 out]
            n1007 = Equal?(x=w2555, y="Report") -> (x = y?=w2549:bool)
            n1008 = Select(t=T3."MainProgram", s=w2549, f=T3."MainProgram") -> (s? t:f=w2552:T3)
            n1009 = call <vilib>:"Application Directory.vi"() -> ("Application Directory"=w2518:path)
            n1010 = Build Path(base path=w2518, name or relative path="data\\TestResult.ini") -> (appended path=w2521:path)
            n1011 = Select(t="Save Report...", s=w2549, f="Program Stopped...\r\nPlease turn OFF All Power sinks") -> (s? t:f=w2547:string)
            n1012 = property on="Report" class="Bool (strict)"(error in=w2544, "Value"=w2505) -> (error out=w2506:errorcluster)  [unwired: 1 in, 1 out]
            n1013 = call <vilib>:"Open Config Data.vi"("configuration file path"=w2521) -> ("error out"=w2519:errorcluster, "refnum"=w2520:T4)  [unwired: 2 in, 7 out]
            n1014 = property on="Stop Button" class="Bool (strict)"(error in=w2506, "Value"=w2505) -> ()  [unwired: 1 in, 2 out]
            n1015 = property on="Pannel User Message" class="Str"("Value"=w2547) -> ()  [unwired: 2 in, 2 out]
            n1016 = call-poly <vilib>:"Write Key.vi"("section"="Kinetics", "error in (no error)"=w2519, "value"=w2514, "key"="Result", "refnum"=w2520) -> ("error out"=w2517:errorcluster, "refnum out"=w2516:T4)  [unwired: 4 in, 1 out]
            n1017 = call <vilib>:"Close Config Data.vi"("error in (no error)"=w2517, "refnum"=w2516) -> ()  [unwired: 8 in, 2 out]
          }
          event "Help Button": Value Change {
            n1018 = event-data() -> ()  [unwired: 1 in, 6 out]
            n1019 = vi-ref "Help.vi"() -> (w2664:refnum<vi>)
            n1020 = invoke class="VI" method="FP.Open"(reference=w2664, error in=w2662, "Activate"=TRUE ("Activate?"), "State"=T15."Standard") -> (error out=w2663:errorcluster)  [unwired: 1 in, 4 out]
            n1021 = call "Help.vi"("error in"=w2663, "TesterSWVersion"=w2654) -> ("error out"=w2661:errorcluster)  [unwired: 6 in]
            n1022 = property on="Help Button" class="Bool (strict)"("Value"=FALSE ("Help Button")) -> ()  [unwired: 2 in, 2 out]
          }
          event "Serial Com": Value Change {
            n1023 = event-data() -> ()  [unwired: 1 in, 6 out]
            n1024 = property on="Serial Com" class="Bool"(error in=w2675, "Visible"=FALSE) -> (error out=w2679:errorcluster)  [unwired: 1 in, 1 out]
            n1025 = property on="VISA Kinetics" class="VISAName"(error in=w2679, "Visible"=TRUE) -> (error out=w2676:errorcluster)  [unwired: 1 in, 1 out]
          }
          event "VISA Kinetics": Value Change {
            n1026 = event-data() -> ()  [unwired: 1 in, 6 out]
            n1027 = property on="Serial Com" class="Bool"(error in=w2683, "Visible"=FALSE) -> ()  [unwired: 1 in, 2 out]
            n1028 = property on="Pannel User Message" class="Str"(error in=w2683, "Value"="Serial connection in process" ("Pannel User Message")) -> ()  [unwired: 1 in, 2 out]
          }
          event "Refresh Button": Value Change {
            n1029 = event-data() -> ()  [unwired: 1 in, 6 out]
          }
          event "Settings": Value Change {
            n1030 = event-data() -> ()  [unwired: 1 in, 6 out]
          }
        }
      }
      frame "Initialize" {
        w2727 = 0
        w2729 = FALSE ("Visible")
        w2731 = FALSE ("Visible")
        w2737 = refnum<visa-resource-name> "COMx" ("VISA resource name")
        w2708 = FALSE ("Serial Status")
        n1031 = property on="EventTimeout" class="DigNum (strict)"(error in=errorcluster {"status"=FALSE, "code"=0, "source"=""} ("error out"), "Value"=100 ("EventTimeout")) -> (error out=w2711:errorcluster)  [unwired: 1 in, 1 out]
        n1032 = property on="ComTestResult" class="Bool (strict)"("Value"=w2731) -> ()  [unwired: 2 in, 2 out]
        n1033 = property on="VenableResult" class="Bool (strict)"("Value"=w2731) -> ()  [unwired: 2 in, 2 out]
        n1034 = property on="VenableDirectionResult" class="Bool (strict)"("Value"=w2731) -> ()  [unwired: 2 in, 2 out]
        n1035 = property on="Serial Com" class="Bool"(error in=w2711, "Visible"=FALSE) -> (error out=w2739:errorcluster)  [unwired: 1 in, 1 out]
        n1036 = property on="VisualInspectionResult" class="Bool (strict)"("Value"=FALSE ("Visible")) -> ()  [unwired: 2 in, 2 out]
        n1037 = property on="VISA Kinetics" class="VISAName"(error in=w2739, "Visible"=FALSE, "Value"=w2737) -> (error out=w2720:errorcluster)  [unwired: 1 in, 1 out]
        n1038 = property on="Analogtest" class="Bool (strict)"("Value"=w2708) -> ()  [unwired: 2 in, 2 out]
        n1039 = property on="Serial Status" class="Bool (strict)"("Value"=w2708) -> ()  [unwired: 2 in, 2 out]
        n1040 = property on="Refresh Button" class="Bool (strict)"(error in=w2720, "Value"=FALSE ("Refresh Button")) -> (error out=w2721:errorcluster)  [unwired: 1 in, 1 out]
        n1041 = property on="MotorTempResult" class="Bool (strict)"("Value"=w2729) -> ()  [unwired: 2 in, 2 out]
        n1042 = property on="Automation" class="Bool (strict)"("Value"=w2729) -> ()  [unwired: 2 in, 2 out]
        n1043 = call "Find DAQ Devices.vi"("Error In"=w2721) -> ("Error Out"=w2724:errorcluster, "DAQmx Device Name"=w2712:tag)  [unwired: 9 in]
        "DAQmx Device Name" <- w2712
        n1044 = call <vilib>:"Clear Errors.vi"("error in (no error)"=w2724) -> ("error out"=w2723:errorcluster)  [unwired: 5 in, 1 out]
        n1045 = Not Equal?(x=w2712, y=tag "") -> (x != y?=w2725:bool)
        n1046 = case shown="True" w2725 {
          tunnel: w2712 -> [_ w2745]
          tunnel: w2723 -> [w2741 w2744]
          tunnel: [w2741 w2743] -> w2719
          frame False {
          }
          frame True {
            n1047 = call "Operation (SubVI).vi"("error in (no error)"=w2744, "Operation"=T5."Init", "DAQmx Device Name"=w2745) -> ("error out"=w2743:errorcluster)  [unwired: 8 in]
          }
        }
        n1048 = call "Operation (SubVI).vi"("error in (no error)"=w2719, "On/Off"=TRUE, "Operation"=T5."0 ohm", "DAQmx Device Name"=w2712) -> ("error out"=w2714:errorcluster)  [unwired: 7 in]
        n1049 = call "Operation (SubVI).vi"("error in (no error)"=w2714, "On/Off"=TRUE, "Operation"=T5."PowerSuply", "DAQmx Device Name"=w2712) -> ("error out"=w2713:errorcluster)  [unwired: 7 in]
        "Test Failed" <- w2708
      }
    }
  }
  n1050 = call "ATRBuild.vi"() -> ()  [unwired: 9 in, 3 out]
  n1051 = disable-structure shown="Disabled" {
    frame Disabled {
      n1052 = case shown="\"BLDC 30A\", Default" {
        selector: _ -> [_ _ _ _ _]
        tunnel: [26 26 26 26 35] -> _
        frame "BLDC 30A", Default {
        }
        frame "Warrior 60A" {
        }
        frame "Condenser Merkava" {
        }
        frame "Condenser India" {
        }
        frame "BLDC 60A" {
        }
      }
    }
    frame Enabled {
    }
  }
  n1053 = disable-structure shown="Disabled" {
    frame Disabled {
      n1054 = control-ref of="Stop Button"() -> ()  [unwired: 1 out]
      n1055 = control-ref of="UUT"() -> ()  [unwired: 1 out]
      n1056 = property on="UUT" class="Str" props=["Value"]() -> ()  [unwired: 2 in, 3 out]
      n1057 = control-ref of="UUT"() -> ()  [unwired: 1 out]
      n1058 = property on="UUT" class="DigNum (strict)" props=["Value"]() -> ()  [unwired: 2 in, 3 out]
      n1059 = control-ref of="Motor Speed RPM Serial"() -> ()  [unwired: 1 out]
      n1060 = call "Find_Number_LineMARVIN.vi"() -> ()  [unwired: 5 in, 4 out]
      n1061 = control-ref of="Pannel User Message"() -> ()  [unwired: 1 out]
      n1062 = call "Write panel message Kinetics (SubVI).vi"() -> ()  [unwired: 10 in, 2 out]
      n1063 = local read "DAQmx Device Name"() -> (w2752:tag)
      n1064 = control-ref of="ATR"() -> ()  [unwired: 1 out]
      n1065 = call "PassOrFail (SubVI).vi"() -> ()  [unwired: 11 in, 1 out]
      n1066 = call "Serial.vi"("write buffer"="EP=1\r\nVC=1000\r\n") -> ()  [unwired: 9 in, 2 out]
      n1067 = call "Operation (SubVI).vi"("DAQmx Device Name"=w2752) -> ()  [unwired: 10 in, 1 out]
      n1068 = property on="UUT" class="Str" props=["Value"]() -> ()  [unwired: 2 in, 3 out]
    }
    frame Enabled {
    }
  }
  n1069 = disable-structure shown="Disabled" {
    frame Disabled {
      w2753 = T13."Disabled and Grayed Out" ("Disabled")
      w2754 = FALSE ("Start")
      n1070 = property on="Current SN" class="DigNum (strict)" props=["Value"]() -> ()  [unwired: 2 in, 3 out]
      n1071 = property on="UUT" class="DigNum (strict)" props=["Value"]() -> ()  [unwired: 2 in, 3 out]
      n1072 = property on="Serial Status" class="Bool (strict)" props=["Value"]() -> ()  [unwired: 2 in, 3 out]
      n1073 = property on="UUT SoftwareVer" class="Str" props=["Value"]() -> ()  [unwired: 2 in, 3 out]
      n1074 = call "Operation (SubVI).vi"() -> ()  [unwired: 11 in, 1 out]
      n1075 = property on="Next SN" class="DigNum (strict)" props=["Value"]() -> ()  [unwired: 3 in, 2 out]
      n1076 = property on="Start" class="Bool (strict)"("Value"=w2754, "DisabledEnum"=w2753) -> ()  [unwired: 2 in, 2 out]
      n1077 = property on="Report" class="Bool (strict)"("Value"=w2754, "DisabledEnum"=w2753) -> ()  [unwired: 2 in, 2 out]
    }
    frame Enabled {
    }
  }
  "Pannel User Message" <- w17
